vi "Text control 2 v7.2_pump-specific.vi"() -> ()   [LabVIEW 2019]
panel:
  in  "Tab Control":enum32{"Main", "Other parameters"}(tab)
  out "Vp vs time (FPP Bias Stress)":cluster{"Y data in":dbl[], "X data in":dbl[]}[](graph)
  out "Line running":i32
  out "Total lines":i32
  out "Path":path=path "C:/users/rlp38/09Apr2009LTtesting/test2.txt"
  out "I vs Vg":cluster{"Y data in":dbl[], "X data in":dbl[]}[](graph)
  out "Is max":dbl format="%.2e"
  out "Id max":dbl format="%.2e"
  out "Ig max":dbl format="%.2e"
  out "Imax vs time":cluster{"Y data in":dbl[], "X data in":dbl[]}[](graph)
  out "Imin vs time":cluster{"Y data in":dbl[], "X data in":dbl[]}[](graph)
  out "I vs Vd":cluster{"Y data in":dbl[], "X data in":dbl[]}[](graph)
  in  "Script":string="#-------------------------------------------------------\n# SPM pump cleaning script x 10\n#\n# Version: 0.5\n# Author: Dimitrios Simatos\n# Last updated: 2020-09-03\n#-------------------------------------------------------\n# Description\n#\n# This script is designed to run the cleaning sequence of the SPM OEM pump ten times.\n#-------------------------------------------------------\n# Changes\n#\n# Placed initialization and hard stop commands in the beginning.\n#-------------------------------------------------------\n# Important points\n#\n# Never leave any liquid in the pump to dry after the experiments. If they dry, the residue may block the valve.\n# Always run the cleaning cycle after the experiments.\n# Use clockwise rotation when going up in valve port numbers and vice versa.\n#-------------------------------------------------------\n# Things to do before running the script\n#\n# Remove all reservoirs, except the one in Port 3.\n# Set filenames.\n# Replace the tubing, if necessary.\n#-------------------------------------------------------\n# Port connections\n#\n# Port 1: Waste\n# Port 2: Waste\n# Port 3: Various cleaning liquids\n# Port 4: Waste\n# Port 5: Waste\n# Port 6: Waste\n#\n# Between each of the 4 runs, the settings of Port 3 will change, according to the cleaning protocol.\n# The settings for Port 3 are:\n# 1st run: 1% v/v solution of sodium hypochlorite in ultrapure water\n# 2nd run: 0.1% w/v solution of sodium dodecyl sulfate in ultrapure water\n# 3rd run: Ultrapure water\n# 4th run: Waste (in air, not immersed in liquid)\n#-------------------------------------------------------\n# Cleaning protocol for the SPM OEM pump (from the manual)\n#\n# A cleaning procedure should be performed at the end of each day or in between two different experiments.\n# An effective cleaning can be performed in the following manner:\n# • Bleach solution to kill microorganisms\n# 1. Prepare a solution of 1% chlorine bleach and deionized water\n#    NOTE: Prepare a 1% v/v solution of sodium hypochlorite in deionized water\n# 2. Prepare a reservoir and place 1 tubing in the bleach solution and 5 tubings in a waste recipient\n# 3. Pick up the bleach solution through 1 port to entirely fill the syringe\n# 4. Sequentially output the syringe content through the remaining ports and throw it to the waste\n# 5. Repeat operation at least 2 times\n# • Detergent solution to remove debris\n# 1. Prepare a solution of 0.1% detergent and deionized water\n#    NOTE: Prepare a 0.1% w/v solution of sodium dodecyl sulfate in deionized water\n# 2. Move the tubing from the bleach solution reservoir and place it into a reservoir of detergent solution\n# 3. Pick up the detergent solution through 1 port to entirely fill the syringe\n# 4. Sequentially output the detergent solution through the remaining ports into the waste recipient\n# 5. Repeat operation at least 2 times\n# • Rinsing water to prepare the pump for your next experiment\n# 1. Move the tubing from the detergent solution reservoir and place it into a reservoir of deionized water\n# 2. Pick up the rinsing solution through 1 port to entirely fill the syringe\n# 3. Sequentially output the rinse water through the remaining ports into the waste recipient\n# 4. Repeat operation at least 2 times\n# • Replace the tubing, if necessary\n#-------------------------------------------------------\n# Pumping cycles and execution time\n#\n# Execution time for a single cycle: 6 x (1 min + 10 sec) = 7 minutes\n# Total execution time: 4 x 7 = 28 minutes\n# Since the script has to run 4 times, the cleaning lasts for: 4 x 28 = 112 minutes\n# Air must be the last to be pumped through the valve, to remove all liquids.\n# There are 4 pumping cycles. Each one draws a different liquid through port 3 and pumps it sequentially through ports 1,2,4,5,6.\n# During the sequential pumping, each port receives 200 ul of liquid (20% of the total syringe volume = 600 \"plunger units\")\n# The device must be disconnected from the port during the cleaning procedure.\n# All cycles are similar, except cycle 1 has the initialization command uncommented and the first report valve command commented.\n#-------------------------------------------------------\n# Volume of liquid needed\n#\n# Volume of liquid needed per cycle: 1 ml\n# Total volume of liquid needed per script run: 4 x 1 = 4 ml\n# Since the script has to run 4 times, the first 3 with different liquids, I need:\n# 4 ml of 1% v/v solution of sodium hypochlorite in ultrapure water\n# 4 ml of 0.1% w/v solution of sodium dodecyl sulfate in ultrapure water\n# 4 ml of ultrapure water\n#-------------------------------------------------------\n# Parameters\n#\n# Syringe size: 1 ml\n# Step resolution N = 0.01 mm\n# Drawing flow V = 300 pulses/second (6000 ul/min)\n# Pumping flow V = 300 pulses/second (6000 ul/min)\n#-------------------------------------------------------\n# Pump initialization\npump /1T #hard stop pump\npump /1ZR #initialize pump\n#-------------------------------------------------------\n# Cycle 1\n# Fill the syringe\npump /1Q #query pump\npump /1? #report absolute plunger position\n#pump /1?6 #report valve position\nwait-min 1 #wait 1 minute\npump /1N0R #set step resolution: 0.01 mm\npump /1Q #query pump\npump /1? #report absolute plunger position (the plunger should be at 0)\npump /1?6 #report valve position\nwait 1000 #wait 1 second\npump /1V300R #choose speed: 300 steps/s (6000 ul/min)\npump /1Q #query pump\nwait 1000 #wait 1 second\npump /1I3R #go to port 3, clockwise rotation\npump /1Q #query pump\npump /1?6 #report valve position\nwait 1000 #wait 1 second\npump /1A3000R #go to absolute position 3000 (= draw 1 ml)\nwait 30000 #wait 30 seconds\npump /1Q #query pump\npump /1? #report absolute plunger position (the plunger should have finished moving)\n#pump /1?6 #report valve position\n# The sequential pumping begins\n# Port 1\npump /1O1R #switch to port 1, counterclockwise rotation\npump /1Q #query pump\npump /1?6 #report valve position\npump /1A2400R #go to absolute position 2400 (= pump 200 ul)\npump /1Q #query pump\npump /1? #report absolute plunger position (the plunger should be moving to 0)\nwait-min 1 #wait 1 minute\npump /1? #report absolute plunger position (the plunger should have finished moving)\n# Port 2\npump /1I2R #switch to port 2, clockwise rotation\npump /1Q #query pump\npump /1?6 #report valve position\npump /1A1800R #go to absolute position 1800 (= pump 200 ul)\npump /1Q #query pump\npump /1? #report absolute plunger position (the plunger should be moving to 0)\nwait-min 1 #wait 1 minute\npump /1? #report absolute plunger position (the plunger should have finished moving)\n# Port 4\npump /1I4R #switch to port 4, clockwise rotation\npump /1Q #query pump\npump /1?6 #report valve position\npump /1A1200R #go to absolute position 1200 (= pump 200 ul)\npump /1Q #query pump\npump /1? #report absolute plunger position (the plunger should be moving to 0)\nwait-min 1 #wait 1 minute\npump /1? #report absolute plunger position (the plunger should have finished moving)\n# Port 5\npump /1I5R #switch to port 5, clockwise rotation\npump /1Q #query pump\npump /1?6 #report valve position\npump /1A600R #go to absolute position 600 (= pump 200 ul)\npump /1Q #query pump\npump /1? #report absolute plunger position (the plunger should be moving to 0)\nwait-min 1 #wait 1 minute\npump /1? #report absolute plunger position (the plunger should have finished moving)\n# Port 6\npump /1I6R #switch to port 6, clockwise rotation\npump /1Q #query pump\npump /1?6 #report valve position\npump /1A0R #go to absolute position 0 (= pump 200 ul)\npump /1Q #query pump\npump /1? #report absolute plunger position (the plunger should be moving to 0)\nwait-min 1 #wait 1 minute\npump /1? #report absolute plunger position (the plunger should have finished moving)\n#-------------------------------------------------------\n# Cycle 2\n# Fill the syringe\n#pump /1ZR #initialize pump\npump /1Q #query pump\npump /1? #report absolute plunger position\npump /1?6 #report valve position\nwait-min 1 #wait 1 minute\npump /1N0R #set step resolution: 0.01 mm\npump /1Q #query pump\npump /1? #report absolute plunger position (the plunger should be at 0)\npump /1?6 #report valve position\nwait 1000 #wait 1 second\npump /1V300R #choose speed: 300 steps/s (6000 ul/min)\npump /1Q #query pump\nwait 1000 #wait 1 second\npump /1O3R #go to port 3, counterclockwise rotation\npump /1Q #query pump\npump /1?6 #report valve position\nwait 1000 #wait 1 second\npump /1A3000R #go to absolute position 3000 (= draw 1 ml)\nwait 30000 #wait 30 seconds\npump /1Q #query pump\npump /1? #report absolute plunger position (the plunger should have finished moving)\n#pump /1?6 #report valve position\n# The sequential pumping begins\n# Port 1\npump /1O1R #switch to port 1, counterclockwise rotation\npump /1Q #query pump\npump /1?6 #report valve position\npump /1A2400R #go to absolute position 2400 (= pump 200 ul)\npump /1Q #query pump\npump /1? #report absolute plunger position (the plunger should be moving to 0)\nwait-min 1 #wait 1 minute\npump /1? #report absolute plunger position (the plunger should have finished moving)\n# Port 2\npump /1I2R #switch to port 2, clockwise rotation\npump /1Q #query pump\npump /1?6 #report valve position\npump /1A1800R #go to absolute position 1800 (= pump 200 ul)\npump /1Q #query pump\npump /1? #report absolute plunger position (the plunger should be moving to 0)\nwait-min 1 #wait 1 minute\npump /1? #report absolute plunger position (the plunger should have finished moving)\n# Port 4\npump /1I4R #switch to port 4, clockwise rotation\npump /1Q #query pump\npump /1?6 #report valve position\npump /1A1200R #go to absolute position 1200 (= pump 200 ul)\npump /1Q #query pump\npump /1? #report absolute plunger position (the plunger should be moving to 0)\nwait-min 1 #wait 1 minute\npump /1? #report absolute plunger position (the plunger should have finished moving)\n# Port 5\npump /1I5R #switch to port 5, clockwise rotation\npump /1Q #query pump\npump /1?6 #report valve position\npump /1A600R #go to absolute position 600 (= pump 200 ul)\npump /1Q #query pump\npump /1? #report absolute plunger position (the plunger should be moving to 0)\nwait-min 1 #wait 1 minute\npump /1? #report absolute plunger position (the plunger should have finished moving)\n# Port 6\npump /1I6R #switch to port 6, clockwise rotation\npump /1Q #query pump\npump /1?6 #report valve position\npump /1A0R #go to absolute position 0 (= pump 200 ul)\npump /1Q #query pump\npump /1? #report absolute plunger position (the plunger should be moving to 0)\nwait-min 1 #wait 1 minute\npump /1? #report absolute plunger position (the plunger should have finished moving)\n#-------------------------------------------------------\n# Cycle 3\n# Fill the syringe\n#pump /1ZR #initialize pump\npump /1Q #query pump\npump /1? #report absolute plunger position\npump /1?6 #report valve position\nwait-min 1 #wait 1 minute\npump /1N0R #set step resolution: 0.01 mm\npump /1Q #query pump\npump /1? #report absolute plunger position (the plunger should be at 0)\npump /1?6 #report valve position\nwait 1000 #wait 1 second\npump /1V300R #choose speed: 300 steps/s (6000 ul/min)\npump /1Q #query pump\nwait 1000 #wait 1 second\npump /1O3R #go to port 3, counterclockwise rotation\npump /1Q #query pump\npump /1?6 #report valve position\nwait 1000 #wait 1 second\npump /1A3000R #go to absolute position 3000 (= draw 1 ml)\nwait 30000 #wait 30 seconds\npump /1Q #query pump\npump /1? #report absolute plunger position (the plunger should have finished moving)\n#pump /1?6 #report valve position\n# The sequential pumping begins\n# Port 1\npump /1O1R #switch to port 1, counterclockwise rotation\npump /1Q #query pump\npump /1?6 #report valve position\npump /1A2400R #go to absolute position 2400 (= pump 200 ul)\npump /1Q #query pump\npump /1? #report absolute plunger position (the plunger should be moving to 0)\nwait-min 1 #wait 1 minute\npump /1? #report absolute plunger position (the plunger should have finished moving)\n# Port 2\npump /1I2R #switch to port 2, clockwise rotation\npump /1Q #query pump\npump /1?6 #report valve position\npump /1A1800R #go to absolute position 1800 (= pump 200 ul)\npump /1Q #query pump\npump /1? #report absolute plunger position (the plunger should be moving to 0)\nwait-min 1 #wait 1 minute\npump /1? #report absolute plunger position (the plunger should have finished moving)\n# Port 4\npump /1I4R #switch to port 4, clockwise rotation\npump /1Q #query pump\npump /1?6 #report valve position\npump /1A1200R #go to absolute position 1200 (= pump 200 ul)\npump /1Q #query pump\npump /1? #report absolute plunger position (the plunger should be moving to 0)\nwait-min 1 #wait 1 minute\npump /1? #report absolute plunger position (the plunger should have finished moving)\n# Port 5\npump /1I5R #switch to port 5, clockwise rotation\npump /1Q #query pump\npump /1?6 #report valve position\npump /1A600R #go to absolute position 600 (= pump 200 ul)\npump /1Q #query pump\npump /1? #report absolute plunger position (the plunger should be moving to 0)\nwait-min 1 #wait 1 minute\npump /1? #report absolute plunger position (the plunger should have finished moving)\n# Port 6\npump /1I6R #switch to port 6, clockwise rotation\npump /1Q #query pump\npump /1?6 #report valve position\npump /1A0R #go to absolute position 0 (= pump 200 ul)\npump /1Q #query pump\npump /1? #report absolute plunger position (the plunger should be moving to 0)\nwait-min 1 #wait 1 minute\npump /1? #report absolute plunger position (the plunger should have finished moving)\n#-------------------------------------------------------\n# Cycle 4\n# Fill the syringe\n#pump /1ZR #initialize pump\npump /1Q #query pump\npump /1? #report absolute plunger position\npump /1?6 #report valve position\nwait-min 1 #wait 1 minute\npump /1N0R #set step resolution: 0.01 mm\npump /1Q #query pump\npump /1? #report absolute plunger position (the plunger should be at 0)\npump /1?6 #report valve position\nwait 1000 #wait 1 second\npump /1V300R #choose speed: 300 steps/s (6000 ul/min)\npump /1Q #query pump\nwait 1000 #wait 1 second\npump /1O3R #go to port 3, counterclockwise rotation\npump /1Q #query pump\npump /1?6 #report valve position\nwait 1000 #wait 1 second\npump /1A3000R #go to absolute position 3000 (= draw 1 ml)\nwait 30000 #wait 30 seconds\npump /1Q #query pump\npump /1? #report absolute plunger position (the plunger should have finished moving)\n#pump /1?6 #report valve position\n# The sequential pumping begins\n# Port 1\npump /1O1R #switch to port 1, counterclockwise rotation\npump /1Q #query pump\npump /1?6 #report valve position\npump /1A2400R #go to absolute position 2400 (= pump 200 ul)\npump /1Q #query pump\npump /1? #report absolute plunger position (the plunger should be moving to 0)\nwait-min 1 #wait 1 minute\npump /1? #report absolute plunger position (the plunger should have finished moving)\n# Port 2\npump /1I2R #switch to port 2, clockwise rotation\npump /1Q #query pump\npump /1?6 #report valve position\npump /1A1800R #go to absolute position 1800 (= pump 200 ul)\npump /1Q #query pump\npump /1? #report absolute plunger position (the plunger should be moving to 0)\nwait-min 1 #wait 1 minute\npump /1? #report absolute plunger position (the plunger should have finished moving)\n# Port 4\npump /1I4R #switch to port 4, clockwise rotation\npump /1Q #query pump\npump /1?6 #report valve position\npump /1A1200R #go to absolute position 1200 (= pump 200 ul)\npump /1Q #query pump\npump /1? #report absolute plunger position (the plunger should be moving to 0)\nwait-min 1 #wait 1 minute\npump /1? #report absolute plunger position (the plunger should have finished moving)\n# Port 5\npump /1I5R #switch to port 5, clockwise rotation\npump /1Q #query pump\npump /1?6 #report valve position\npump /1A600R #go to absolute position 600 (= pump 200 ul)\npump /1Q #query pump\npump /1? #report absolute plunger position (the plunger should be moving to 0)\nwait-min 1 #wait 1 minute\npump /1? #report absolute plunger position (the plunger should have finished moving)\n# Port 6\npump /1I6R #switch to port 6, clockwise rotation\npump /1Q #query pump\npump /1?6 #report valve position\npump /1A0R #go to absolute position 0 (= pump 200 ul)\npump /1Q #query pump\npump /1? #report absolute plunger position (the plunger should be moving to 0)\nwait-min 1 #wait 1 minute\npump /1? #report absolute plunger position (the plunger should have finished moving)\n#-------------------------------------------------------\n# Cycle 5\n# Fill the syringe\npump /1Q #query pump\npump /1? #report absolute plunger position\n#pump /1?6 #report valve position\nwait-min 1 #wait 1 minute\npump /1N0R #set step resolution: 0.01 mm\npump /1Q #query pump\npump /1? #report absolute plunger position (the plunger should be at 0)\npump /1?6 #report valve position\nwait 1000 #wait 1 second\npump /1V300R #choose speed: 300 steps/s (6000 ul/min)\npump /1Q #query pump\nwait 1000 #wait 1 second\npump /1I3R #go to port 3, clockwise rotation\npump /1Q #query pump\npump /1?6 #report valve position\nwait 1000 #wait 1 second\npump /1A3000R #go to absolute position 3000 (= draw 1 ml)\nwait 30000 #wait 30 seconds\npump /1Q #query pump\npump /1? #report absolute plunger position (the plunger should have finished moving)\n#pump /1?6 #report valve position\n# The sequential pumping begins\n# Port 1\npump /1O1R #switch to port 1, counterclockwise rotation\npump /1Q #query pump\npump /1?6 #report valve position\npump /1A2400R #go to absolute position 2400 (= pump 200 ul)\npump /1Q #query pump\npump /1? #report absolute plunger position (the plunger should be moving to 0)\nwait-min 1 #wait 1 minute\npump /1? #report absolute plunger position (the plunger should have finished moving)\n# Port 2\npump /1I2R #switch to port 2, clockwise rotation\npump /1Q #query pump\npump /1?6 #report valve position\npump /1A1800R #go to absolute position 1800 (= pump 200 ul)\npump /1Q #query pump\npump /1? #report absolute plunger position (the plunger should be moving to 0)\nwait-min 1 #wait 1 minute\npump /1? #report absolute plunger position (the plunger should have finished moving)\n# Port 4\npump /1I4R #switch to port 4, clockwise rotation\npump /1Q #query pump\npump /1?6 #report valve position\npump /1A1200R #go to absolute position 1200 (= pump 200 ul)\npump /1Q #query pump\npump /1? #report absolute plunger position (the plunger should be moving to 0)\nwait-min 1 #wait 1 minute\npump /1? #report absolute plunger position (the plunger should have finished moving)\n# Port 5\npump /1I5R #switch to port 5, clockwise rotation\npump /1Q #query pump\npump /1?6 #report valve position\npump /1A600R #go to absolute position 600 (= pump 200 ul)\npump /1Q #query pump\npump /1? #report absolute plunger position (the plunger should be moving to 0)\nwait-min 1 #wait 1 minute\npump /1? #report absolute plunger position (the plunger should have finished moving)\n# Port 6\npump /1I6R #switch to port 6, clockwise rotation\npump /1Q #query pump\npump /1?6 #report valve position\npump /1A0R #go to absolute position 0 (= pump 200 ul)\npump /1Q #query pump\npump /1? #report absolute plunger position (the plunger should be moving to 0)\nwait-min 1 #wait 1 minute\npump /1? #report absolute plunger position (the plunger should have finished moving)\n#-------------------------------------------------------\n# Cycle 6\n# Fill the syringe\n#pump /1ZR #initialize pump\npump /1Q #query pump\npump /1? #report absolute plunger position\npump /1?6 #report valve position\nwait-min 1 #wait 1 minute\npump /1N0R #set step resolution: 0.01 mm\npump /1Q #query pump\npump /1? #report absolute plunger position (the plunger should be at 0)\npump /1?6 #report valve position\nwait 1000 #wait 1 second\npump /1V300R #choose speed: 300 steps/s (6000 ul/min)\npump /1Q #query pump\nwait 1000 #wait 1 second\npump /1O3R #go to port 3, counterclockwise rotation\npump /1Q #query pump\npump /1?6 #report valve position\nwait 1000 #wait 1 second\npump /1A3000R #go to absolute position 3000 (= draw 1 ml)\nwait 30000 #wait 30 seconds\npump /1Q #query pump\npump /1? #report absolute plunger position (the plunger should have finished moving)\n#pump /1?6 #report valve position\n# The sequential pumping begins\n# Port 1\npump /1O1R #switch to port 1, counterclockwise rotation\npump /1Q #query pump\npump /1?6 #report valve position\npump /1A2400R #go to absolute position 2400 (= pump 200 ul)\npump /1Q #query pump\npump /1? #report absolute plunger position (the plunger should be moving to 0)\nwait-min 1 #wait 1 minute\npump /1? #report absolute plunger position (the plunger should have finished moving)\n# Port 2\npump /1I2R #switch to port 2, clockwise rotation\npump /1Q #query pump\npump /1?6 #report valve position\npump /1A1800R #go to absolute position 1800 (= pump 200 ul)\npump /1Q #query pump\npump /1? #report absolute plunger position (the plunger should be moving to 0)\nwait-min 1 #wait 1 minute\npump /1? #report absolute plunger position (the plunger should have finished moving)\n# Port 4\npump /1I4R #switch to port 4, clockwise rotation\npump /1Q #query pump\npump /1?6 #report valve position\npump /1A1200R #go to absolute position 1200 (= pump 200 ul)\npump /1Q #query pump\npump /1? #report absolute plunger position (the plunger should be moving to 0)\nwait-min 1 #wait 1 minute\npump /1? #report absolute plunger position (the plunger should have finished moving)\n# Port 5\npump /1I5R #switch to port 5, clockwise rotation\npump /1Q #query pump\npump /1?6 #report valve position\npump /1A600R #go to absolute position 600 (= pump 200 ul)\npump /1Q #query pump\npump /1? #report absolute plunger position (the plunger should be moving to 0)\nwait-min 1 #wait 1 minute\npump /1? #report absolute plunger position (the plunger should have finished moving)\n# Port 6\npump /1I6R #switch to port 6, clockwise rotation\npump /1Q #query pump\npump /1?6 #report valve position\npump /1A0R #go to absolute position 0 (= pump 200 ul)\npump /1Q #query pump\npump /1? #report absolute plunger position (the plunger should be moving to 0)\nwait-min 1 #wait 1 minute\npump /1? #report absolute plunger position (the plunger should have finished moving)\n#-------------------------------------------------------\n# Cycle 7\n# Fill the syringe\n#pump /1ZR #initialize pump\npump /1Q #query pump\npump /1? #report absolute plunger position\npump /1?6 #report valve position\nwait-min 1 #wait 1 minute\npump /1N0R #set step resolution: 0.01 mm\npump /1Q #query pump\npump /1? #report absolute plunger position (the plunger should be at 0)\npump /1?6 #report valve position\nwait 1000 #wait 1 second\npump /1V300R #choose speed: 300 steps/s (6000 ul/min)\npump /1Q #query pump\nwait 1000 #wait 1 second\npump /1O3R #go to port 3, counterclockwise rotation\npump /1Q #query pump\npump /1?6 #report valve position\nwait 1000 #wait 1 second\npump /1A3000R #go to absolute position 3000 (= draw 1 ml)\nwait 30000 #wait 30 seconds\npump /1Q #query pump\npump /1? #report absolute plunger position (the plunger should have finished moving)\n#pump /1?6 #report valve position\n# The sequential pumping begins\n# Port 1\npump /1O1R #switch to port 1, counterclockwise rotation\npump /1Q #query pump\npump /1?6 #report valve position\npump /1A2400R #go to absolute position 2400 (= pump 200 ul)\npump /1Q #query pump\npump /1? #report absolute plunger position (the plunger should be moving to 0)\nwait-min 1 #wait 1 minute\npump /1? #report absolute plunger position (the plunger should have finished moving)\n# Port 2\npump /1I2R #switch to port 2, clockwise rotation\npump /1Q #query pump\npump /1?6 #report valve position\npump /1A1800R #go to absolute position 1800 (= pump 200 ul)\npump /1Q #query pump\npump /1? #report absolute plunger position (the plunger should be moving to 0)\nwait-min 1 #wait 1 minute\npump /1? #report absolute plunger position (the plunger should have finished moving)\n# Port 4\npump /1I4R #switch to port 4, clockwise rotation\npump /1Q #query pump\npump /1?6 #report valve position\npump /1A1200R #go to absolute position 1200 (= pump 200 ul)\npump /1Q #query pump\npump /1? #report absolute plunger position (the plunger should be moving to 0)\nwait-min 1 #wait 1 minute\npump /1? #report absolute plunger position (the plunger should have finished moving)\n# Port 5\npump /1I5R #switch to port 5, clockwise rotation\npump /1Q #query pump\npump /1?6 #report valve position\npump /1A600R #go to absolute position 600 (= pump 200 ul)\npump /1Q #query pump\npump /1? #report absolute plunger position (the plunger should be moving to 0)\nwait-min 1 #wait 1 minute\npump /1? #report absolute plunger position (the plunger should have finished moving)\n# Port 6\npump /1I6R #switch to port 6, clockwise rotation\npump /1Q #query pump\npump /1?6 #report valve position\npump /1A0R #go to absolute position 0 (= pump 200 ul)\npump /1Q #query pump\npump /1? #report absolute plunger position (the plunger should be moving to 0)\nwait-min 1 #wait 1 minute\npump /1? #report absolute plunger position (the plunger should have finished moving)\n#-------------------------------------------------------\n# Cycle 8\n# Fill the syringe\n#pump /1ZR #initialize pump\npump /1Q #query pump\npump /1? #report absolute plunger position\npump /1?6 #report valve position\nwait-min 1 #wait 1 minute\npump /1N0R #set step resolution: 0.01 mm\npump /1Q #query pump\npump /1? #report absolute plunger position (the plunger should be at 0)\npump /1?6 #report valve position\nwait 1000 #wait 1 second\npump /1V300R #choose speed: 300 steps/s (6000 ul/min)\npump /1Q #query pump\nwait 1000 #wait 1 second\npump /1O3R #go to port 3, counterclockwise rotation\npump /1Q #query pump\npump /1?6 #report valve position\nwait 1000 #wait 1 second\npump /1A3000R #go to absolute position 3000 (= draw 1 ml)\nwait 30000 #wait 30 seconds\npump /1Q #query pump\npump /1? #report absolute plunger position (the plunger should have finished moving)\n#pump /1?6 #report valve position\n# The sequential pumping begins\n# Port 1\npump /1O1R #switch to port 1, counterclockwise rotation\npump /1Q #query pump\npump /1?6 #report valve position\npump /1A2400R #go to absolute position 2400 (= pump 200 ul)\npump /1Q #query pump\npump /1? #report absolute plunger position (the plunger should be moving to 0)\nwait-min 1 #wait 1 minute\npump /1? #report absolute plunger position (the plunger should have finished moving)\n# Port 2\npump /1I2R #switch to port 2, clockwise rotation\npump /1Q #query pump\npump /1?6 #report valve position\npump /1A1800R #go to absolute position 1800 (= pump 200 ul)\npump /1Q #query pump\npump /1? #report absolute plunger position (the plunger should be moving to 0)\nwait-min 1 #wait 1 minute\npump /1? #report absolute plunger position (the plunger should have finished moving)\n# Port 4\npump /1I4R #switch to port 4, clockwise rotation\npump /1Q #query pump\npump /1?6 #report valve position\npump /1A1200R #go to absolute position 1200 (= pump 200 ul)\npump /1Q #query pump\npump /1? #report absolute plunger position (the plunger should be moving to 0)\nwait-min 1 #wait 1 minute\npump /1? #report absolute plunger position (the plunger should have finished moving)\n# Port 5\npump /1I5R #switch to port 5, clockwise rotation\npump /1Q #query pump\npump /1?6 #report valve position\npump /1A600R #go to absolute position 600 (= pump 200 ul)\npump /1Q #query pump\npump /1? #report absolute plunger position (the plunger should be moving to 0)\nwait-min 1 #wait 1 minute\npump /1? #report absolute plunger position (the plunger should have finished moving)\n# Port 6\npump /1I6R #switch to port 6, clockwise rotation\npump /1Q #query pump\npump /1?6 #report valve position\npump /1A0R #go to absolute position 0 (= pump 200 ul)\npump /1Q #query pump\npump /1? #report absolute plunger position (the plunger should be moving to 0)\nwait-min 1 #wait 1 minute\npump /1? #report absolute plunger position (the plunger should have finished moving)\n#-------------------------------------------------------\n# Cycle 9\n# Fill the syringe\npump /1Q #query pump\npump /1? #report absolute plunger position\n#pump /1?6 #report valve position\nwait-min 1 #wait 1 minute\npump /1N0R #set step resolution: 0.01 mm\npump /1Q #query pump\npump /1? #report absolute plunger position (the plunger should be at 0)\npump /1?6 #report valve position\nwait 1000 #wait 1 second\npump /1V300R #choose speed: 300 steps/s (6000 ul/min)\npump /1Q #query pump\nwait 1000 #wait 1 second\npump /1I3R #go to port 3, clockwise rotation\npump /1Q #query pump\npump /1?6 #report valve position\nwait 1000 #wait 1 second\npump /1A3000R #go to absolute position 3000 (= draw 1 ml)\nwait 30000 #wait 30 seconds\npump /1Q #query pump\npump /1? #report absolute plunger position (the plunger should have finished moving)\n#pump /1?6 #report valve position\n# The sequential pumping begins\n# Port 1\npump /1O1R #switch to port 1, counterclockwise rotation\npump /1Q #query pump\npump /1?6 #report valve position\npump /1A2400R #go to absolute position 2400 (= pump 200 ul)\npump /1Q #query pump\npump /1? #report absolute plunger position (the plunger should be moving to 0)\nwait-min 1 #wait 1 minute\npump /1? #report absolute plunger position (the plunger should have finished moving)\n# Port 2\npump /1I2R #switch to port 2, clockwise rotation\npump /1Q #query pump\npump /1?6 #report valve position\npump /1A1800R #go to absolute position 1800 (= pump 200 ul)\npump /1Q #query pump\npump /1? #report absolute plunger position (the plunger should be moving to 0)\nwait-min 1 #wait 1 minute\npump /1? #report absolute plunger position (the plunger should have finished moving)\n# Port 4\npump /1I4R #switch to port 4, clockwise rotation\npump /1Q #query pump\npump /1?6 #report valve position\npump /1A1200R #go to absolute position 1200 (= pump 200 ul)\npump /1Q #query pump\npump /1? #report absolute plunger position (the plunger should be moving to 0)\nwait-min 1 #wait 1 minute\npump /1? #report absolute plunger position (the plunger should have finished moving)\n# Port 5\npump /1I5R #switch to port 5, clockwise rotation\npump /1Q #query pump\npump /1?6 #report valve position\npump /1A600R #go to absolute position 600 (= pump 200 ul)\npump /1Q #query pump\npump /1? #report absolute plunger position (the plunger should be moving to 0)\nwait-min 1 #wait 1 minute\npump /1? #report absolute plunger position (the plunger should have finished moving)\n# Port 6\npump /1I6R #switch to port 6, clockwise rotation\npump /1Q #query pump\npump /1?6 #report valve position\npump /1A0R #go to absolute position 0 (= pump 200 ul)\npump /1Q #query pump\npump /1? #report absolute plunger position (the plunger should be moving to 0)\nwait-min 1 #wait 1 minute\npump /1? #report absolute plunger position (the plunger should have finished moving)\n#-------------------------------------------------------\n# Cycle 10\n# Fill the syringe\n#pump /1ZR #initialize pump\npump /1Q #query pump\npump /1? #report absolute plunger position\npump /1?6 #report valve position\nwait-min 1 #wait 1 minute\npump /1N0R #set step resolution: 0.01 mm\npump /1Q #query pump\npump /1? #report absolute plunger position (the plunger should be at 0)\npump /1?6 #report valve position\nwait 1000 #wait 1 second\npump /1V300R #choose speed: 300 steps/s (6000 ul/min)\npump /1Q #query pump\nwait 1000 #wait 1 second\npump /1O3R #go to port 3, counterclockwise rotation\npump /1Q #query pump\npump /1?6 #report valve position\nwait 1000 #wait 1 second\npump /1A3000R #go to absolute position 3000 (= draw 1 ml)\nwait 30000 #wait 30 seconds\npump /1Q #query pump\npump /1? #report absolute plunger position (the plunger should have finished moving)\n#pump /1?6 #report valve position\n# The sequential pumping begins\n# Port 1\npump /1O1R #switch to port 1, counterclockwise rotation\npump /1Q #query pump\npump /1?6 #report valve position\npump /1A2400R #go to absolute position 2400 (= pump 200 ul)\npump /1Q #query pump\npump /1? #report absolute plunger position (the plunger should be moving to 0)\nwait-min 1 #wait 1 minute\npump /1? #report absolute plunger position (the plunger should have finished moving)\n# Port 2\npump /1I2R #switch to port 2, clockwise rotation\npump /1Q #query pump\npump /1?6 #report valve position\npump /1A1800R #go to absolute position 1800 (= pump 200 ul)\npump /1Q #query pump\npump /1? #report absolute plunger position (the plunger should be moving to 0)\nwait-min 1 #wait 1 minute\npump /1? #report absolute plunger position (the plunger should have finished moving)\n# Port 4\npump /1I4R #switch to port 4, clockwise rotation\npump /1Q #query pump\npump /1?6 #report valve position\npump /1A1200R #go to absolute position 1200 (= pump 200 ul)\npump /1Q #query pump\npump /1? #report absolute plunger position (the plunger should be moving to 0)\nwait-min 1 #wait 1 minute\npump /1? #report absolute plunger position (the plunger should have finished moving)\n# Port 5\npump /1I5R #switch to port 5, clockwise rotation\npump /1Q #query pump\npump /1?6 #report valve position\npump /1A600R #go to absolute position 600 (= pump 200 ul)\npump /1Q #query pump\npump /1? #report absolute plunger position (the plunger should be moving to 0)\nwait-min 1 #wait 1 minute\npump /1? #report absolute plunger position (the plunger should have finished moving)\n# Port 6\npump /1I6R #switch to port 6, clockwise rotation\npump /1Q #query pump\npump /1?6 #report valve position\npump /1A0R #go to absolute position 0 (= pump 200 ul)\npump /1Q #query pump\npump /1? #report absolute plunger position (the plunger should be moving to 0)\nwait-min 1 #wait 1 minute\npump /1? #report absolute plunger position (the plunger should have finished moving)\n#-------------------------------------------------------\n# Cycle 11\n# Fill the syringe\n#pump /1ZR #initialize pump\npump /1Q #query pump\npump /1? #report absolute plunger position\npump /1?6 #report valve position\nwait-min 1 #wait 1 minute\npump /1N0R #set step resolution: 0.01 mm\npump /1Q #query pump\npump /1? #report absolute plunger position (the plunger should be at 0)\npump /1?6 #report valve position\nwait 1000 #wait 1 second\npump /1V300R #choose speed: 300 steps/s (6000 ul/min)\npump /1Q #query pump\nwait 1000 #wait 1 second\npump /1O3R #go to port 3, counterclockwise rotation\npump /1Q #query pump\npump /1?6 #report valve position\nwait 1000 #wait 1 second\npump /1A3000R #go to absolute position 3000 (= draw 1 ml)\nwait 30000 #wait 30 seconds\npump /1Q #query pump\npump /1? #report absolute plunger position (the plunger should have finished moving)\n#pump /1?6 #report valve position\n# The sequential pumping begins\n# Port 1\npump /1O1R #switch to port 1, counterclockwise rotation\npump /1Q #query pump\npump /1?6 #report valve position\npump /1A2400R #go to absolute position 2400 (= pump 200 ul)\npump /1Q #query pump\npump /1? #report absolute plunger position (the plunger should be moving to 0)\nwait-min 1 #wait 1 minute\npump /1? #report absolute plunger position (the plunger should have finished moving)\n# Port 2\npump /1I2R #switch to port 2, clockwise rotation\npump /1Q #query pump\npump /1?6 #report valve position\npump /1A1800R #go to absolute position 1800 (= pump 200 ul)\npump /1Q #query pump\npump /1? #report absolute plunger position (the plunger should be moving to 0)\nwait-min 1 #wait 1 minute\npump /1? #report absolute plunger position (the plunger should have finished moving)\n# Port 4\npump /1I4R #switch to port 4, clockwise rotation\npump /1Q #query pump\npump /1?6 #report valve position\npump /1A1200R #go to absolute position 1200 (= pump 200 ul)\npump /1Q #query pump\npump /1? #report absolute plunger position (the plunger should be moving to 0)\nwait-min 1 #wait 1 minute\npump /1? #report absolute plunger position (the plunger should have finished moving)\n# Port 5\npump /1I5R #switch to port 5, clockwise rotation\npump /1Q #query pump\npump /1?6 #report valve position\npump /1A600R #go to absolute position 600 (= pump 200 ul)\npump /1Q #query pump\npump /1? #report absolute plunger position (the plunger should be moving to 0)\nwait-min 1 #wait 1 minute\npump /1? #report absolute plunger position (the plunger should have finished moving)\n# Port 6\npump /1I6R #switch to port 6, clockwise rotation\npump /1Q #query pump\npump /1?6 #report valve position\npump /1A0R #go to absolute position 0 (= pump 200 ul)\npump /1Q #query pump\npump /1? #report absolute plunger position (the plunger should be moving to 0)\nwait-min 1 #wait 1 minute\npump /1? #report absolute plunger position (the plunger should have finished moving)\n#-------------------------------------------------------\n# Cycle 12\n# Fill the syringe\n#pump /1ZR #initialize pump\npump /1Q #query pump\npump /1? #report absolute plunger position\npump /1?6 #report valve position\nwait-min 1 #wait 1 minute\npump /1N0R #set step resolution: 0.01 mm\npump /1Q #query pump\npump /1? #report absolute plunger position (the plunger should be at 0)\npump /1?6 #report valve position\nwait 1000 #wait 1 second\npump /1V300R #choose speed: 300 steps/s (6000 ul/min)\npump /1Q #query pump\nwait 1000 #wait 1 second\npump /1O3R #go to port 3, counterclockwise rotation\npump /1Q #query pump\npump /1?6 #report valve position\nwait 1000 #wait 1 second\npump /1A3000R #go to absolute position 3000 (= draw 1 ml)\nwait 30000 #wait 30 seconds\npump /1Q #query pump\npump /1? #report absolute plunger position (the plunger should have finished moving)\n#pump /1?6 #report valve position\n# The sequential pumping begins\n# Port 1\npump /1O1R #switch to port 1, counterclockwise rotation\npump /1Q #query pump\npump /1?6 #report valve position\npump /1A2400R #go to absolute position 2400 (= pump 200 ul)\npump /1Q #query pump\npump /1? #report absolute plunger position (the plunger should be moving to 0)\nwait-min 1 #wait 1 minute\npump /1? #report absolute plunger position (the plunger should have finished moving)\n# Port 2\npump /1I2R #switch to port 2, clockwise rotation\npump /1Q #query pump\npump /1?6 #report valve position\npump /1A1800R #go to absolute position 1800 (= pump 200 ul)\npump /1Q #query pump\npump /1? #report absolute plunger position (the plunger should be moving to 0)\nwait-min 1 #wait 1 minute\npump /1? #report absolute plunger position (the plunger should have finished moving)\n# Port 4\npump /1I4R #switch to port 4, clockwise rotation\npump /1Q #query pump\npump /1?6 #report valve position\npump /1A1200R #go to absolute position 1200 (= pump 200 ul)\npump /1Q #query pump\npump /1? #report absolute plunger position (the plunger should be moving to 0)\nwait-min 1 #wait 1 minute\npump /1? #report absolute plunger position (the plunger should have finished moving)\n# Port 5\npump /1I5R #switch to port 5, clockwise rotation\npump /1Q #query pump\npump /1?6 #report valve position\npump /1A600R #go to absolute position 600 (= pump 200 ul)\npump /1Q #query pump\npump /1? #report absolute plunger position (the plunger should be moving to 0)\nwait-min 1 #wait 1 minute\npump /1? #report absolute plunger position (the plunger should have finished moving)\n# Port 6\npump /1I6R #switch to port 6, clockwise rotation\npump /1Q #query pump\npump /1?6 #report valve position\npump /1A0R #go to absolute position 0 (= pump 200 ul)\npump /1Q #query pump\npump /1? #report absolute plunger position (the plunger should be moving to 0)\nwait-min 1 #wait 1 minute\npump /1? #report absolute plunger position (the plunger should have finished moving)\n#-------------------------------------------------------\n# Cycle 13\n# Fill the syringe\npump /1Q #query pump\npump /1? #report absolute plunger position\n#pump /1?6 #report valve position\nwait-min 1 #wait 1 minute\npump /1N0R #set step resolution: 0.01 mm\npump /1Q #query pump\npump /1? #report absolute plunger position (the plunger should be at 0)\npump /1?6 #report valve position\nwait 1000 #wait 1 second\npump /1V300R #choose speed: 300 steps/s (6000 ul/min)\npump /1Q #query pump\nwait 1000 #wait 1 second\npump /1I3R #go to port 3, clockwise rotation\npump /1Q #query pump\npump /1?6 #report valve position\nwait 1000 #wait 1 second\npump /1A3000R #go to absolute position 3000 (= draw 1 ml)\nwait 30000 #wait 30 seconds\npump /1Q #query pump\npump /1? #report absolute plunger position (the plunger should have finished moving)\n#pump /1?6 #report valve position\n# The sequential pumping begins\n# Port 1\npump /1O1R #switch to port 1, counterclockwise rotation\npump /1Q #query pump\npump /1?6 #report valve position\npump /1A2400R #go to absolute position 2400 (= pump 200 ul)\npump /1Q #query pump\npump /1? #report absolute plunger position (the plunger should be moving to 0)\nwait-min 1 #wait 1 minute\npump /1? #report absolute plunger position (the plunger should have finished moving)\n# Port 2\npump /1I2R #switch to port 2, clockwise rotation\npump /1Q #query pump\npump /1?6 #report valve position\npump /1A1800R #go to absolute position 1800 (= pump 200 ul)\npump /1Q #query pump\npump /1? #report absolute plunger position (the plunger should be moving to 0)\nwait-min 1 #wait 1 minute\npump /1? #report absolute plunger position (the plunger should have finished moving)\n# Port 4\npump /1I4R #switch to port 4, clockwise rotation\npump /1Q #query pump\npump /1?6 #report valve position\npump /1A1200R #go to absolute position 1200 (= pump 200 ul)\npump /1Q #query pump\npump /1? #report absolute plunger position (the plunger should be moving to 0)\nwait-min 1 #wait 1 minute\npump /1? #report absolute plunger position (the plunger should have finished moving)\n# Port 5\npump /1I5R #switch to port 5, clockwise rotation\npump /1Q #query pump\npump /1?6 #report valve position\npump /1A600R #go to absolute position 600 (= pump 200 ul)\npump /1Q #query pump\npump /1? #report absolute plunger position (the plunger should be moving to 0)\nwait-min 1 #wait 1 minute\npump /1? #report absolute plunger position (the plunger should have finished moving)\n# Port 6\npump /1I6R #switch to port 6, clockwise rotation\npump /1Q #query pump\npump /1?6 #report valve position\npump /1A0R #go to absolute position 0 (= pump 200 ul)\npump /1Q #query pump\npump /1? #report absolute plunger position (the plunger should be moving to 0)\nwait-min 1 #wait 1 minute\npump /1? #report absolute plunger position (the plunger should have finished moving)\n#-------------------------------------------------------\n# Cycle 14\n# Fill the syringe\n#pump /1ZR #initialize pump\npump /1Q #query pump\npump /1? #report absolute plunger position\npump /1?6 #report valve position\nwait-min 1 #wait 1 minute\npump /1N0R #set step resolution: 0.01 mm\npump /1Q #query pump\npump /1? #report absolute plunger position (the plunger should be at 0)\npump /1?6 #report valve position\nwait 1000 #wait 1 second\npump /1V300R #choose speed: 300 steps/s (6000 ul/min)\npump /1Q #query pump\nwait 1000 #wait 1 second\npump /1O3R #go to port 3, counterclockwise rotation\npump /1Q #query pump\npump /1?6 #report valve position\nwait 1000 #wait 1 second\npump /1A3000R #go to absolute position 3000 (= draw 1 ml)\nwait 30000 #wait 30 seconds\npump /1Q #query pump\npump /1? #report absolute plunger position (the plunger should have finished moving)\n#pump /1?6 #report valve position\n# The sequential pumping begins\n# Port 1\npump /1O1R #switch to port 1, counterclockwise rotation\npump /1Q #query pump\npump /1?6 #report valve position\npump /1A2400R #go to absolute position 2400 (= pump 200 ul)\npump /1Q #query pump\npump /1? #report absolute plunger position (the plunger should be moving to 0)\nwait-min 1 #wait 1 minute\npump /1? #report absolute plunger position (the plunger should have finished moving)\n# Port 2\npump /1I2R #switch to port 2, clockwise rotation\npump /1Q #query pump\npump /1?6 #report valve position\npump /1A1800R #go to absolute position 1800 (= pump 200 ul)\npump /1Q #query pump\npump /1? #report absolute plunger position (the plunger should be moving to 0)\nwait-min 1 #wait 1 minute\npump /1? #report absolute plunger position (the plunger should have finished moving)\n# Port 4\npump /1I4R #switch to port 4, clockwise rotation\npump /1Q #query pump\npump /1?6 #report valve position\npump /1A1200R #go to absolute position 1200 (= pump 200 ul)\npump /1Q #query pump\npump /1? #report absolute plunger position (the plunger should be moving to 0)\nwait-min 1 #wait 1 minute\npump /1? #report absolute plunger position (the plunger should have finished moving)\n# Port 5\npump /1I5R #switch to port 5, clockwise rotation\npump /1Q #query pump\npump /1?6 #report valve position\npump /1A600R #go to absolute position 600 (= pump 200 ul)\npump /1Q #query pump\npump /1? #report absolute plunger position (the plunger should be moving to 0)\nwait-min 1 #wait 1 minute\npump /1? #report absolute plunger position (the plunger should have finished moving)\n# Port 6\npump /1I6R #switch to port 6, clockwise rotation\npump /1Q #query pump\npump /1?6 #report valve position\npump /1A0R #go to absolute position 0 (= pump 200 ul)\npump /1Q #query pump\npump /1? #report absolute plunger position (the plunger should be moving to 0)\nwait-min 1 #wait 1 minute\npump /1? #report absolute plunger position (the plunger should have finished moving)\n#-------------------------------------------------------\n# Cycle 15\n# Fill the syringe\n#pump /1ZR #initialize pump\npump /1Q #query pump\npump /1? #report absolute plunger position\npump /1?6 #report valve position\nwait-min 1 #wait 1 minute\npump /1N0R #set step resolution: 0.01 mm\npump /1Q #query pump\npump /1? #report absolute plunger position (the plunger should be at 0)\npump /1?6 #report valve position\nwait 1000 #wait 1 second\npump /1V300R #choose speed: 300 steps/s (6000 ul/min)\npump /1Q #query pump\nwait 1000 #wait 1 second\npump /1O3R #go to port 3, counterclockwise rotation\npump /1Q #query pump\npump /1?6 #report valve position\nwait 1000 #wait 1 second\npump /1A3000R #go to absolute position 3000 (= draw 1 ml)\nwait 30000 #wait 30 seconds\npump /1Q #query pump\npump /1? #report absolute plunger position (the plunger should have finished moving)\n#pump /1?6 #report valve position\n# The sequential pumping begins\n# Port 1\npump /1O1R #switch to port 1, counterclockwise rotation\npump /1Q #query pump\npump /1?6 #report valve position\npump /1A2400R #go to absolute position 2400 (= pump 200 ul)\npump /1Q #query pump\npump /1? #report absolute plunger position (the plunger should be moving to 0)\nwait-min 1 #wait 1 minute\npump /1? #report absolute plunger position (the plunger should have finished moving)\n# Port 2\npump /1I2R #switch to port 2, clockwise rotation\npump /1Q #query pump\npump /1?6 #report valve position\npump /1A1800R #go to absolute position 1800 (= pump 200 ul)\npump /1Q #query pump\npump /1? #report absolute plunger position (the plunger should be moving to 0)\nwait-min 1 #wait 1 minute\npump /1? #report absolute plunger position (the plunger should have finished moving)\n# Port 4\npump /1I4R #switch to port 4, clockwise rotation\npump /1Q #query pump\npump /1?6 #report valve position\npump /1A1200R #go to absolute position 1200 (= pump 200 ul)\npump /1Q #query pump\npump /1? #report absolute plunger position (the plunger should be moving to 0)\nwait-min 1 #wait 1 minute\npump /1? #report absolute plunger position (the plunger should have finished moving)\n# Port 5\npump /1I5R #switch to port 5, clockwise rotation\npump /1Q #query pump\npump /1?6 #report valve position\npump /1A600R #go to absolute position 600 (= pump 200 ul)\npump /1Q #query pump\npump /1? #report absolute plunger position (the plunger should be moving to 0)\nwait-min 1 #wait 1 minute\npump /1? #report absolute plunger position (the plunger should have finished moving)\n# Port 6\npump /1I6R #switch to port 6, clockwise rotation\npump /1Q #query pump\npump /1?6 #report valve position\npump /1A0R #go to absolute position 0 (= pump 200 ul)\npump /1Q #query pump\npump /1? #report absolute plunger position (the plunger should be moving to 0)\nwait-min 1 #wait 1 minute\npump /1? #report absolute plunger position (the plunger should have finished moving)\n#-------------------------------------------------------\n# Cycle 16\n# Fill the syringe\n#pump /1ZR #initialize pump\npump /1Q #query pump\npump /1? #report absolute plunger position\npump /1?6 #report valve position\nwait-min 1 #wait 1 minute\npump /1N0R #set step resolution: 0.01 mm\npump /1Q #query pump\npump /1? #report absolute plunger position (the plunger should be at 0)\npump /1?6 #report valve position\nwait 1000 #wait 1 second\npump /1V300R #choose speed: 300 steps/s (6000 ul/min)\npump /1Q #query pump\nwait 1000 #wait 1 second\npump /1O3R #go to port 3, counterclockwise rotation\npump /1Q #query pump\npump /1?6 #report valve position\nwait 1000 #wait 1 second\npump /1A3000R #go to absolute position 3000 (= draw 1 ml)\nwait 30000 #wait 30 seconds\npump /1Q #query pump\npump /1? #report absolute plunger position (the plunger should have finished moving)\n#pump /1?6 #report valve position\n# The sequential pumping begins\n# Port 1\npump /1O1R #switch to port 1, counterclockwise rotation\npump /1Q #query pump\npump /1?6 #report valve position\npump /1A2400R #go to absolute position 2400 (= pump 200 ul)\npump /1Q #query pump\npump /1? #report absolute plunger position (the plunger should be moving to 0)\nwait-min 1 #wait 1 minute\npump /1? #report absolute plunger position (the plunger should have finished moving)\n# Port 2\npump /1I2R #switch to port 2, clockwise rotation\npump /1Q #query pump\npump /1?6 #report valve position\npump /1A1800R #go to absolute position 1800 (= pump 200 ul)\npump /1Q #query pump\npump /1? #report absolute plunger position (the plunger should be moving to 0)\nwait-min 1 #wait 1 minute\npump /1? #report absolute plunger position (the plunger should have finished moving)\n# Port 4\npump /1I4R #switch to port 4, clockwise rotation\npump /1Q #query pump\npump /1?6 #report valve position\npump /1A1200R #go to absolute position 1200 (= pump 200 ul)\npump /1Q #query pump\npump /1? #report absolute plunger position (the plunger should be moving to 0)\nwait-min 1 #wait 1 minute\npump /1? #report absolute plunger position (the plunger should have finished moving)\n# Port 5\npump /1I5R #switch to port 5, clockwise rotation\npump /1Q #query pump\npump /1?6 #report valve position\npump /1A600R #go to absolute position 600 (= pump 200 ul)\npump /1Q #query pump\npump /1? #report absolute plunger position (the plunger should be moving to 0)\nwait-min 1 #wait 1 minute\npump /1? #report absolute plunger position (the plunger should have finished moving)\n# Port 6\npump /1I6R #switch to port 6, clockwise rotation\npump /1Q #query pump\npump /1?6 #report valve position\npump /1A0R #go to absolute position 0 (= pump 200 ul)\npump /1Q #query pump\npump /1? #report absolute plunger position (the plunger should be moving to 0)\nwait-min 1 #wait 1 minute\npump /1? #report absolute plunger position (the plunger should have finished moving)\n#-------------------------------------------------------\n# Cycle 17\n# Fill the syringe\npump /1Q #query pump\npump /1? #report absolute plunger position\n#pump /1?6 #report valve position\nwait-min 1 #wait 1 minute\npump /1N0R #set step resolution: 0.01 mm\npump /1Q #query pump\npump /1? #report absolute plunger position (the plunger should be at 0)\npump /1?6 #report valve position\nwait 1000 #wait 1 second\npump /1V300R #choose speed: 300 steps/s (6000 ul/min)\npump /1Q #query pump\nwait 1000 #wait 1 second\npump /1I3R #go to port 3, clockwise rotation\npump /1Q #query pump\npump /1?6 #report valve position\nwait 1000 #wait 1 second\npump /1A3000R #go to absolute position 3000 (= draw 1 ml)\nwait 30000 #wait 30 seconds\npump /1Q #query pump\npump /1? #report absolute plunger position (the plunger should have finished moving)\n#pump /1?6 #report valve position\n# The sequential pumping begins\n# Port 1\npump /1O1R #switch to port 1, counterclockwise rotation\npump /1Q #query pump\npump /1?6 #report valve position\npump /1A2400R #go to absolute position 2400 (= pump 200 ul)\npump /1Q #query pump\npump /1? #report absolute plunger position (the plunger should be moving to 0)\nwait-min 1 #wait 1 minute\npump /1? #report absolute plunger position (the plunger should have finished moving)\n# Port 2\npump /1I2R #switch to port 2, clockwise rotation\npump /1Q #query pump\npump /1?6 #report valve position\npump /1A1800R #go to absolute position 1800 (= pump 200 ul)\npump /1Q #query pump\npump /1? #report absolute plunger position (the plunger should be moving to 0)\nwait-min 1 #wait 1 minute\npump /1? #report absolute plunger position (the plunger should have finished moving)\n# Port 4\npump /1I4R #switch to port 4, clockwise rotation\npump /1Q #query pump\npump /1?6 #report valve position\npump /1A1200R #go to absolute position 1200 (= pump 200 ul)\npump /1Q #query pump\npump /1? #report absolute plunger position (the plunger should be moving to 0)\nwait-min 1 #wait 1 minute\npump /1? #report absolute plunger position (the plunger should have finished moving)\n# Port 5\npump /1I5R #switch to port 5, clockwise rotation\npump /1Q #query pump\npump /1?6 #report valve position\npump /1A600R #go to absolute position 600 (= pump 200 ul)\npump /1Q #query pump\npump /1? #report absolute plunger position (the plunger should be moving to 0)\nwait-min 1 #wait 1 minute\npump /1? #report absolute plunger position (the plunger should have finished moving)\n# Port 6\npump /1I6R #switch to port 6, clockwise rotation\npump /1Q #query pump\npump /1?6 #report valve position\npump /1A0R #go to absolute position 0 (= pump 200 ul)\npump /1Q #query pump\npump /1? #report absolute plunger position (the plunger should be moving to 0)\nwait-min 1 #wait 1 minute\npump /1? #report absolute plunger position (the plunger should have finished moving)\n#-------------------------------------------------------\n# Cycle 18\n# Fill the syringe\n#pump /1ZR #initialize pump\npump /1Q #query pump\npump /1? #report absolute plunger position\npump /1?6 #report valve position\nwait-min 1 #wait 1 minute\npump /1N0R #set step resolution: 0.01 mm\npump /1Q #query pump\npump /1? #report absolute plunger position (the plunger should be at 0)\npump /1?6 #report valve position\nwait 1000 #wait 1 second\npump /1V300R #choose speed: 300 steps/s (6000 ul/min)\npump /1Q #query pump\nwait 1000 #wait 1 second\npump /1O3R #go to port 3, counterclockwise rotation\npump /1Q #query pump\npump /1?6 #report valve position\nwait 1000 #wait 1 second\npump /1A3000R #go to absolute position 3000 (= draw 1 ml)\nwait 30000 #wait 30 seconds\npump /1Q #query pump\npump /1? #report absolute plunger position (the plunger should have finished moving)\n#pump /1?6 #report valve position\n# The sequential pumping begins\n# Port 1\npump /1O1R #switch to port 1, counterclockwise rotation\npump /1Q #query pump\npump /1?6 #report valve position\npump /1A2400R #go to absolute position 2400 (= pump 200 ul)\npump /1Q #query pump\npump /1? #report absolute plunger position (the plunger should be moving to 0)\nwait-min 1 #wait 1 minute\npump /1? #report absolute plunger position (the plunger should have finished moving)\n# Port 2\npump /1I2R #switch to port 2, clockwise rotation\npump /1Q #query pump\npump /1?6 #report valve position\npump /1A1800R #go to absolute position 1800 (= pump 200 ul)\npump /1Q #query pump\npump /1? #report absolute plunger position (the plunger should be moving to 0)\nwait-min 1 #wait 1 minute\npump /1? #report absolute plunger position (the plunger should have finished moving)\n# Port 4\npump /1I4R #switch to port 4, clockwise rotation\npump /1Q #query pump\npump /1?6 #report valve position\npump /1A1200R #go to absolute position 1200 (= pump 200 ul)\npump /1Q #query pump\npump /1? #report absolute plunger position (the plunger should be moving to 0)\nwait-min 1 #wait 1 minute\npump /1? #report absolute plunger position (the plunger should have finished moving)\n# Port 5\npump /1I5R #switch to port 5, clockwise rotation\npump /1Q #query pump\npump /1?6 #report valve position\npump /1A600R #go to absolute position 600 (= pump 200 ul)\npump /1Q #query pump\npump /1? #report absolute plunger position (the plunger should be moving to 0)\nwait-min 1 #wait 1 minute\npump /1? #report absolute plunger position (the plunger should have finished moving)\n# Port 6\npump /1I6R #switch to port 6, clockwise rotation\npump /1Q #query pump\npump /1?6 #report valve position\npump /1A0R #go to absolute position 0 (= pump 200 ul)\npump /1Q #query pump\npump /1? #report absolute plunger position (the plunger should be moving to 0)\nwait-min 1 #wait 1 minute\npump /1? #report absolute plunger position (the plunger should have finished moving)\n#-------------------------------------------------------\n# Cycle 19\n# Fill the syringe\n#pump /1ZR #initialize pump\npump /1Q #query pump\npump /1? #report absolute plunger position\npump /1?6 #report valve position\nwait-min 1 #wait 1 minute\npump /1N0R #set step resolution: 0.01 mm\npump /1Q #query pump\npump /1? #report absolute plunger position (the plunger should be at 0)\npump /1?6 #report valve position\nwait 1000 #wait 1 second\npump /1V300R #choose speed: 300 steps/s (6000 ul/min)\npump /1Q #query pump\nwait 1000 #wait 1 second\npump /1O3R #go to port 3, counterclockwise rotation\npump /1Q #query pump\npump /1?6 #report valve position\nwait 1000 #wait 1 second\npump /1A3000R #go to absolute position 3000 (= draw 1 ml)\nwait 30000 #wait 30 seconds\npump /1Q #query pump\npump /1? #report absolute plunger position (the plunger should have finished moving)\n#pump /1?6 #report valve position\n# The sequential pumping begins\n# Port 1\npump /1O1R #switch to port 1, counterclockwise rotation\npump /1Q #query pump\npump /1?6 #report valve position\npump /1A2400R #go to absolute position 2400 (= pump 200 ul)\npump /1Q #query pump\npump /1? #report absolute plunger position (the plunger should be moving to 0)\nwait-min 1 #wait 1 minute\npump /1? #report absolute plunger position (the plunger should have finished moving)\n# Port 2\npump /1I2R #switch to port 2, clockwise rotation\npump /1Q #query pump\npump /1?6 #report valve position\npump /1A1800R #go to absolute position 1800 (= pump 200 ul)\npump /1Q #query pump\npump /1? #report absolute plunger position (the plunger should be moving to 0)\nwait-min 1 #wait 1 minute\npump /1? #report absolute plunger position (the plunger should have finished moving)\n# Port 4\npump /1I4R #switch to port 4, clockwise rotation\npump /1Q #query pump\npump /1?6 #report valve position\npump /1A1200R #go to absolute position 1200 (= pump 200 ul)\npump /1Q #query pump\npump /1? #report absolute plunger position (the plunger should be moving to 0)\nwait-min 1 #wait 1 minute\npump /1? #report absolute plunger position (the plunger should have finished moving)\n# Port 5\npump /1I5R #switch to port 5, clockwise rotation\npump /1Q #query pump\npump /1?6 #report valve position\npump /1A600R #go to absolute position 600 (= pump 200 ul)\npump /1Q #query pump\npump /1? #report absolute plunger position (the plunger should be moving to 0)\nwait-min 1 #wait 1 minute\npump /1? #report absolute plunger position (the plunger should have finished moving)\n# Port 6\npump /1I6R #switch to port 6, clockwise rotation\npump /1Q #query pump\npump /1?6 #report valve position\npump /1A0R #go to absolute position 0 (= pump 200 ul)\npump /1Q #query pump\npump /1? #report absolute plunger position (the plunger should be moving to 0)\nwait-min 1 #wait 1 minute\npump /1? #report absolute plunger position (the plunger should have finished moving)\n#-------------------------------------------------------\n# Cycle 20\n# Fill the syringe\n#pump /1ZR #initialize pump\npump /1Q #query pump\npump /1? #report absolute plunger position\npump /1?6 #report valve position\nwait-min 1 #wait 1 minute\npump /1N0R #set step resolution: 0.01 mm\npump /1Q #query pump\npump /1? #report absolute plunger position (the plunger should be at 0)\npump /1?6 #report valve position\nwait 1000 #wait 1 second\npump /1V300R #choose speed: 300 steps/s (6000 ul/min)\npump /1Q #query pump\nwait 1000 #wait 1 second\npump /1O3R #go to port 3, counterclockwise rotation\npump /1Q #query pump\npump /1?6 #report valve position\nwait 1000 #wait 1 second\npump /1A3000R #go to absolute position 3000 (= draw 1 ml)\nwait 30000 #wait 30 seconds\npump /1Q #query pump\npump /1? #report absolute plunger position (the plunger should have finished moving)\n#pump /1?6 #report valve position\n# The sequential pumping begins\n# Port 1\npump /1O1R #switch to port 1, counterclockwise rotation\npump /1Q #query pump\npump /1?6 #report valve position\npump /1A2400R #go to absolute position 2400 (= pump 200 ul)\npump /1Q #query pump\npump /1? #report absolute plunger position (the plunger should be moving to 0)\nwait-min 1 #wait 1 minute\npump /1? #report absolute plunger position (the plunger should have finished moving)\n# Port 2\npump /1I2R #switch to port 2, clockwise rotation\npump /1Q #query pump\npump /1?6 #report valve position\npump /1A1800R #go to absolute position 1800 (= pump 200 ul)\npump /1Q #query pump\npump /1? #report absolute plunger position (the plunger should be moving to 0)\nwait-min 1 #wait 1 minute\npump /1? #report absolute plunger position (the plunger should have finished moving)\n# Port 4\npump /1I4R #switch to port 4, clockwise rotation\npump /1Q #query pump\npump /1?6 #report valve position\npump /1A1200R #go to absolute position 1200 (= pump 200 ul)\npump /1Q #query pump\npump /1? #report absolute plunger position (the plunger should be moving to 0)\nwait-min 1 #wait 1 minute\npump /1? #report absolute plunger position (the plunger should have finished moving)\n# Port 5\npump /1I5R #switch to port 5, clockwise rotation\npump /1Q #query pump\npump /1?6 #report valve position\npump /1A600R #go to absolute position 600 (= pump 200 ul)\npump /1Q #query pump\npump /1? #report absolute plunger position (the plunger should be moving to 0)\nwait-min 1 #wait 1 minute\npump /1? #report absolute plunger position (the plunger should have finished moving)\n# Port 6\npump /1I6R #switch to port 6, clockwise rotation\npump /1Q #query pump\npump /1?6 #report valve position\npump /1A0R #go to absolute position 0 (= pump 200 ul)\npump /1Q #query pump\npump /1? #report absolute plunger position (the plunger should be moving to 0)\nwait-min 1 #wait 1 minute\npump /1? #report absolute plunger position (the plunger should have finished moving)\n#-------------------------------------------------------\n# Cycle 21\n# Fill the syringe\npump /1Q #query pump\npump /1? #report absolute plunger position\n#pump /1?6 #report valve position\nwait-min 1 #wait 1 minute\npump /1N0R #set step resolution: 0.01 mm\npump /1Q #query pump\npump /1? #report absolute plunger position (the plunger should be at 0)\npump /1?6 #report valve position\nwait 1000 #wait 1 second\npump /1V300R #choose speed: 300 steps/s (6000 ul/min)\npump /1Q #query pump\nwait 1000 #wait 1 second\npump /1I3R #go to port 3, clockwise rotation\npump /1Q #query pump\npump /1?6 #report valve position\nwait 1000 #wait 1 second\npump /1A3000R #go to absolute position 3000 (= draw 1 ml)\nwait 30000 #wait 30 seconds\npump /1Q #query pump\npump /1? #report absolute plunger position (the plunger should have finished moving)\n#pump /1?6 #report valve position\n# The sequential pumping begins\n# Port 1\npump /1O1R #switch to port 1, counterclockwise rotation\npump /1Q #query pump\npump /1?6 #report valve position\npump /1A2400R #go to absolute position 2400 (= pump 200 ul)\npump /1Q #query pump\npump /1? #report absolute plunger position (the plunger should be moving to 0)\nwait-min 1 #wait 1 minute\npump /1? #report absolute plunger position (the plunger should have finished moving)\n# Port 2\npump /1I2R #switch to port 2, clockwise rotation\npump /1Q #query pump\npump /1?6 #report valve position\npump /1A1800R #go to absolute position 1800 (= pump 200 ul)\npump /1Q #query pump\npump /1? #report absolute plunger position (the plunger should be moving to 0)\nwait-min 1 #wait 1 minute\npump /1? #report absolute plunger position (the plunger should have finished moving)\n# Port 4\npump /1I4R #switch to port 4, clockwise rotation\npump /1Q #query pump\npump /1?6 #report valve position\npump /1A1200R #go to absolute position 1200 (= pump 200 ul)\npump /1Q #query pump\npump /1? #report absolute plunger position (the plunger should be moving to 0)\nwait-min 1 #wait 1 minute\npump /1? #report absolute plunger position (the plunger should have finished moving)\n# Port 5\npump /1I5R #switch to port 5, clockwise rotation\npump /1Q #query pump\npump /1?6 #report valve position\npump /1A600R #go to absolute position 600 (= pump 200 ul)\npump /1Q #query pump\npump /1? #report absolute plunger position (the plunger should be moving to 0)\nwait-min 1 #wait 1 minute\npump /1? #report absolute plunger position (the plunger should have finished moving)\n# Port 6\npump /1I6R #switch to port 6, clockwise rotation\npump /1Q #query pump\npump /1?6 #report valve position\npump /1A0R #go to absolute position 0 (= pump 200 ul)\npump /1Q #query pump\npump /1? #report absolute plunger position (the plunger should be moving to 0)\nwait-min 1 #wait 1 minute\npump /1? #report absolute plunger position (the plunger should have finished moving)\n#-------------------------------------------------------\n# Cycle 22\n# Fill the syringe\n#pump /1ZR #initialize pump\npump /1Q #query pump\npump /1? #report absolute plunger position\npump /1?6 #report valve position\nwait-min 1 #wait 1 minute\npump /1N0R #set step resolution: 0.01 mm\npump /1Q #query pump\npump /1? #report absolute plunger position (the plunger should be at 0)\npump /1?6 #report valve position\nwait 1000 #wait 1 second\npump /1V300R #choose speed: 300 steps/s (6000 ul/min)\npump /1Q #query pump\nwait 1000 #wait 1 second\npump /1O3R #go to port 3, counterclockwise rotation\npump /1Q #query pump\npump /1?6 #report valve position\nwait 1000 #wait 1 second\npump /1A3000R #go to absolute position 3000 (= draw 1 ml)\nwait 30000 #wait 30 seconds\npump /1Q #query pump\npump /1? #report absolute plunger position (the plunger should have finished moving)\n#pump /1?6 #report valve position\n# The sequential pumping begins\n# Port 1\npump /1O1R #switch to port 1, counterclockwise rotation\npump /1Q #query pump\npump /1?6 #report valve position\npump /1A2400R #go to absolute position 2400 (= pump 200 ul)\npump /1Q #query pump\npump /1? #report absolute plunger position (the plunger should be moving to 0)\nwait-min 1 #wait 1 minute\npump /1? #report absolute plunger position (the plunger should have finished moving)\n# Port 2\npump /1I2R #switch to port 2, clockwise rotation\npump /1Q #query pump\npump /1?6 #report valve position\npump /1A1800R #go to absolute position 1800 (= pump 200 ul)\npump /1Q #query pump\npump /1? #report absolute plunger position (the plunger should be moving to 0)\nwait-min 1 #wait 1 minute\npump /1? #report absolute plunger position (the plunger should have finished moving)\n# Port 4\npump /1I4R #switch to port 4, clockwise rotation\npump /1Q #query pump\npump /1?6 #report valve position\npump /1A1200R #go to absolute position 1200 (= pump 200 ul)\npump /1Q #query pump\npump /1? #report absolute plunger position (the plunger should be moving to 0)\nwait-min 1 #wait 1 minute\npump /1? #report absolute plunger position (the plunger should have finished moving)\n# Port 5\npump /1I5R #switch to port 5, clockwise rotation\npump /1Q #query pump\npump /1?6 #report valve position\npump /1A600R #go to absolute position 600 (= pump 200 ul)\npump /1Q #query pump\npump /1? #report absolute plunger position (the plunger should be moving to 0)\nwait-min 1 #wait 1 minute\npump /1? #report absolute plunger position (the plunger should have finished moving)\n# Port 6\npump /1I6R #switch to port 6, clockwise rotation\npump /1Q #query pump\npump /1?6 #report valve position\npump /1A0R #go to absolute position 0 (= pump 200 ul)\npump /1Q #query pump\npump /1? #report absolute plunger position (the plunger should be moving to 0)\nwait-min 1 #wait 1 minute\npump /1? #report absolute plunger position (the plunger should have finished moving)\n#-------------------------------------------------------\n# Cycle 23\n# Fill the syringe\n#pump /1ZR #initialize pump\npump /1Q #query pump\npump /1? #report absolute plunger position\npump /1?6 #report valve position\nwait-min 1 #wait 1 minute\npump /1N0R #set step resolution: 0.01 mm\npump /1Q #query pump\npump /1? #report absolute plunger position (the plunger should be at 0)\npump /1?6 #report valve position\nwait 1000 #wait 1 second\npump /1V300R #choose speed: 300 steps/s (6000 ul/min)\npump /1Q #query pump\nwait 1000 #wait 1 second\npump /1O3R #go to port 3, counterclockwise rotation\npump /1Q #query pump\npump /1?6 #report valve position\nwait 1000 #wait 1 second\npump /1A3000R #go to absolute position 3000 (= draw 1 ml)\nwait 30000 #wait 30 seconds\npump /1Q #query pump\npump /1? #report absolute plunger position (the plunger should have finished moving)\n#pump /1?6 #report valve position\n# The sequential pumping begins\n# Port 1\npump /1O1R #switch to port 1, counterclockwise rotation\npump /1Q #query pump\npump /1?6 #report valve position\npump /1A2400R #go to absolute position 2400 (= pump 200 ul)\npump /1Q #query pump\npump /1? #report absolute plunger position (the plunger should be moving to 0)\nwait-min 1 #wait 1 minute\npump /1? #report absolute plunger position (the plunger should have finished moving)\n# Port 2\npump /1I2R #switch to port 2, clockwise rotation\npump /1Q #query pump\npump /1?6 #report valve position\npump /1A1800R #go to absolute position 1800 (= pump 200 ul)\npump /1Q #query pump\npump /1? #report absolute plunger position (the plunger should be moving to 0)\nwait-min 1 #wait 1 minute\npump /1? #report absolute plunger position (the plunger should have finished moving)\n# Port 4\npump /1I4R #switch to port 4, clockwise rotation\npump /1Q #query pump\npump /1?6 #report valve position\npump /1A1200R #go to absolute position 1200 (= pump 200 ul)\npump /1Q #query pump\npump /1? #report absolute plunger position (the plunger should be moving to 0)\nwait-min 1 #wait 1 minute\npump /1? #report absolute plunger position (the plunger should have finished moving)\n# Port 5\npump /1I5R #switch to port 5, clockwise rotation\npump /1Q #query pump\npump /1?6 #report valve position\npump /1A600R #go to absolute position 600 (= pump 200 ul)\npump /1Q #query pump\npump /1? #report absolute plunger position (the plunger should be moving to 0)\nwait-min 1 #wait 1 minute\npump /1? #report absolute plunger position (the plunger should have finished moving)\n# Port 6\npump /1I6R #switch to port 6, clockwise rotation\npump /1Q #query pump\npump /1?6 #report valve position\npump /1A0R #go to absolute position 0 (= pump 200 ul)\npump /1Q #query pump\npump /1? #report absolute plunger position (the plunger should be moving to 0)\nwait-min 1 #wait 1 minute\npump /1? #report absolute plunger position (the plunger should have finished moving)\n#-------------------------------------------------------\n# Cycle 24\n# Fill the syringe\n#pump /1ZR #initialize pump\npump /1Q #query pump\npump /1? #report absolute plunger position\npump /1?6 #report valve position\nwait-min 1 #wait 1 minute\npump /1N0R #set step resolution: 0.01 mm\npump /1Q #query pump\npump /1? #report absolute plunger position (the plunger should be at 0)\npump /1?6 #report valve position\nwait 1000 #wait 1 second\npump /1V300R #choose speed: 300 steps/s (6000 ul/min)\npump /1Q #query pump\nwait 1000 #wait 1 second\npump /1O3R #go to port 3, counterclockwise rotation\npump /1Q #query pump\npump /1?6 #report valve position\nwait 1000 #wait 1 second\npump /1A3000R #go to absolute position 3000 (= draw 1 ml)\nwait 30000 #wait 30 seconds\npump /1Q #query pump\npump /1? #report absolute plunger position (the plunger should have finished moving)\n#pump /1?6 #report valve position\n# The sequential pumping begins\n# Port 1\npump /1O1R #switch to port 1, counterclockwise rotation\npump /1Q #query pump\npump /1?6 #report valve position\npump /1A2400R #go to absolute position 2400 (= pump 200 ul)\npump /1Q #query pump\npump /1? #report absolute plunger position (the plunger should be moving to 0)\nwait-min 1 #wait 1 minute\npump /1? #report absolute plunger position (the plunger should have finished moving)\n# Port 2\npump /1I2R #switch to port 2, clockwise rotation\npump /1Q #query pump\npump /1?6 #report valve position\npump /1A1800R #go to absolute position 1800 (= pump 200 ul)\npump /1Q #query pump\npump /1? #report absolute plunger position (the plunger should be moving to 0)\nwait-min 1 #wait 1 minute\npump /1? #report absolute plunger position (the plunger should have finished moving)\n# Port 4\npump /1I4R #switch to port 4, clockwise rotation\npump /1Q #query pump\npump /1?6 #report valve position\npump /1A1200R #go to absolute position 1200 (= pump 200 ul)\npump /1Q #query pump\npump /1? #report absolute plunger position (the plunger should be moving to 0)\nwait-min 1 #wait 1 minute\npump /1? #report absolute plunger position (the plunger should have finished moving)\n# Port 5\npump /1I5R #switch to port 5, clockwise rotation\npump /1Q #query pump\npump /1?6 #report valve position\npump /1A600R #go to absolute position 600 (= pump 200 ul)\npump /1Q #query pump\npump /1? #report absolute plunger position (the plunger should be moving to 0)\nwait-min 1 #wait 1 minute\npump /1? #report absolute plunger position (the plunger should have finished moving)\n# Port 6\npump /1I6R #switch to port 6, clockwise rotation\npump /1Q #query pump\npump /1?6 #report valve position\npump /1A0R #go to absolute position 0 (= pump 200 ul)\npump /1Q #query pump\npump /1? #report absolute plunger position (the plunger should be moving to 0)\nwait-min 1 #wait 1 minute\npump /1? #report absolute plunger position (the plunger should have finished moving)\n#-------------------------------------------------------\n# Cycle 25\n# Fill the syringe\npump /1Q #query pump\npump /1? #report absolute plunger position\n#pump /1?6 #report valve position\nwait-min 1 #wait 1 minute\npump /1N0R #set step resolution: 0.01 mm\npump /1Q #query pump\npump /1? #report absolute plunger position (the plunger should be at 0)\npump /1?6 #report valve position\nwait 1000 #wait 1 second\npump /1V300R #choose speed: 300 steps/s (6000 ul/min)\npump /1Q #query pump\nwait 1000 #wait 1 second\npump /1I3R #go to port 3, clockwise rotation\npump /1Q #query pump\npump /1?6 #report valve position\nwait 1000 #wait 1 second\npump /1A3000R #go to absolute position 3000 (= draw 1 ml)\nwait 30000 #wait 30 seconds\npump /1Q #query pump\npump /1? #report absolute plunger position (the plunger should have finished moving)\n#pump /1?6 #report valve position\n# The sequential pumping begins\n# Port 1\npump /1O1R #switch to port 1, counterclockwise rotation\npump /1Q #query pump\npump /1?6 #report valve position\npump /1A2400R #go to absolute position 2400 (= pump 200 ul)\npump /1Q #query pump\npump /1? #report absolute plunger position (the plunger should be moving to 0)\nwait-min 1 #wait 1 minute\npump /1? #report absolute plunger position (the plunger should have finished moving)\n# Port 2\npump /1I2R #switch to port 2, clockwise rotation\npump /1Q #query pump\npump /1?6 #report valve position\npump /1A1800R #go to absolute position 1800 (= pump 200 ul)\npump /1Q #query pump\npump /1? #report absolute plunger position (the plunger should be moving to 0)\nwait-min 1 #wait 1 minute\npump /1? #report absolute plunger position (the plunger should have finished moving)\n# Port 4\npump /1I4R #switch to port 4, clockwise rotation\npump /1Q #query pump\npump /1?6 #report valve position\npump /1A1200R #go to absolute position 1200 (= pump 200 ul)\npump /1Q #query pump\npump /1? #report absolute plunger position (the plunger should be moving to 0)\nwait-min 1 #wait 1 minute\npump /1? #report absolute plunger position (the plunger should have finished moving)\n# Port 5\npump /1I5R #switch to port 5, clockwise rotation\npump /1Q #query pump\npump /1?6 #report valve position\npump /1A600R #go to absolute position 600 (= pump 200 ul)\npump /1Q #query pump\npump /1? #report absolute plunger position (the plunger should be moving to 0)\nwait-min 1 #wait 1 minute\npump /1? #report absolute plunger position (the plunger should have finished moving)\n# Port 6\npump /1I6R #switch to port 6, clockwise rotation\npump /1Q #query pump\npump /1?6 #report valve position\npump /1A0R #go to absolute position 0 (= pump 200 ul)\npump /1Q #query pump\npump /1? #report absolute plunger position (the plunger should be moving to 0)\nwait-min 1 #wait 1 minute\npump /1? #report absolute plunger position (the plunger should have finished moving)\n#-------------------------------------------------------\n# Cycle 26\n# Fill the syringe\n#pump /1ZR #initialize pump\npump /1Q #query pump\npump /1? #report absolute plunger position\npump /1?6 #report valve position\nwait-min 1 #wait 1 minute\npump /1N0R #set step resolution: 0.01 mm\npump /1Q #query pump\npump /1? #report absolute plunger position (the plunger should be at 0)\npump /1?6 #report valve position\nwait 1000 #wait 1 second\npump /1V300R #choose speed: 300 steps/s (6000 ul/min)\npump /1Q #query pump\nwait 1000 #wait 1 second\npump /1O3R #go to port 3, counterclockwise rotation\npump /1Q #query pump\npump /1?6 #report valve position\nwait 1000 #wait 1 second\npump /1A3000R #go to absolute position 3000 (= draw 1 ml)\nwait 30000 #wait 30 seconds\npump /1Q #query pump\npump /1? #report absolute plunger position (the plunger should have finished moving)\n#pump /1?6 #report valve position\n# The sequential pumping begins\n# Port 1\npump /1O1R #switch to port 1, counterclockwise rotation\npump /1Q #query pump\npump /1?6 #report valve position\npump /1A2400R #go to absolute position 2400 (= pump 200 ul)\npump /1Q #query pump\npump /1? #report absolute plunger position (the plunger should be moving to 0)\nwait-min 1 #wait 1 minute\npump /1? #report absolute plunger position (the plunger should have finished moving)\n# Port 2\npump /1I2R #switch to port 2, clockwise rotation\npump /1Q #query pump\npump /1?6 #report valve position\npump /1A1800R #go to absolute position 1800 (= pump 200 ul)\npump /1Q #query pump\npump /1? #report absolute plunger position (the plunger should be moving to 0)\nwait-min 1 #wait 1 minute\npump /1? #report absolute plunger position (the plunger should have finished moving)\n# Port 4\npump /1I4R #switch to port 4, clockwise rotation\npump /1Q #query pump\npump /1?6 #report valve position\npump /1A1200R #go to absolute position 1200 (= pump 200 ul)\npump /1Q #query pump\npump /1? #report absolute plunger position (the plunger should be moving to 0)\nwait-min 1 #wait 1 minute\npump /1? #report absolute plunger position (the plunger should have finished moving)\n# Port 5\npump /1I5R #switch to port 5, clockwise rotation\npump /1Q #query pump\npump /1?6 #report valve position\npump /1A600R #go to absolute position 600 (= pump 200 ul)\npump /1Q #query pump\npump /1? #report absolute plunger position (the plunger should be moving to 0)\nwait-min 1 #wait 1 minute\npump /1? #report absolute plunger position (the plunger should have finished moving)\n# Port 6\npump /1I6R #switch to port 6, clockwise rotation\npump /1Q #query pump\npump /1?6 #report valve position\npump /1A0R #go to absolute position 0 (= pump 200 ul)\npump /1Q #query pump\npump /1? #report absolute plunger position (the plunger should be moving to 0)\nwait-min 1 #wait 1 minute\npump /1? #report absolute plunger position (the plunger should have finished moving)\n#-------------------------------------------------------\n# Cycle 27\n# Fill the syringe\n#pump /1ZR #initialize pump\npump /1Q #query pump\npump /1? #report absolute plunger position\npump /1?6 #report valve position\nwait-min 1 #wait 1 minute\npump /1N0R #set step resolution: 0.01 mm\npump /1Q #query pump\npump /1? #report absolute plunger position (the plunger should be at 0)\npump /1?6 #report valve position\nwait 1000 #wait 1 second\npump /1V300R #choose speed: 300 steps/s (6000 ul/min)\npump /1Q #query pump\nwait 1000 #wait 1 second\npump /1O3R #go to port 3, counterclockwise rotation\npump /1Q #query pump\npump /1?6 #report valve position\nwait 1000 #wait 1 second\npump /1A3000R #go to absolute position 3000 (= draw 1 ml)\nwait 30000 #wait 30 seconds\npump /1Q #query pump\npump /1? #report absolute plunger position (the plunger should have finished moving)\n#pump /1?6 #report valve position\n# The sequential pumping begins\n# Port 1\npump /1O1R #switch to port 1, counterclockwise rotation\npump /1Q #query pump\npump /1?6 #report valve position\npump /1A2400R #go to absolute position 2400 (= pump 200 ul)\npump /1Q #query pump\npump /1? #report absolute plunger position (the plunger should be moving to 0)\nwait-min 1 #wait 1 minute\npump /1? #report absolute plunger position (the plunger should have finished moving)\n# Port 2\npump /1I2R #switch to port 2, clockwise rotation\npump /1Q #query pump\npump /1?6 #report valve position\npump /1A1800R #go to absolute position 1800 (= pump 200 ul)\npump /1Q #query pump\npump /1? #report absolute plunger position (the plunger should be moving to 0)\nwait-min 1 #wait 1 minute\npump /1? #report absolute plunger position (the plunger should have finished moving)\n# Port 4\npump /1I4R #switch to port 4, clockwise rotation\npump /1Q #query pump\npump /1?6 #report valve position\npump /1A1200R #go to absolute position 1200 (= pump 200 ul)\npump /1Q #query pump\npump /1? #report absolute plunger position (the plunger should be moving to 0)\nwait-min 1 #wait 1 minute\npump /1? #report absolute plunger position (the plunger should have finished moving)\n# Port 5\npump /1I5R #switch to port 5, clockwise rotation\npump /1Q #query pump\npump /1?6 #report valve position\npump /1A600R #go to absolute position 600 (= pump 200 ul)\npump /1Q #query pump\npump /1? #report absolute plunger position (the plunger should be moving to 0)\nwait-min 1 #wait 1 minute\npump /1? #report absolute plunger position (the plunger should have finished moving)\n# Port 6\npump /1I6R #switch to port 6, clockwise rotation\npump /1Q #query pump\npump /1?6 #report valve position\npump /1A0R #go to absolute position 0 (= pump 200 ul)\npump /1Q #query pump\npump /1? #report absolute plunger position (the plunger should be moving to 0)\nwait-min 1 #wait 1 minute\npump /1? #report absolute plunger position (the plunger should have finished moving)\n#-------------------------------------------------------\n# Cycle 28\n# Fill the syringe\n#pump /1ZR #initialize pump\npump /1Q #query pump\npump /1? #report absolute plunger position\npump /1?6 #report valve position\nwait-min 1 #wait 1 minute\npump /1N0R #set step resolution: 0.01 mm\npump /1Q #query pump\npump /1? #report absolute plunger position (the plunger should be at 0)\npump /1?6 #report valve position\nwait 1000 #wait 1 second\npump /1V300R #choose speed: 300 steps/s (6000 ul/min)\npump /1Q #query pump\nwait 1000 #wait 1 second\npump /1O3R #go to port 3, counterclockwise rotation\npump /1Q #query pump\npump /1?6 #report valve position\nwait 1000 #wait 1 second\npump /1A3000R #go to absolute position 3000 (= draw 1 ml)\nwait 30000 #wait 30 seconds\npump /1Q #query pump\npump /1? #report absolute plunger position (the plunger should have finished moving)\n#pump /1?6 #report valve position\n# The sequential pumping begins\n# Port 1\npump /1O1R #switch to port 1, counterclockwise rotation\npump /1Q #query pump\npump /1?6 #report valve position\npump /1A2400R #go to absolute position 2400 (= pump 200 ul)\npump /1Q #query pump\npump /1? #report absolute plunger position (the plunger should be moving to 0)\nwait-min 1 #wait 1 minute\npump /1? #report absolute plunger position (the plunger should have finished moving)\n# Port 2\npump /1I2R #switch to port 2, clockwise rotation\npump /1Q #query pump\npump /1?6 #report valve position\npump /1A1800R #go to absolute position 1800 (= pump 200 ul)\npump /1Q #query pump\npump /1? #report absolute plunger position (the plunger should be moving to 0)\nwait-min 1 #wait 1 minute\npump /1? #report absolute plunger position (the plunger should have finished moving)\n# Port 4\npump /1I4R #switch to port 4, clockwise rotation\npump /1Q #query pump\npump /1?6 #report valve position\npump /1A1200R #go to absolute position 1200 (= pump 200 ul)\npump /1Q #query pump\npump /1? #report absolute plunger position (the plunger should be moving to 0)\nwait-min 1 #wait 1 minute\npump /1? #report absolute plunger position (the plunger should have finished moving)\n# Port 5\npump /1I5R #switch to port 5, clockwise rotation\npump /1Q #query pump\npump /1?6 #report valve position\npump /1A600R #go to absolute position 600 (= pump 200 ul)\npump /1Q #query pump\npump /1? #report absolute plunger position (the plunger should be moving to 0)\nwait-min 1 #wait 1 minute\npump /1? #report absolute plunger position (the plunger should have finished moving)\n# Port 6\npump /1I6R #switch to port 6, clockwise rotation\npump /1Q #query pump\npump /1?6 #report valve position\npump /1A0R #go to absolute position 0 (= pump 200 ul)\npump /1Q #query pump\npump /1? #report absolute plunger position (the plunger should be moving to 0)\nwait-min 1 #wait 1 minute\npump /1? #report absolute plunger position (the plunger should have finished moving)\n#-------------------------------------------------------\n# Cycle 29\n# Fill the syringe\npump /1Q #query pump\npump /1? #report absolute plunger position\n#pump /1?6 #report valve position\nwait-min 1 #wait 1 minute\npump /1N0R #set step resolution: 0.01 mm\npump /1Q #query pump\npump /1? #report absolute plunger position (the plunger should be at 0)\npump /1?6 #report valve position\nwait 1000 #wait 1 second\npump /1V300R #choose speed: 300 steps/s (6000 ul/min)\npump /1Q #query pump\nwait 1000 #wait 1 second\npump /1I3R #go to port 3, clockwise rotation\npump /1Q #query pump\npump /1?6 #report valve position\nwait 1000 #wait 1 second\npump /1A3000R #go to absolute position 3000 (= draw 1 ml)\nwait 30000 #wait 30 seconds\npump /1Q #query pump\npump /1? #report absolute plunger position (the plunger should have finished moving)\n#pump /1?6 #report valve position\n# The sequential pumping begins\n# Port 1\npump /1O1R #switch to port 1, counterclockwise rotation\npump /1Q #query pump\npump /1?6 #report valve position\npump /1A2400R #go to absolute position 2400 (= pump 200 ul)\npump /1Q #query pump\npump /1? #report absolute plunger position (the plunger should be moving to 0)\nwait-min 1 #wait 1 minute\npump /1? #report absolute plunger position (the plunger should have finished moving)\n# Port 2\npump /1I2R #switch to port 2, clockwise rotation\npump /1Q #query pump\npump /1?6 #report valve position\npump /1A1800R #go to absolute position 1800 (= pump 200 ul)\npump /1Q #query pump\npump /1? #report absolute plunger position (the plunger should be moving to 0)\nwait-min 1 #wait 1 minute\npump /1? #report absolute plunger position (the plunger should have finished moving)\n# Port 4\npump /1I4R #switch to port 4, clockwise rotation\npump /1Q #query pump\npump /1?6 #report valve position\npump /1A1200R #go to absolute position 1200 (= pump 200 ul)\npump /1Q #query pump\npump /1? #report absolute plunger position (the plunger should be moving to 0)\nwait-min 1 #wait 1 minute\npump /1? #report absolute plunger position (the plunger should have finished moving)\n# Port 5\npump /1I5R #switch to port 5, clockwise rotation\npump /1Q #query pump\npump /1?6 #report valve position\npump /1A600R #go to absolute position 600 (= pump 200 ul)\npump /1Q #query pump\npump /1? #report absolute plunger position (the plunger should be moving to 0)\nwait-min 1 #wait 1 minute\npump /1? #report absolute plunger position (the plunger should have finished moving)\n# Port 6\npump /1I6R #switch to port 6, clockwise rotation\npump /1Q #query pump\npump /1?6 #report valve position\npump /1A0R #go to absolute position 0 (= pump 200 ul)\npump /1Q #query pump\npump /1? #report absolute plunger position (the plunger should be moving to 0)\nwait-min 1 #wait 1 minute\npump /1? #report absolute plunger position (the plunger should have finished moving)\n#-------------------------------------------------------\n# Cycle 30\n# Fill the syringe\n#pump /1ZR #initialize pump\npump /1Q #query pump\npump /1? #report absolute plunger position\npump /1?6 #report valve position\nwait-min 1 #wait 1 minute\npump /1N0R #set step resolution: 0.01 mm\npump /1Q #query pump\npump /1? #report absolute plunger position (the plunger should be at 0)\npump /1?6 #report valve position\nwait 1000 #wait 1 second\npump /1V300R #choose speed: 300 steps/s (6000 ul/min)\npump /1Q #query pump\nwait 1000 #wait 1 second\npump /1O3R #go to port 3, counterclockwise rotation\npump /1Q #query pump\npump /1?6 #report valve position\nwait 1000 #wait 1 second\npump /1A3000R #go to absolute position 3000 (= draw 1 ml)\nwait 30000 #wait 30 seconds\npump /1Q #query pump\npump /1? #report absolute plunger position (the plunger should have finished moving)\n#pump /1?6 #report valve position\n# The sequential pumping begins\n# Port 1\npump /1O1R #switch to port 1, counterclockwise rotation\npump /1Q #query pump\npump /1?6 #report valve position\npump /1A2400R #go to absolute position 2400 (= pump 200 ul)\npump /1Q #query pump\npump /1? #report absolute plunger position (the plunger should be moving to 0)\nwait-min 1 #wait 1 minute\npump /1? #report absolute plunger position (the plunger should have finished moving)\n# Port 2\npump /1I2R #switch to port 2, clockwise rotation\npump /1Q #query pump\npump /1?6 #report valve position\npump /1A1800R #go to absolute position 1800 (= pump 200 ul)\npump /1Q #query pump\npump /1? #report absolute plunger position (the plunger should be moving to 0)\nwait-min 1 #wait 1 minute\npump /1? #report absolute plunger position (the plunger should have finished moving)\n# Port 4\npump /1I4R #switch to port 4, clockwise rotation\npump /1Q #query pump\npump /1?6 #report valve position\npump /1A1200R #go to absolute position 1200 (= pump 200 ul)\npump /1Q #query pump\npump /1? #report absolute plunger position (the plunger should be moving to 0)\nwait-min 1 #wait 1 minute\npump /1? #report absolute plunger position (the plunger should have finished moving)\n# Port 5\npump /1I5R #switch to port 5, clockwise rotation\npump /1Q #query pump\npump /1?6 #report valve position\npump /1A600R #go to absolute position 600 (= pump 200 ul)\npump /1Q #query pump\npump /1? #report absolute plunger position (the plunger should be moving to 0)\nwait-min 1 #wait 1 minute\npump /1? #report absolute plunger position (the plunger should have finished moving)\n# Port 6\npump /1I6R #switch to port 6, clockwise rotation\npump /1Q #query pump\npump /1?6 #report valve position\npump /1A0R #go to absolute position 0 (= pump 200 ul)\npump /1Q #query pump\npump /1? #report absolute plunger position (the plunger should be moving to 0)\nwait-min 1 #wait 1 minute\npump /1? #report absolute plunger position (the plunger should have finished moving)\n#-------------------------------------------------------\n# Cycle 31\n# Fill the syringe\n#pump /1ZR #initialize pump\npump /1Q #query pump\npump /1? #report absolute plunger position\npump /1?6 #report valve position\nwait-min 1 #wait 1 minute\npump /1N0R #set step resolution: 0.01 mm\npump /1Q #query pump\npump /1? #report absolute plunger position (the plunger should be at 0)\npump /1?6 #report valve position\nwait 1000 #wait 1 second\npump /1V300R #choose speed: 300 steps/s (6000 ul/min)\npump /1Q #query pump\nwait 1000 #wait 1 second\npump /1O3R #go to port 3, counterclockwise rotation\npump /1Q #query pump\npump /1?6 #report valve position\nwait 1000 #wait 1 second\npump /1A3000R #go to absolute position 3000 (= draw 1 ml)\nwait 30000 #wait 30 seconds\npump /1Q #query pump\npump /1? #report absolute plunger position (the plunger should have finished moving)\n#pump /1?6 #report valve position\n# The sequential pumping begins\n# Port 1\npump /1O1R #switch to port 1, counterclockwise rotation\npump /1Q #query pump\npump /1?6 #report valve position\npump /1A2400R #go to absolute position 2400 (= pump 200 ul)\npump /1Q #query pump\npump /1? #report absolute plunger position (the plunger should be moving to 0)\nwait-min 1 #wait 1 minute\npump /1? #report absolute plunger position (the plunger should have finished moving)\n# Port 2\npump /1I2R #switch to port 2, clockwise rotation\npump /1Q #query pump\npump /1?6 #report valve position\npump /1A1800R #go to absolute position 1800 (= pump 200 ul)\npump /1Q #query pump\npump /1? #report absolute plunger position (the plunger should be moving to 0)\nwait-min 1 #wait 1 minute\npump /1? #report absolute plunger position (the plunger should have finished moving)\n# Port 4\npump /1I4R #switch to port 4, clockwise rotation\npump /1Q #query pump\npump /1?6 #report valve position\npump /1A1200R #go to absolute position 1200 (= pump 200 ul)\npump /1Q #query pump\npump /1? #report absolute plunger position (the plunger should be moving to 0)\nwait-min 1 #wait 1 minute\npump /1? #report absolute plunger position (the plunger should have finished moving)\n# Port 5\npump /1I5R #switch to port 5, clockwise rotation\npump /1Q #query pump\npump /1?6 #report valve position\npump /1A600R #go to absolute position 600 (= pump 200 ul)\npump /1Q #query pump\npump /1? #report absolute plunger position (the plunger should be moving to 0)\nwait-min 1 #wait 1 minute\npump /1? #report absolute plunger position (the plunger should have finished moving)\n# Port 6\npump /1I6R #switch to port 6, clockwise rotation\npump /1Q #query pump\npump /1?6 #report valve position\npump /1A0R #go to absolute position 0 (= pump 200 ul)\npump /1Q #query pump\npump /1? #report absolute plunger position (the plunger should be moving to 0)\nwait-min 1 #wait 1 minute\npump /1? #report absolute plunger position (the plunger should have finished moving)\n#-------------------------------------------------------\n# Cycle 32\n# Fill the syringe\n#pump /1ZR #initialize pump\npump /1Q #query pump\npump /1? #report absolute plunger position\npump /1?6 #report valve position\nwait-min 1 #wait 1 minute\npump /1N0R #set step resolution: 0.01 mm\npump /1Q #query pump\npump /1? #report absolute plunger position (the plunger should be at 0)\npump /1?6 #report valve position\nwait 1000 #wait 1 second\npump /1V300R #choose speed: 300 steps/s (6000 ul/min)\npump /1Q #query pump\nwait 1000 #wait 1 second\npump /1O3R #go to port 3, counterclockwise rotation\npump /1Q #query pump\npump /1?6 #report valve position\nwait 1000 #wait 1 second\npump /1A3000R #go to absolute position 3000 (= draw 1 ml)\nwait 30000 #wait 30 seconds\npump /1Q #query pump\npump /1? #report absolute plunger position (the plunger should have finished moving)\n#pump /1?6 #report valve position\n# The sequential pumping begins\n# Port 1\npump /1O1R #switch to port 1, counterclockwise rotation\npump /1Q #query pump\npump /1?6 #report valve position\npump /1A2400R #go to absolute position 2400 (= pump 200 ul)\npump /1Q #query pump\npump /1? #report absolute plunger position (the plunger should be moving to 0)\nwait-min 1 #wait 1 minute\npump /1? #report absolute plunger position (the plunger should have finished moving)\n# Port 2\npump /1I2R #switch to port 2, clockwise rotation\npump /1Q #query pump\npump /1?6 #report valve position\npump /1A1800R #go to absolute position 1800 (= pump 200 ul)\npump /1Q #query pump\npump /1? #report absolute plunger position (the plunger should be moving to 0)\nwait-min 1 #wait 1 minute\npump /1? #report absolute plunger position (the plunger should have finished moving)\n# Port 4\npump /1I4R #switch to port 4, clockwise rotation\npump /1Q #query pump\npump /1?6 #report valve position\npump /1A1200R #go to absolute position 1200 (= pump 200 ul)\npump /1Q #query pump\npump /1? #report absolute plunger position (the plunger should be moving to 0)\nwait-min 1 #wait 1 minute\npump /1? #report absolute plunger position (the plunger should have finished moving)\n# Port 5\npump /1I5R #switch to port 5, clockwise rotation\npump /1Q #query pump\npump /1?6 #report valve position\npump /1A600R #go to absolute position 600 (= pump 200 ul)\npump /1Q #query pump\npump /1? #report absolute plunger position (the plunger should be moving to 0)\nwait-min 1 #wait 1 minute\npump /1? #report absolute plunger position (the plunger should have finished moving)\n# Port 6\npump /1I6R #switch to port 6, clockwise rotation\npump /1Q #query pump\npump /1?6 #report valve position\npump /1A0R #go to absolute position 0 (= pump 200 ul)\npump /1Q #query pump\npump /1? #report absolute plunger position (the plunger should be moving to 0)\nwait-min 1 #wait 1 minute\npump /1? #report absolute plunger position (the plunger should have finished moving)\n#-------------------------------------------------------\n# Cycle 33\n# Fill the syringe\npump /1Q #query pump\npump /1? #report absolute plunger position\n#pump /1?6 #report valve position\nwait-min 1 #wait 1 minute\npump /1N0R #set step resolution: 0.01 mm\npump /1Q #query pump\npump /1? #report absolute plunger position (the plunger should be at 0)\npump /1?6 #report valve position\nwait 1000 #wait 1 second\npump /1V300R #choose speed: 300 steps/s (6000 ul/min)\npump /1Q #query pump\nwait 1000 #wait 1 second\npump /1I3R #go to port 3, clockwise rotation\npump /1Q #query pump\npump /1?6 #report valve position\nwait 1000 #wait 1 second\npump /1A3000R #go to absolute position 3000 (= draw 1 ml)\nwait 30000 #wait 30 seconds\npump /1Q #query pump\npump /1? #report absolute plunger position (the plunger should have finished moving)\n#pump /1?6 #report valve position\n# The sequential pumping begins\n# Port 1\npump /1O1R #switch to port 1, counterclockwise rotation\npump /1Q #query pump\npump /1?6 #report valve position\npump /1A2400R #go to absolute position 2400 (= pump 200 ul)\npump /1Q #query pump\npump /1? #report absolute plunger position (the plunger should be moving to 0)\nwait-min 1 #wait 1 minute\npump /1? #report absolute plunger position (the plunger should have finished moving)\n# Port 2\npump /1I2R #switch to port 2, clockwise rotation\npump /1Q #query pump\npump /1?6 #report valve position\npump /1A1800R #go to absolute position 1800 (= pump 200 ul)\npump /1Q #query pump\npump /1? #report absolute plunger position (the plunger should be moving to 0)\nwait-min 1 #wait 1 minute\npump /1? #report absolute plunger position (the plunger should have finished moving)\n# Port 4\npump /1I4R #switch to port 4, clockwise rotation\npump /1Q #query pump\npump /1?6 #report valve position\npump /1A1200R #go to absolute position 1200 (= pump 200 ul)\npump /1Q #query pump\npump /1? #report absolute plunger position (the plunger should be moving to 0)\nwait-min 1 #wait 1 minute\npump /1? #report absolute plunger position (the plunger should have finished moving)\n# Port 5\npump /1I5R #switch to port 5, clockwise rotation\npump /1Q #query pump\npump /1?6 #report valve position\npump /1A600R #go to absolute position 600 (= pump 200 ul)\npump /1Q #query pump\npump /1? #report absolute plunger position (the plunger should be moving to 0)\nwait-min 1 #wait 1 minute\npump /1? #report absolute plunger position (the plunger should have finished moving)\n# Port 6\npump /1I6R #switch to port 6, clockwise rotation\npump /1Q #query pump\npump /1?6 #report valve position\npump /1A0R #go to absolute position 0 (= pump 200 ul)\npump /1Q #query pump\npump /1? #report absolute plunger position (the plunger should be moving to 0)\nwait-min 1 #wait 1 minute\npump /1? #report absolute plunger position (the plunger should have finished moving)\n#-------------------------------------------------------\n# Cycle 34\n# Fill the syringe\n#pump /1ZR #initialize pump\npump /1Q #query pump\npump /1? #report absolute plunger position\npump /1?6 #report valve position\nwait-min 1 #wait 1 minute\npump /1N0R #set step resolution: 0.01 mm\npump /1Q #query pump\npump /1? #report absolute plunger position (the plunger should be at 0)\npump /1?6 #report valve position\nwait 1000 #wait 1 second\npump /1V300R #choose speed: 300 steps/s (6000 ul/min)\npump /1Q #query pump\nwait 1000 #wait 1 second\npump /1O3R #go to port 3, counterclockwise rotation\npump /1Q #query pump\npump /1?6 #report valve position\nwait 1000 #wait 1 second\npump /1A3000R #go to absolute position 3000 (= draw 1 ml)\nwait 30000 #wait 30 seconds\npump /1Q #query pump\npump /1? #report absolute plunger position (the plunger should have finished moving)\n#pump /1?6 #report valve position\n# The sequential pumping begins\n# Port 1\npump /1O1R #switch to port 1, counterclockwise rotation\npump /1Q #query pump\npump /1?6 #report valve position\npump /1A2400R #go to absolute position 2400 (= pump 200 ul)\npump /1Q #query pump\npump /1? #report absolute plunger position (the plunger should be moving to 0)\nwait-min 1 #wait 1 minute\npump /1? #report absolute plunger position (the plunger should have finished moving)\n# Port 2\npump /1I2R #switch to port 2, clockwise rotation\npump /1Q #query pump\npump /1?6 #report valve position\npump /1A1800R #go to absolute position 1800 (= pump 200 ul)\npump /1Q #query pump\npump /1? #report absolute plunger position (the plunger should be moving to 0)\nwait-min 1 #wait 1 minute\npump /1? #report absolute plunger position (the plunger should have finished moving)\n# Port 4\npump /1I4R #switch to port 4, clockwise rotation\npump /1Q #query pump\npump /1?6 #report valve position\npump /1A1200R #go to absolute position 1200 (= pump 200 ul)\npump /1Q #query pump\npump /1? #report absolute plunger position (the plunger should be moving to 0)\nwait-min 1 #wait 1 minute\npump /1? #report absolute plunger position (the plunger should have finished moving)\n# Port 5\npump /1I5R #switch to port 5, clockwise rotation\npump /1Q #query pump\npump /1?6 #report valve position\npump /1A600R #go to absolute position 600 (= pump 200 ul)\npump /1Q #query pump\npump /1? #report absolute plunger position (the plunger should be moving to 0)\nwait-min 1 #wait 1 minute\npump /1? #report absolute plunger position (the plunger should have finished moving)\n# Port 6\npump /1I6R #switch to port 6, clockwise rotation\npump /1Q #query pump\npump /1?6 #report valve position\npump /1A0R #go to absolute position 0 (= pump 200 ul)\npump /1Q #query pump\npump /1? #report absolute plunger position (the plunger should be moving to 0)\nwait-min 1 #wait 1 minute\npump /1? #report absolute plunger position (the plunger should have finished moving)\n#-------------------------------------------------------\n# Cycle 35\n# Fill the syringe\n#pump /1ZR #initialize pump\npump /1Q #query pump\npump /1? #report absolute plunger position\npump /1?6 #report valve position\nwait-min 1 #wait 1 minute\npump /1N0R #set step resolution: 0.01 mm\npump /1Q #query pump\npump /1? #report absolute plunger position (the plunger should be at 0)\npump /1?6 #report valve position\nwait 1000 #wait 1 second\npump /1V300R #choose speed: 300 steps/s (6000 ul/min)\npump /1Q #query pump\nwait 1000 #wait 1 second\npump /1O3R #go to port 3, counterclockwise rotation\npump /1Q #query pump\npump /1?6 #report valve position\nwait 1000 #wait 1 second\npump /1A3000R #go to absolute position 3000 (= draw 1 ml)\nwait 30000 #wait 30 seconds\npump /1Q #query pump\npump /1? #report absolute plunger position (the plunger should have finished moving)\n#pump /1?6 #report valve position\n# The sequential pumping begins\n# Port 1\npump /1O1R #switch to port 1, counterclockwise rotation\npump /1Q #query pump\npump /1?6 #report valve position\npump /1A2400R #go to absolute position 2400 (= pump 200 ul)\npump /1Q #query pump\npump /1? #report absolute plunger position (the plunger should be moving to 0)\nwait-min 1 #wait 1 minute\npump /1? #report absolute plunger position (the plunger should have finished moving)\n# Port 2\npump /1I2R #switch to port 2, clockwise rotation\npump /1Q #query pump\npump /1?6 #report valve position\npump /1A1800R #go to absolute position 1800 (= pump 200 ul)\npump /1Q #query pump\npump /1? #report absolute plunger position (the plunger should be moving to 0)\nwait-min 1 #wait 1 minute\npump /1? #report absolute plunger position (the plunger should have finished moving)\n# Port 4\npump /1I4R #switch to port 4, clockwise rotation\npump /1Q #query pump\npump /1?6 #report valve position\npump /1A1200R #go to absolute position 1200 (= pump 200 ul)\npump /1Q #query pump\npump /1? #report absolute plunger position (the plunger should be moving to 0)\nwait-min 1 #wait 1 minute\npump /1? #report absolute plunger position (the plunger should have finished moving)\n# Port 5\npump /1I5R #switch to port 5, clockwise rotation\npump /1Q #query pump\npump /1?6 #report valve position\npump /1A600R #go to absolute position 600 (= pump 200 ul)\npump /1Q #query pump\npump /1? #report absolute plunger position (the plunger should be moving to 0)\nwait-min 1 #wait 1 minute\npump /1? #report absolute plunger position (the plunger should have finished moving)\n# Port 6\npump /1I6R #switch to port 6, clockwise rotation\npump /1Q #query pump\npump /1?6 #report valve position\npump /1A0R #go to absolute position 0 (= pump 200 ul)\npump /1Q #query pump\npump /1? #report absolute plunger position (the plunger should be moving to 0)\nwait-min 1 #wait 1 minute\npump /1? #report absolute plunger position (the plunger should have finished moving)\n#-------------------------------------------------------\n# Cycle 36\n# Fill the syringe\n#pump /1ZR #initialize pump\npump /1Q #query pump\npump /1? #report absolute plunger position\npump /1?6 #report valve position\nwait-min 1 #wait 1 minute\npump /1N0R #set step resolution: 0.01 mm\npump /1Q #query pump\npump /1? #report absolute plunger position (the plunger should be at 0)\npump /1?6 #report valve position\nwait 1000 #wait 1 second\npump /1V300R #choose speed: 300 steps/s (6000 ul/min)\npump /1Q #query pump\nwait 1000 #wait 1 second\npump /1O3R #go to port 3, counterclockwise rotation\npump /1Q #query pump\npump /1?6 #report valve position\nwait 1000 #wait 1 second\npump /1A3000R #go to absolute position 3000 (= draw 1 ml)\nwait 30000 #wait 30 seconds\npump /1Q #query pump\npump /1? #report absolute plunger position (the plunger should have finished moving)\n#pump /1?6 #report valve position\n# The sequential pumping begins\n# Port 1\npump /1O1R #switch to port 1, counterclockwise rotation\npump /1Q #query pump\npump /1?6 #report valve position\npump /1A2400R #go to absolute position 2400 (= pump 200 ul)\npump /1Q #query pump\npump /1? #report absolute plunger position (the plunger should be moving to 0)\nwait-min 1 #wait 1 minute\npump /1? #report absolute plunger position (the plunger should have finished moving)\n# Port 2\npump /1I2R #switch to port 2, clockwise rotation\npump /1Q #query pump\npump /1?6 #report valve position\npump /1A1800R #go to absolute position 1800 (= pump 200 ul)\npump /1Q #query pump\npump /1? #report absolute plunger position (the plunger should be moving to 0)\nwait-min 1 #wait 1 minute\npump /1? #report absolute plunger position (the plunger should have finished moving)\n# Port 4\npump /1I4R #switch to port 4, clockwise rotation\npump /1Q #query pump\npump /1?6 #report valve position\npump /1A1200R #go to absolute position 1200 (= pump 200 ul)\npump /1Q #query pump\npump /1? #report absolute plunger position (the plunger should be moving to 0)\nwait-min 1 #wait 1 minute\npump /1? #report absolute plunger position (the plunger should have finished moving)\n# Port 5\npump /1I5R #switch to port 5, clockwise rotation\npump /1Q #query pump\npump /1?6 #report valve position\npump /1A600R #go to absolute position 600 (= pump 200 ul)\npump /1Q #query pump\npump /1? #report absolute plunger position (the plunger should be moving to 0)\nwait-min 1 #wait 1 minute\npump /1? #report absolute plunger position (the plunger should have finished moving)\n# Port 6\npump /1I6R #switch to port 6, clockwise rotation\npump /1Q #query pump\npump /1?6 #report valve position\npump /1A0R #go to absolute position 0 (= pump 200 ul)\npump /1Q #query pump\npump /1? #report absolute plunger position (the plunger should be moving to 0)\nwait-min 1 #wait 1 minute\npump /1? #report absolute plunger position (the plunger should have finished moving)\n#-------------------------------------------------------\n# Cycle 37\n# Fill the syringe\npump /1Q #query pump\npump /1? #report absolute plunger position\n#pump /1?6 #report valve position\nwait-min 1 #wait 1 minute\npump /1N0R #set step resolution: 0.01 mm\npump /1Q #query pump\npump /1? #report absolute plunger position (the plunger should be at 0)\npump /1?6 #report valve position\nwait 1000 #wait 1 second\npump /1V300R #choose speed: 300 steps/s (6000 ul/min)\npump /1Q #query pump\nwait 1000 #wait 1 second\npump /1I3R #go to port 3, clockwise rotation\npump /1Q #query pump\npump /1?6 #report valve position\nwait 1000 #wait 1 second\npump /1A3000R #go to absolute position 3000 (= draw 1 ml)\nwait 30000 #wait 30 seconds\npump /1Q #query pump\npump /1? #report absolute plunger position (the plunger should have finished moving)\n#pump /1?6 #report valve position\n# The sequential pumping begins\n# Port 1\npump /1O1R #switch to port 1, counterclockwise rotation\npump /1Q #query pump\npump /1?6 #report valve position\npump /1A2400R #go to absolute position 2400 (= pump 200 ul)\npump /1Q #query pump\npump /1? #report absolute plunger position (the plunger should be moving to 0)\nwait-min 1 #wait 1 minute\npump /1? #report absolute plunger position (the plunger should have finished moving)\n# Port 2\npump /1I2R #switch to port 2, clockwise rotation\npump /1Q #query pump\npump /1?6 #report valve position\npump /1A1800R #go to absolute position 1800 (= pump 200 ul)\npump /1Q #query pump\npump /1? #report absolute plunger position (the plunger should be moving to 0)\nwait-min 1 #wait 1 minute\npump /1? #report absolute plunger position (the plunger should have finished moving)\n# Port 4\npump /1I4R #switch to port 4, clockwise rotation\npump /1Q #query pump\npump /1?6 #report valve position\npump /1A1200R #go to absolute position 1200 (= pump 200 ul)\npump /1Q #query pump\npump /1? #report absolute plunger position (the plunger should be moving to 0)\nwait-min 1 #wait 1 minute\npump /1? #report absolute plunger position (the plunger should have finished moving)\n# Port 5\npump /1I5R #switch to port 5, clockwise rotation\npump /1Q #query pump\npump /1?6 #report valve position\npump /1A600R #go to absolute position 600 (= pump 200 ul)\npump /1Q #query pump\npump /1? #report absolute plunger position (the plunger should be moving to 0)\nwait-min 1 #wait 1 minute\npump /1? #report absolute plunger position (the plunger should have finished moving)\n# Port 6\npump /1I6R #switch to port 6, clockwise rotation\npump /1Q #query pump\npump /1?6 #report valve position\npump /1A0R #go to absolute position 0 (= pump 200 ul)\npump /1Q #query pump\npump /1? #report absolute plunger position (the plunger should be moving to 0)\nwait-min 1 #wait 1 minute\npump /1? #report absolute plunger position (the plunger should have finished moving)\n#-------------------------------------------------------\n# Cycle 38\n# Fill the syringe\n#pump /1ZR #initialize pump\npump /1Q #query pump\npump /1? #report absolute plunger position\npump /1?6 #report valve position\nwait-min 1 #wait 1 minute\npump /1N0R #set step resolution: 0.01 mm\npump /1Q #query pump\npump /1? #report absolute plunger position (the plunger should be at 0)\npump /1?6 #report valve position\nwait 1000 #wait 1 second\npump /1V300R #choose speed: 300 steps/s (6000 ul/min)\npump /1Q #query pump\nwait 1000 #wait 1 second\npump /1O3R #go to port 3, counterclockwise rotation\npump /1Q #query pump\npump /1?6 #report valve position\nwait 1000 #wait 1 second\npump /1A3000R #go to absolute position 3000 (= draw 1 ml)\nwait 30000 #wait 30 seconds\npump /1Q #query pump\npump /1? #report absolute plunger position (the plunger should have finished moving)\n#pump /1?6 #report valve position\n# The sequential pumping begins\n# Port 1\npump /1O1R #switch to port 1, counterclockwise rotation\npump /1Q #query pump\npump /1?6 #report valve position\npump /1A2400R #go to absolute position 2400 (= pump 200 ul)\npump /1Q #query pump\npump /1? #report absolute plunger position (the plunger should be moving to 0)\nwait-min 1 #wait 1 minute\npump /1? #report absolute plunger position (the plunger should have finished moving)\n# Port 2\npump /1I2R #switch to port 2, clockwise rotation\npump /1Q #query pump\npump /1?6 #report valve position\npump /1A1800R #go to absolute position 1800 (= pump 200 ul)\npump /1Q #query pump\npump /1? #report absolute plunger position (the plunger should be moving to 0)\nwait-min 1 #wait 1 minute\npump /1? #report absolute plunger position (the plunger should have finished moving)\n# Port 4\npump /1I4R #switch to port 4, clockwise rotation\npump /1Q #query pump\npump /1?6 #report valve position\npump /1A1200R #go to absolute position 1200 (= pump 200 ul)\npump /1Q #query pump\npump /1? #report absolute plunger position (the plunger should be moving to 0)\nwait-min 1 #wait 1 minute\npump /1? #report absolute plunger position (the plunger should have finished moving)\n# Port 5\npump /1I5R #switch to port 5, clockwise rotation\npump /1Q #query pump\npump /1?6 #report valve position\npump /1A600R #go to absolute position 600 (= pump 200 ul)\npump /1Q #query pump\npump /1? #report absolute plunger position (the plunger should be moving to 0)\nwait-min 1 #wait 1 minute\npump /1? #report absolute plunger position (the plunger should have finished moving)\n# Port 6\npump /1I6R #switch to port 6, clockwise rotation\npump /1Q #query pump\npump /1?6 #report valve position\npump /1A0R #go to absolute position 0 (= pump 200 ul)\npump /1Q #query pump\npump /1? #report absolute plunger position (the plunger should be moving to 0)\nwait-min 1 #wait 1 minute\npump /1? #report absolute plunger position (the plunger should have finished moving)\n#-------------------------------------------------------\n# Cycle 39\n# Fill the syringe\n#pump /1ZR #initialize pump\npump /1Q #query pump\npump /1? #report absolute plunger position\npump /1?6 #report valve position\nwait-min 1 #wait 1 minute\npump /1N0R #set step resolution: 0.01 mm\npump /1Q #query pump\npump /1? #report absolute plunger position (the plunger should be at 0)\npump /1?6 #report valve position\nwait 1000 #wait 1 second\npump /1V300R #choose speed: 300 steps/s (6000 ul/min)\npump /1Q #query pump\nwait 1000 #wait 1 second\npump /1O3R #go to port 3, counterclockwise rotation\npump /1Q #query pump\npump /1?6 #report valve position\nwait 1000 #wait 1 second\npump /1A3000R #go to absolute position 3000 (= draw 1 ml)\nwait 30000 #wait 30 seconds\npump /1Q #query pump\npump /1? #report absolute plunger position (the plunger should have finished moving)\n#pump /1?6 #report valve position\n# The sequential pumping begins\n# Port 1\npump /1O1R #switch to port 1, counterclockwise rotation\npump /1Q #query pump\npump /1?6 #report valve position\npump /1A2400R #go to absolute position 2400 (= pump 200 ul)\npump /1Q #query pump\npump /1? #report absolute plunger position (the plunger should be moving to 0)\nwait-min 1 #wait 1 minute\npump /1? #report absolute plunger position (the plunger should have finished moving)\n# Port 2\npump /1I2R #switch to port 2, clockwise rotation\npump /1Q #query pump\npump /1?6 #report valve position\npump /1A1800R #go to absolute position 1800 (= pump 200 ul)\npump /1Q #query pump\npump /1? #report absolute plunger position (the plunger should be moving to 0)\nwait-min 1 #wait 1 minute\npump /1? #report absolute plunger position (the plunger should have finished moving)\n# Port 4\npump /1I4R #switch to port 4, clockwise rotation\npump /1Q #query pump\npump /1?6 #report valve position\npump /1A1200R #go to absolute position 1200 (= pump 200 ul)\npump /1Q #query pump\npump /1? #report absolute plunger position (the plunger should be moving to 0)\nwait-min 1 #wait 1 minute\npump /1? #report absolute plunger position (the plunger should have finished moving)\n# Port 5\npump /1I5R #switch to port 5, clockwise rotation\npump /1Q #query pump\npump /1?6 #report valve position\npump /1A600R #go to absolute position 600 (= pump 200 ul)\npump /1Q #query pump\npump /1? #report absolute plunger position (the plunger should be moving to 0)\nwait-min 1 #wait 1 minute\npump /1? #report absolute plunger position (the plunger should have finished moving)\n# Port 6\npump /1I6R #switch to port 6, clockwise rotation\npump /1Q #query pump\npump /1?6 #report valve position\npump /1A0R #go to absolute position 0 (= pump 200 ul)\npump /1Q #query pump\npump /1? #report absolute plunger position (the plunger should be moving to 0)\nwait-min 1 #wait 1 minute\npump /1? #report absolute plunger position (the plunger should have finished moving)\n#-------------------------------------------------------\n# Cycle 40\n# Fill the syringe\n#pump /1ZR #initialize pump\npump /1Q #query pump\npump /1? #report absolute plunger position\npump /1?6 #report valve position\nwait-min 1 #wait 1 minute\npump /1N0R #set step resolution: 0.01 mm\npump /1Q #query pump\npump /1? #report absolute plunger position (the plunger should be at 0)\npump /1?6 #report valve position\nwait 1000 #wait 1 second\npump /1V300R #choose speed: 300 steps/s (6000 ul/min)\npump /1Q #query pump\nwait 1000 #wait 1 second\npump /1O3R #go to port 3, counterclockwise rotation\npump /1Q #query pump\npump /1?6 #report valve position\nwait 1000 #wait 1 second\npump /1A3000R #go to absolute position 3000 (= draw 1 ml)\nwait 30000 #wait 30 seconds\npump /1Q #query pump\npump /1? #report absolute plunger position (the plunger should have finished moving)\n#pump /1?6 #report valve position\n# The sequential pumping begins\n# Port 1\npump /1O1R #switch to port 1, counterclockwise rotation\npump /1Q #query pump\npump /1?6 #report valve position\npump /1A2400R #go to absolute position 2400 (= pump 200 ul)\npump /1Q #query pump\npump /1? #report absolute plunger position (the plunger should be moving to 0)\nwait-min 1 #wait 1 minute\npump /1? #report absolute plunger position (the plunger should have finished moving)\n# Port 2\npump /1I2R #switch to port 2, clockwise rotation\npump /1Q #query pump\npump /1?6 #report valve position\npump /1A1800R #go to absolute position 1800 (= pump 200 ul)\npump /1Q #query pump\npump /1? #report absolute plunger position (the plunger should be moving to 0)\nwait-min 1 #wait 1 minute\npump /1? #report absolute plunger position (the plunger should have finished moving)\n# Port 4\npump /1I4R #switch to port 4, clockwise rotation\npump /1Q #query pump\npump /1?6 #report valve position\npump /1A1200R #go to absolute position 1200 (= pump 200 ul)\npump /1Q #query pump\npump /1? #report absolute plunger position (the plunger should be moving to 0)\nwait-min 1 #wait 1 minute\npump /1? #report absolute plunger position (the plunger should have finished moving)\n# Port 5\npump /1I5R #switch to port 5, clockwise rotation\npump /1Q #query pump\npump /1?6 #report valve position\npump /1A600R #go to absolute position 600 (= pump 200 ul)\npump /1Q #query pump\npump /1? #report absolute plunger position (the plunger should be moving to 0)\nwait-min 1 #wait 1 minute\npump /1? #report absolute plunger position (the plunger should have finished moving)\n# Port 6\npump /1I6R #switch to port 6, clockwise rotation\npump /1Q #query pump\npump /1?6 #report valve position\npump /1A0R #go to absolute position 0 (= pump 200 ul)\npump /1Q #query pump\npump /1? #report absolute plunger position (the plunger should be moving to 0)\nwait-min 1 #wait 1 minute\npump /1? #report absolute plunger position (the plunger should have finished moving)\n#-------------------------------------------------------"
  out "Command running:":string
  out "Serial port data":string
  out "Elapsed Time":dbl caption="Elapsed Time (s)"
  in  "Time Units":u16(ring)=1 items=["Seconds", "Minutes", "Hours"]
  in  "Time Offset":dbl caption="Set Start Time (s)"
  in  "Reset":bool
  in  "Auto Reset":bool
  in  "integration time":u32(slide) max=2 step=1 scale=0.0..2.0
  in  "Interrupt scan":bool
  out "Absolute plunger position vs time":cluster{"Y data in":dbl[], "X data in":dbl[]}[](graph)
  out "Valve position vs time":cluster{"Y data in":dbl[], "X data in":dbl[]}[](graph)
  out "Is on":dbl format="%.2e"
  out "Id on":dbl format="%.2e"
  out "Ig on":dbl format="%.2e"
  out "Ion vs time":cluster{"Y data in":dbl[], "X data in":dbl[]}[](graph)
  out "Ioff vs time":cluster{"Y data in":dbl[], "X data in":dbl[]}[](graph)
  out "Ig min":dbl format="%.2e"
  out "Id min":dbl format="%.2e"
  out "Is min":dbl format="%.2e"
  out "Is off":dbl format="%.2e"
  out "Id off":dbl format="%.2e"
  out "Ig off":dbl format="%.2e"
  in  "Integration time (long)":dbl=0.32 min=0.04 max=2.0 step=0.02 format="%.2f"
  in  "Integration time (short)":dbl=0.0019 min=8e-05 max=0.0019 step=8e-05 format="%^.0e"
  in  "Gate: Compliance":dbl=0.001 format="%.8f"
  in  "Drain: Compliance":dbl=0.001 format="%.8f"
  in  "Hard stop pump":bool
  in  "Halt pump":bool
  in  "Interrupt program":bool
  in  "Suffix (script)":string="step_1_up-H2O_initial_script.txt"
  in  "Filename (variable part)":string="step_1_up-H2O_initial_"
  in  "Plot output curve extrema vs time":bool
  in  "Plot transfer curve extrema vs time":bool=TRUE
  in  "Plot sample extrema vs time":bool
  out "I vs time (Bias Stress)":cluster{"Y data in":dbl[], "X data in":dbl[]}[](graph)
  out "Vp1":dbl format="%.2e"
  out "Vp2":dbl format="%.2e"
  in  "Sample I - Probe 4 (Disabled)":u32(ring)=3 items=["SMU1  ", "SMU2  ", "SMU3  ", "SMU4  ", "SMU5  ", "SMU6  ", "VSU1  ", "VSU2  "]
  in  "Sample I - Source/Common":u32(ring) items=["SMU1  ", "SMU2  ", "SMU3  ", "SMU4  ", "SMU5  ", "SMU6  ", "VSU1  ", "VSU2  "]
  in  "Sample I - Probe 3 (Disabled)":u32(ring)=2 items=["SMU1  ", "SMU2  ", "SMU3  ", "SMU4  ", "SMU5  ", "SMU6  ", "VSU1  ", "VSU2  "]
  in  "Sample I - Drain/Gate":u32(ring)=1 items=["SMU1  ", "SMU2  ", "SMU3  ", "SMU4  ", "SMU5  ", "SMU6  ", "VSU1  ", "VSU2  "]
  in  "Sample - Probe 4":u32(ring)=3 items=["SMU1  ", "SMU2  ", "SMU3  ", "SMU4  ", "SMU5  ", "SMU6  ", "VSU1  ", "VSU2  "]
  in  "Sample - Source/Common":u32(ring) items=["SMU1  ", "SMU2  ", "SMU3  ", "SMU4  ", "SMU5  ", "SMU6  ", "VSU1  ", "VSU2  "]
  in  "Sample - Gate":u32(ring)=2 items=["SMU1  ", "SMU2  ", "SMU3  ", "SMU4  ", "SMU5  ", "SMU6  ", "VSU1  ", "VSU2  "]
  in  "Sample - Drain":u32(ring)=1 items=["SMU1  ", "SMU2  ", "SMU3  ", "SMU4  ", "SMU5  ", "SMU6  ", "VSU1  ", "VSU2  "]
  in  "VSU2 Stress - Source/Common":u32(ring) items=["SMU1  ", "SMU2  ", "SMU3  ", "SMU4  ", "SMU5  ", "SMU6  ", "VSU1  "]
  in  "Stress I - Source/Common":u32(ring) items=["SMU1  ", "SMU2  ", "SMU3  ", "SMU4  ", "SMU5  ", "SMU6  ", "VSU1  ", "VSU2  "]
  in  "Stress I - Drain/Gate":u32(ring)=1 items=["SMU1  ", "SMU2  ", "SMU3  ", "SMU4  ", "SMU5  ", "SMU6  ", "VSU1  ", "VSU2  "]
  in  "Stress V - Source/Common":u32(ring) items=["SMU1  ", "SMU2  ", "SMU3  ", "SMU4  ", "SMU5  ", "SMU6  ", "VSU1  ", "VSU2  "]
  in  "Stress V - Gate":u32(ring)=2 items=["SMU1  ", "SMU2  ", "SMU3  ", "SMU4  ", "SMU5  ", "SMU6  ", "VSU1  ", "VSU2  "]
  in  "Stress V - Drain":u32(ring)=1 items=["SMU1  ", "SMU2  ", "SMU3  ", "SMU4  ", "SMU5  ", "SMU6  ", "VSU1  ", "VSU2  "]
  in  "FPP - Source":u32(ring)=6 items=["SMU1  ", "SMU2  ", "SMU3  ", "SMU4  ", "SMU5  ", "SMU6  ", "VSU1  ", "VSU2  "]
  in  "FPP - Probe 2":u32(ring)=3 items=["SMU1  ", "SMU2  ", "SMU3  ", "SMU4  ", "SMU5  ", "SMU6  ", "VSU1  ", "VSU2  "]
  in  "FPP - Probe 1":u32(ring) items=["SMU1  ", "SMU2  ", "SMU3  ", "SMU4  ", "SMU5  ", "SMU6  ", "VSU1  ", "VSU2  "]
  in  "FPP - Gate":u32(ring)=2 items=["SMU1  ", "SMU2  ", "SMU3  ", "SMU4  ", "SMU5  ", "SMU6  ", "VSU1  ", "VSU2  "]
  in  "FPP - Drain":u32(ring)=1 items=["SMU1  ", "SMU2  ", "SMU3  ", "SMU4  ", "SMU5  ", "SMU6  ", "VSU1  ", "VSU2  "]
  in  "Pulsed Stress V - Vextra":u32(ring)=6 items=["SMU1  ", "SMU2  ", "SMU3  ", "SMU4  ", "SMU5  ", "SMU6  ", "VSU1  ", "VSU2  "]
  in  "Pulsed Stress V - Probe 4":u32(ring)=3 items=["SMU1  ", "SMU2  ", "SMU3  ", "SMU4  ", "SMU5  ", "SMU6  ", "VSU1  ", "VSU2  "]
  in  "Pulsed Stress V - Source/Common":u32(ring) items=["SMU1  ", "SMU2  ", "SMU3  ", "SMU4  ", "SMU5  ", "SMU6  ", "VSU1  ", "VSU2  "]
  in  "Pulsed Stress V - Gate":u32(ring)=2 items=["SMU1  ", "SMU2  ", "SMU3  ", "SMU4  ", "SMU5  ", "SMU6  ", "VSU1  ", "VSU2  "]
  in  "Pulsed Stress V - Drain":u32(ring)=1 items=["SMU1  ", "SMU2  ", "SMU3  ", "SMU4  ", "SMU5  ", "SMU6  ", "VSU1  ", "VSU2  "]
  in  "Transfer/Output - Probe 4":u32(ring)=3 items=["SMU1  ", "SMU2  ", "SMU3  ", "SMU4  ", "SMU5  ", "SMU6  ", "VSU1  ", "VSU2  "]
  in  "Transfer/Output - Source/Common":u32(ring) items=["SMU1  ", "SMU2  ", "SMU3  ", "SMU4  ", "SMU5  ", "SMU6  ", "VSU1  ", "VSU2  "]
  in  "Transfer/Output - Gate":u32(ring)=2 items=["SMU1  ", "SMU2  ", "SMU3  ", "SMU4  ", "SMU5  ", "SMU6  ", "VSU1  ", "VSU2  "]
  in  "Transfer/Output - Drain":u32(ring)=1 items=["SMU1  ", "SMU2  ", "SMU3  ", "SMU4  ", "SMU5  ", "SMU6  ", "VSU1  ", "VSU2  "]
  in  "Gate Range\nmode":u16(ring) items=["Auto", "Limited", "Fixed"]
  in  "Gate Range":u8(slide)=3 max=11 scale=0.0..11.0
  in  "Source/Drain\nRange mode":u16(ring) items=["Auto", "Limited", "Fixed"]
  in  "Source/Drain Range":u8(slide)=3 max=11 scale=0.0..11.0
  in  "Panel Controls":T1={"Emergency Stop"=refnum, "TransGraph Max"=1e-05, "Text/Graph (text=false)"=TRUE} {"TransGraph Max" format="%.2e"}
  in  "Panel Controls 2":T2={"Emergency Stop"=refnum, "TransGraph Max"=1e-05, "Text/Graph (text=false)"=TRUE, "TransGraph Min"=1e-11} {"TransGraph Min" format="%.2e"; "TransGraph Max" format="%.2e"}
  in  "Probe 4":cluster{"on/off":bool, "Voltage":dbl} {"Voltage" min=-100.0 max=100.0 format="%.2f"}
  in  "Full Reset":bool
  in  "Standby":T3
  out "error out":errorcluster
  in  "Delay before read (ms)":u32=1000
  in  "byte count":u32=64
  in  "Serial End Mode for Reads":u16(ring)=2 items=["None", "LastBit", "TermChar"]
  in  "Timeout (ms)":u32=10000
  in  "Enable Termination\nChar (T)":bool=TRUE
  in  "Termination char\n(0xA = '\\n' = LF)\n(0xD = '\\r' = CR)":u8=13 format="%.0x"
  in  "flow control":u16(ring) items=["None"=0, "XON/XOFF"=1, "RTS/CTS"=2, "DTR/DSR"=4]
  in  "stop bits":u16(ring)=10 items=["1.0"=10, "1.5"=15, "2.0"=20]
  in  "parity":u16(ring) items=["None", "Odd", "Even", "Mark", "Space"]
  in  "data bits":u16=8 min=5 max=8 step=1
  in  "VISA resource name":refnum<visa-resource-name>="COM6"
  in  "baud rate":u32=9600
  out "Timings Indicator":T4 {"integration time" scale=0.0..2.0}
  in  "Timings (overwritten by the Front Panel)":T5={"integration time"=0, "Short/Long integration time"=0.00064, "hold time (sec)"=0.0, "delay time (sec)"=0.0, "Step Time (0 disables)"=0.0, "sweep method"=0, "Pulse period"=0.005, "Base voltage"=0.0, "Pulse width"=0.0005} {"Pulse width" min=0.0005 max=0.1 step=0.0001 format="%.4f"; "Base voltage" format="%^.4e"; "Pulse period" min=0.005 max=1.0 step=0.0001 format="%.4f"; "sweep method" items=["Continuous", "Pulsed"]; "Step Time (0 disables)" format="%.2f"; "delay time (sec)" format="%.4f"; "hold time (sec)" format="%.4f"; "Short/Long integration time" format="%^.0e"; "integration time" scale=0.0..2.0}
  out "Probe 4 Indicator":cluster{"on/off":bool, "Voltage":dbl} {"Voltage" min=-100.0 max=100.0 format="%.2f"}
  in  "VISA resource name in":refnum<visa-resource-name>="GPIB0::14::INSTR"
  in  "Gate":T6={"Gate Start"=0.0, "Gate Stop"=2.0, "Gate Step (linear only)"=1.0, "Gate Compliance"=0.0001, "Gate PComp"=0.0, "Range mode"=0, "Range"=6} {"Range" max=11 scale=0.0..11.0; "Range mode" items=["Auto", "Limited", "Fixed"]; "Gate PComp" format="%^.2e"; "Gate Compliance" format="%^.2e"; "Gate Step (linear only)" format="%^.4e"; "Gate Stop" format="%^.4e"; "Gate Start" format="%^.4e"}
  in  "Drain 2":T7={"Drain Start"=0.0, "Drain Stop"=2.0, "Drain Compliance"=0.0001, "Drain Step"=1.0, "Drain PComp"=0.0, "Range mode"=0, "Range"=6} {"Range" max=11 scale=0.0..11.0; "Range mode" items=["Auto", "Limited", "Fixed"]; "Drain PComp" format="%^.2e"; "Drain Step" format="%^.4e"; "Drain Compliance" format="%^.2e"; "Drain Stop" format="%^.4e"; "Drain Start" format="%^.4e"}
  # "Syntax:\nitime [s|m|l] time(sec): [s|m|l] determines the integration time setting (small|medium|long) and time sets the value.\nNOTE: The value of the integration time has to be within the range allowed by its category (s|m|l), otherwise, the closest value will be used. (e.g. if the category is set to short but the time value is very long, the actual value used will be the maximum short integration time.\nIntegration times:\n    Short: Default: 640 us. Range: 8E-5 - 1.92E-3 seconds.\n    Medium: Fixed at 1 NPL cycle (0.02 seconds).\n    Long: Default: 16 NPL cycles (0.32 seconds). Range: 2-100 NPL cycles (0.04 seconds - 2 seconds).\ngaterangemode [a|l|f]\ndrainrangemode [a|l|f]\npulsed [on|off] PulsePeriod(sec) PulseBaseVoltage PulseONWidth(sec)\nstandby [on l off]\nwait NumMilliseconds\nwait-min NumMinutes\n# texthere = comment\nProbe4 [ON|OFF] Voltage\ntransfer [s|d] VgStart VgStop VgStep VdStart VdStop VdStep\noutput [s|d] VgStart VgStop VgStep VdStart VdStop VdStep\nsample Vg Vd NumSamples Time(s) SampleInterval(s)\nsamplei Idg NumSamples Time(s) SampleInterval(s) VDGcompliance\n100 samples is approximately 13 seconds with medium integration\n# If in doubt use SampleInterval(s) = 0.004\n    NOTE: When doing bias stress measurements, it is best to set the Time Units to \"Seconds\", as the \"sample\" command has been configured to give the output to seconds.\nstressV VG VD IGcompliance IDcompliance Duration(sec)\nstressI IDG VDGcompliance Duration(sec)\nvsu2pulse Bias Duration(s)\npulsedstressV [s|d] VEstop VgON VgOFF Period(s) PulseONwidth(s) Vd\nsample-fpp Vg Vd NumSamples Time\nresample-fpp Vg Vd\ntransfer-fpp [s|d] VgStart VgStop VgStep VdStart VdStop VdStep\noutput-fpp [s|d] VgStart VgStop VgStep VdStart VdStop VdStep\nserial SerialPortCommand\npump SerialPortCommand for the SPM pump\n\nSPM Pump Syntax (<x>: pump number, use 1 if only one pump):\nif the command syntax contains [R], then append the letter R to the command\n/<x>Q: query (a query command should follow each command)\n/<x>Z[R] or /<x>Y[R]: initialize pump\n/<x>N<n>[R] (<n>=0,1): <0> (<1>) microstep 0.01 mm (0.00125 mm) resolution\n/<x>I<n> (<n>=0-6): turn to port number n (clockwise)\n/<x>O<n> (<n>=0-6): turn to port number n (counterclockwise)\n/<x>X: Re-execute last command string\n/<x>G<n>[R] (<n>=0-60000): repeat command sequence (default: 0, 0=loop forever)\n/<x>g: Mark the start of a repeat sequence (max = 10)\n/<x>M<n>[R] (<n>=0-86400000): delay command execution by n milliseconds\n/<x>H: Halt; Pause the sequence after finishing the current move\n/<x>T: Hardstop; Interrupt the current move and suppress it from the sequence\n/<x>A<n>[R] (<n>=0-3000 with N=0, 0-24000 with N=1): absolute position\n/<x>P<n>[R] (<n>=0-3000 with N=0, 0-24000 with N=1): relative pickup\n/<x>D<n>[R] (<n>=0-3000 with N=0, 0-24000 with N=1): relative dispense\n/<x>V<n>[R] (<n>=1-1600 default: 150): set peak speed (pulses/sec)\nNOTE: The lowest speed limit is 1 pulse/sec, not 5, as the manual states.\n/<x>S<n>[R] (<n>=10-40 default: 22): set speed (NOT in pulses/sec, look in manual)\nNOTE: When controlled with absolute position, one does not need to pay special attention to the syringe that is mounted on the pump.\nWithdraw from lower stage (ports 3, 5), dispense from higher stage (ports 2, 4, 6).\nConnect Port 1 to waste."
  # "Time"
  # "1\n2\n3\n4\n5\n6\n7\n8\n9\n10\n11\n12\n13\n14\n15\n16\n17\n18\n19\n20"
  # "Serial port settings"
  # "SMUs"
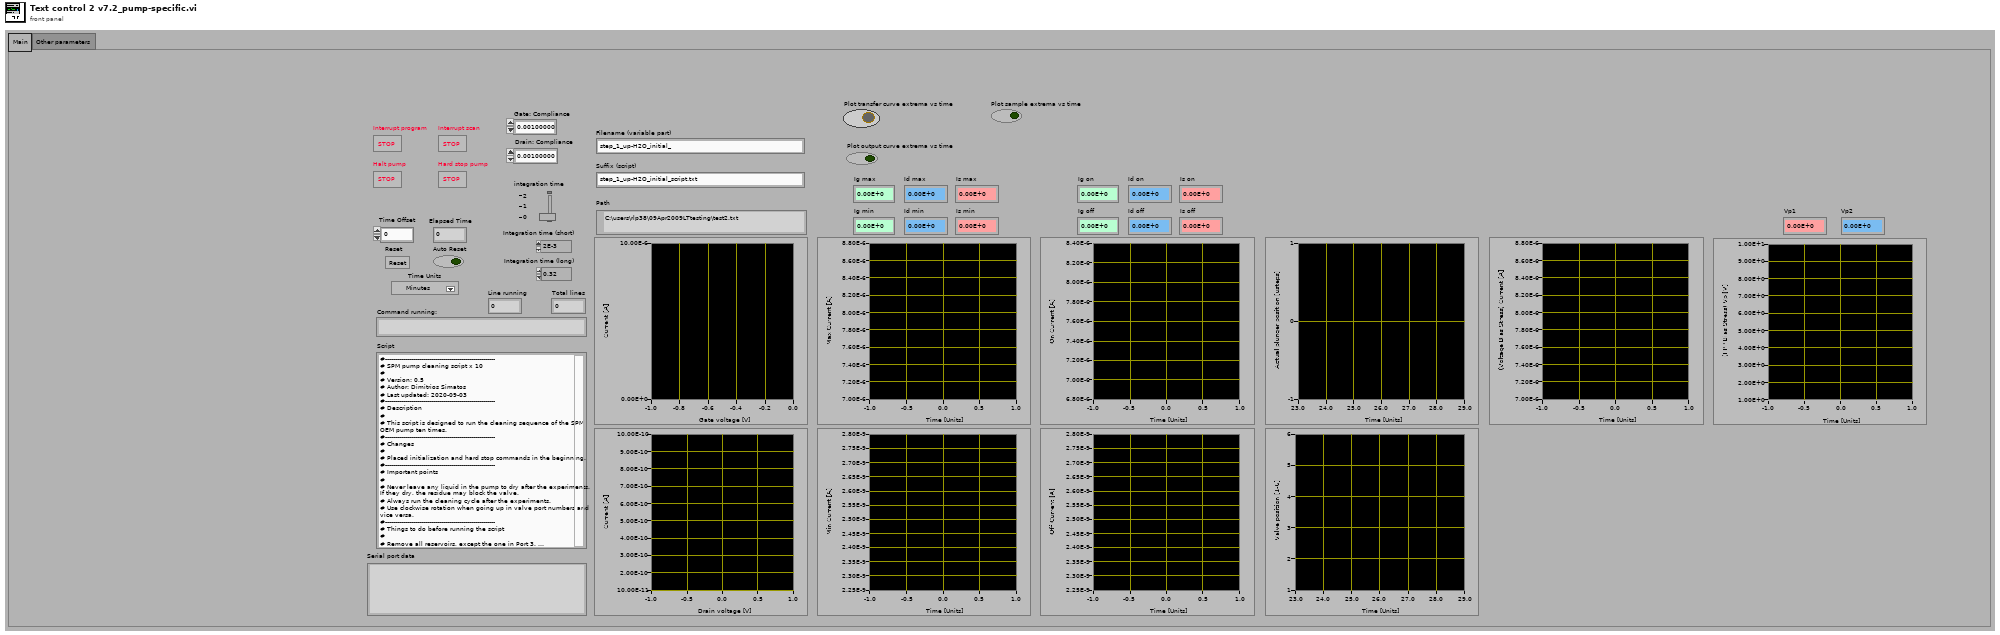
[diagram p1: front panel]
types:
  T1 = cluster{"Emergency Stop":refnum<vi>, "TransGraph Max":dbl, "Text/Graph (text=false)":bool}
  T2 = cluster{"Emergency Stop":refnum<vi>, "TransGraph Max":dbl, "Text/Graph (text=false)":bool, "TransGraph Min":dbl}
  T3 = cluster{"Gate Standby":bool, "Drain Standby":bool}
  T4 = cluster{"Short/Long integration time":dbl, "hold time (sec)":dbl, "delay time (sec)":dbl, "Step Time (0 disables)":dbl, "sweep method":u16, "Pulse period":dbl, "Base voltage":dbl, "Pulse width":dbl, "integration time":u32}
  T5 = cluster{"integration time":u32, "Short/Long integration time":dbl, "hold time (sec)":dbl, "delay time (sec)":dbl, "Step Time (0 disables)":dbl, "sweep method":u16, "Pulse period":dbl, "Base voltage":dbl, "Pulse width":dbl}
  T6 = cluster{"Gate Start":dbl, "Gate Stop":dbl, "Gate Step (linear only)":dbl, "Gate Compliance":dbl, "Gate PComp":dbl, "Range mode":u16, "Range":u8}
  T7 = cluster{"Drain Start":dbl, "Drain Stop":dbl, "Drain Compliance":dbl, "Drain Step":dbl, "Drain PComp":dbl, "Range mode":u16, "Range":u8}
  T8 = enum16{"open", "replace", "create", "open or create", "replace or create", "replace or create with confirmation"}
  T9 = cluster{"V2 Start":dbl, "V2 Step":dbl, "Number of points":i32}
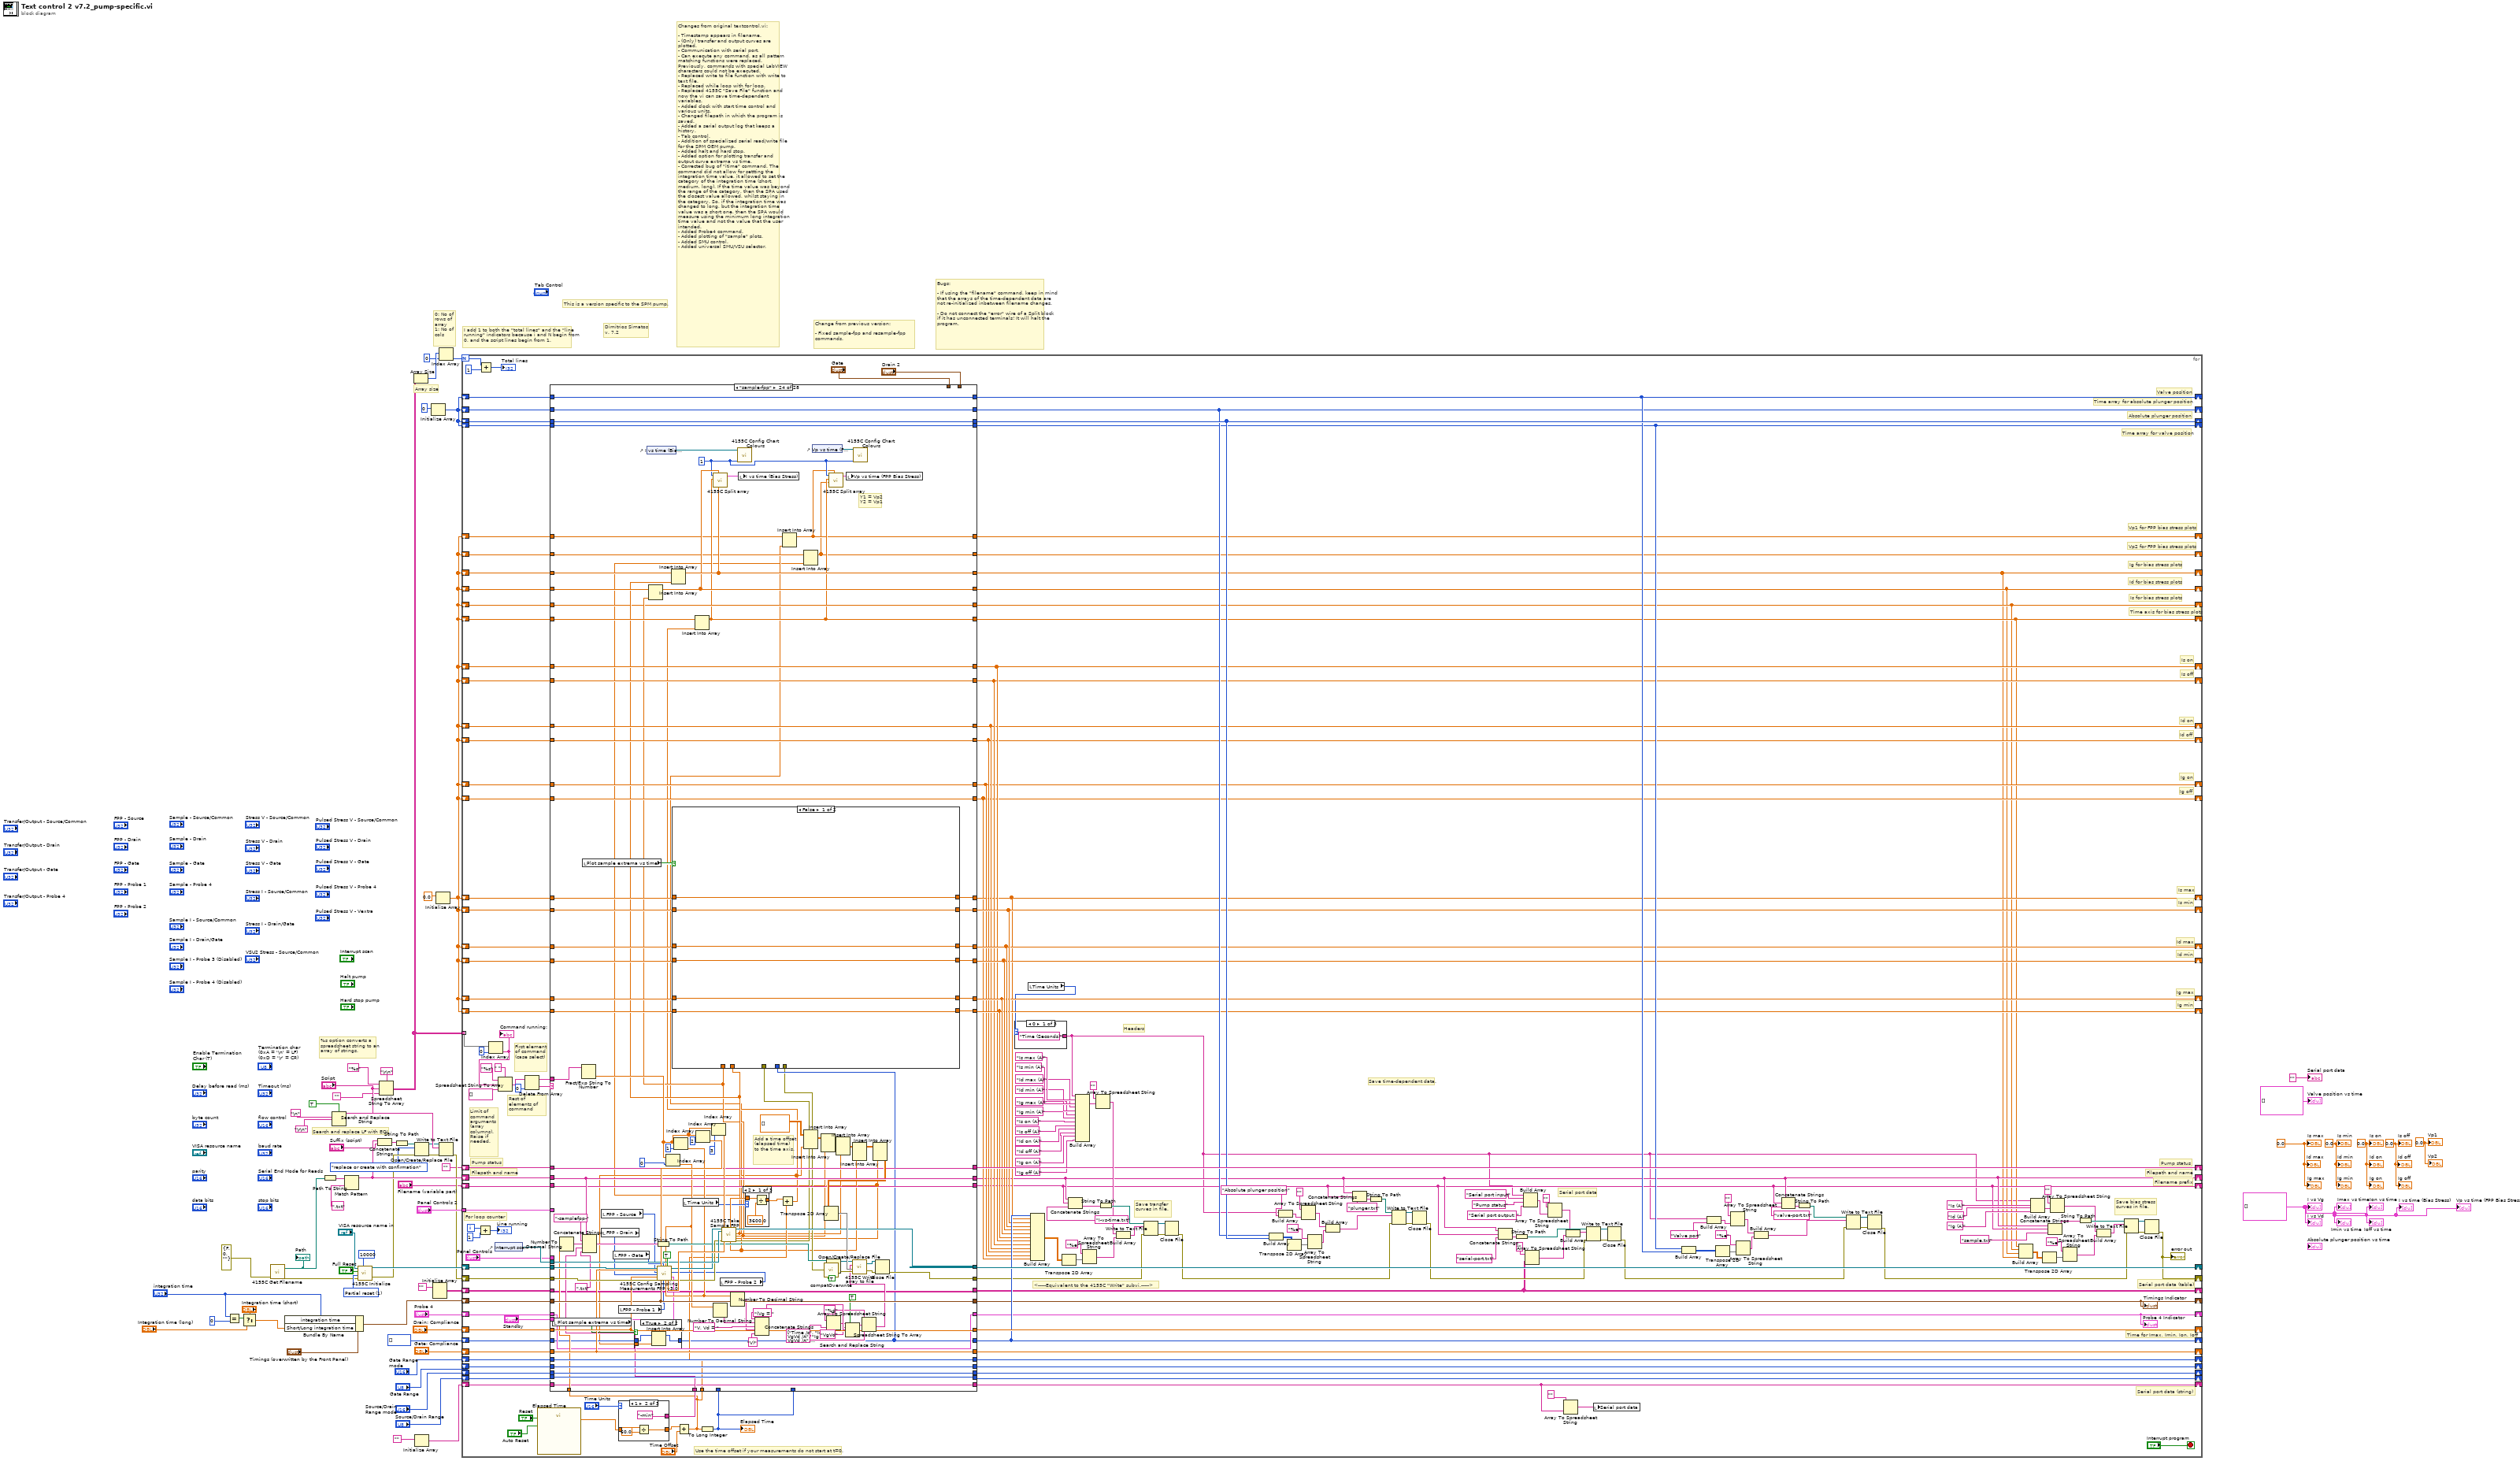
[diagram p0: block diagram]
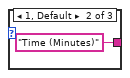
[diagram p2: hidden frame]
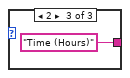
[diagram p3: hidden frame]
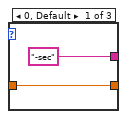
[diagram p4: hidden frame]
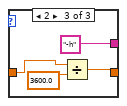
[diagram p5: hidden frame]
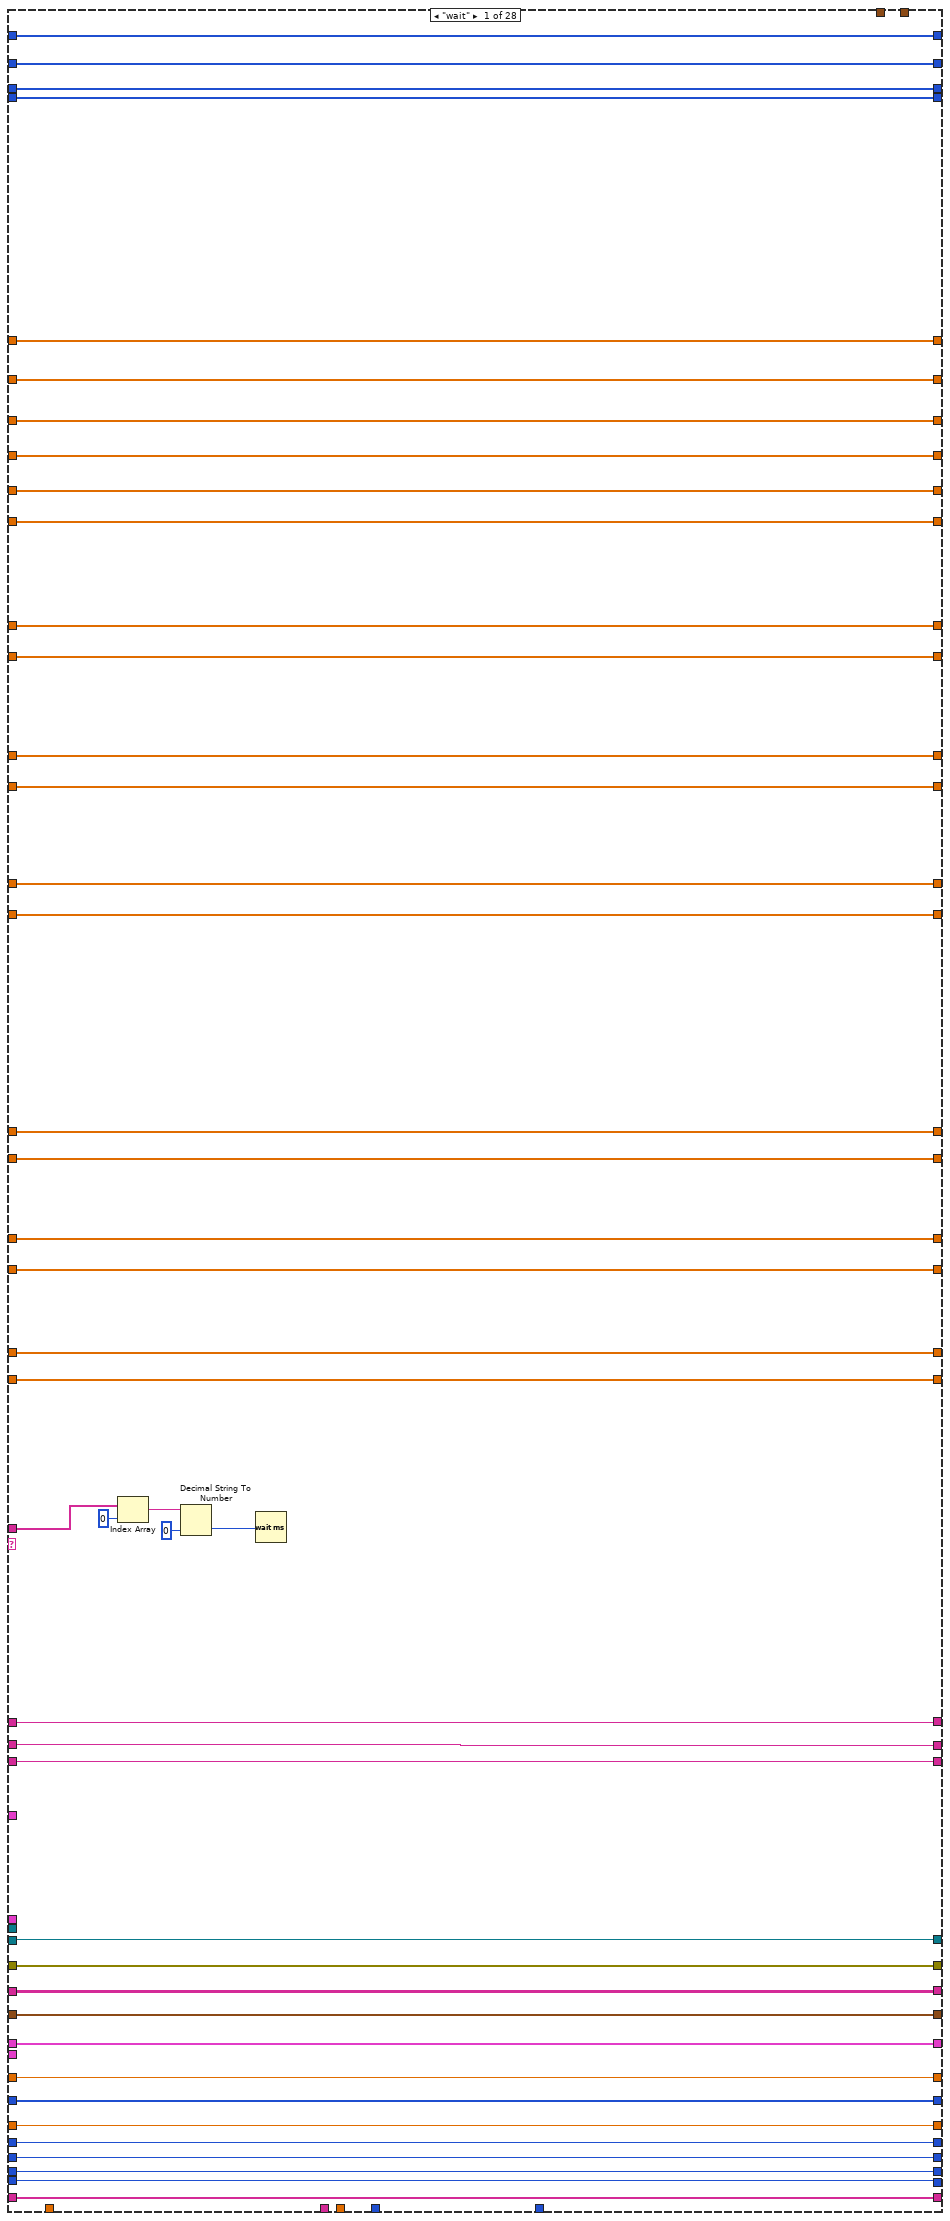
[diagram p6: hidden frame]
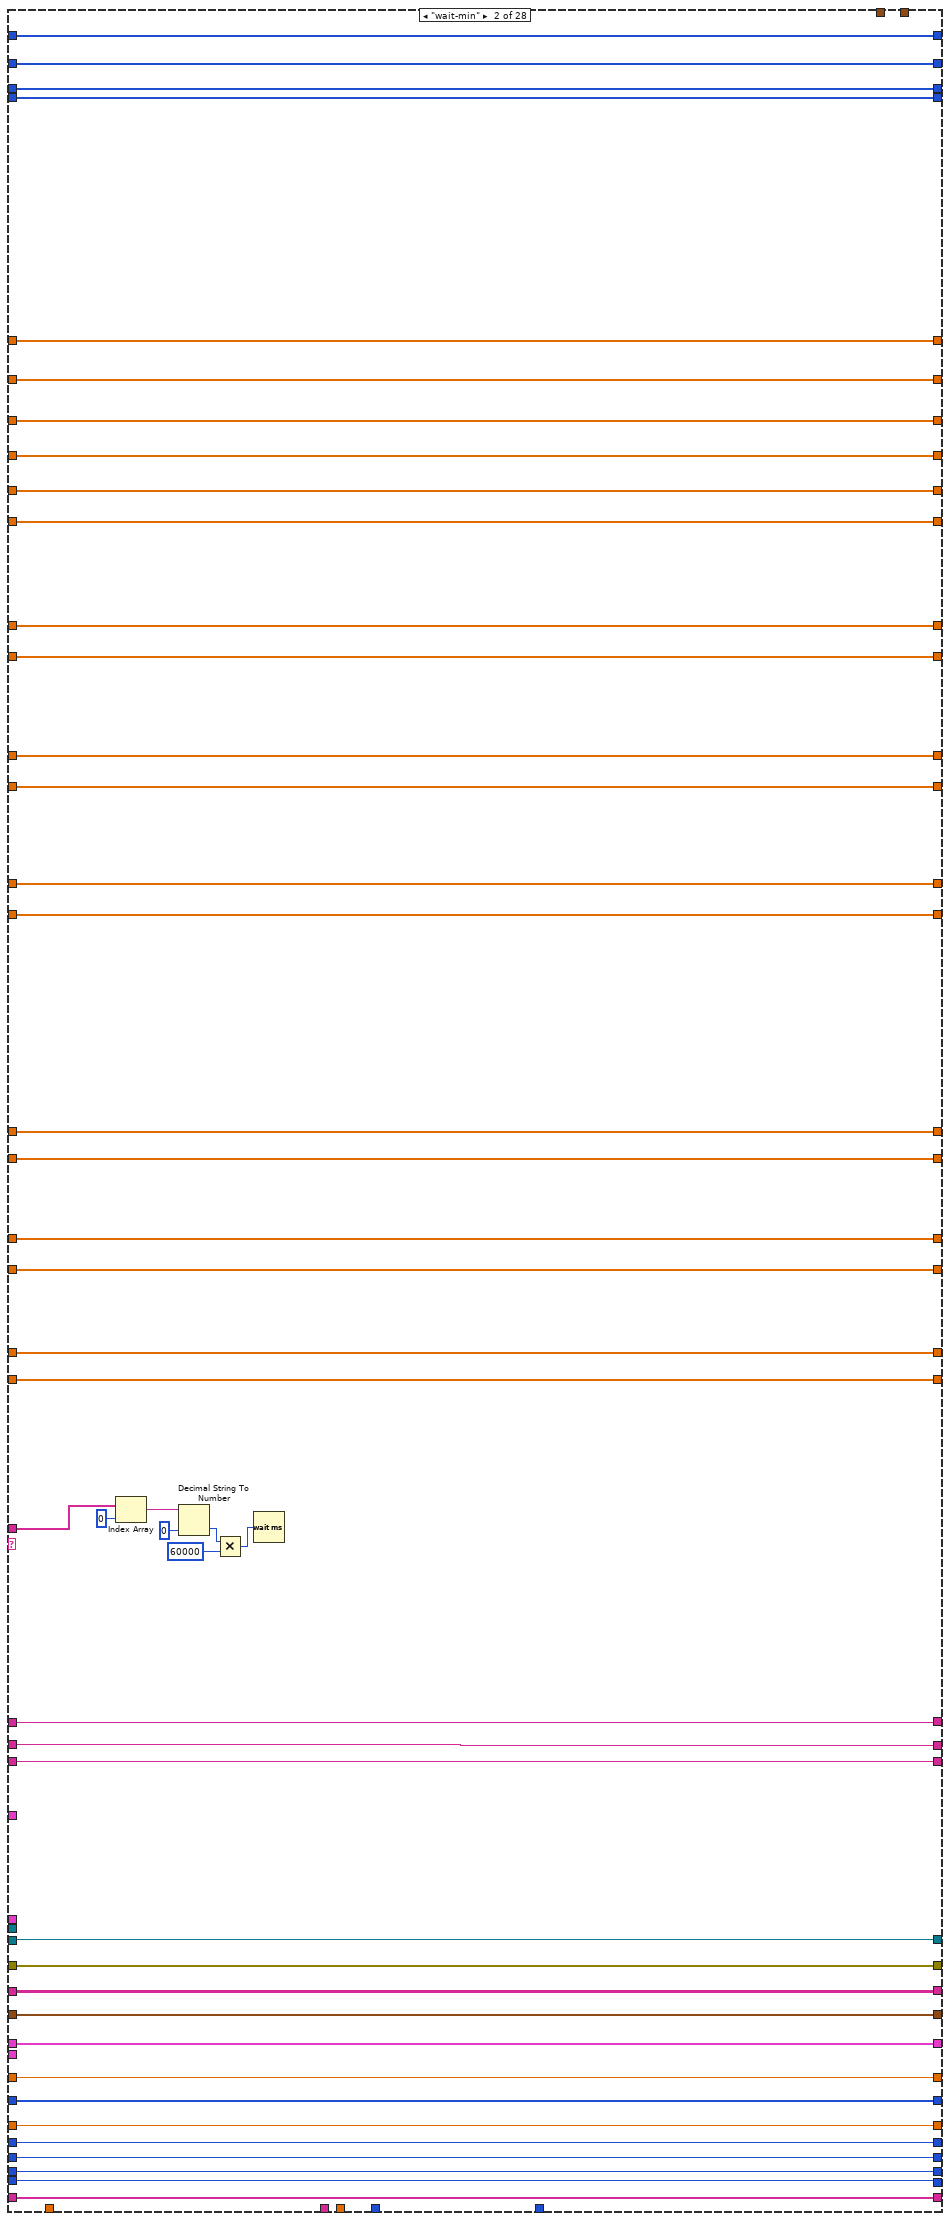
[diagram p7: hidden frame]
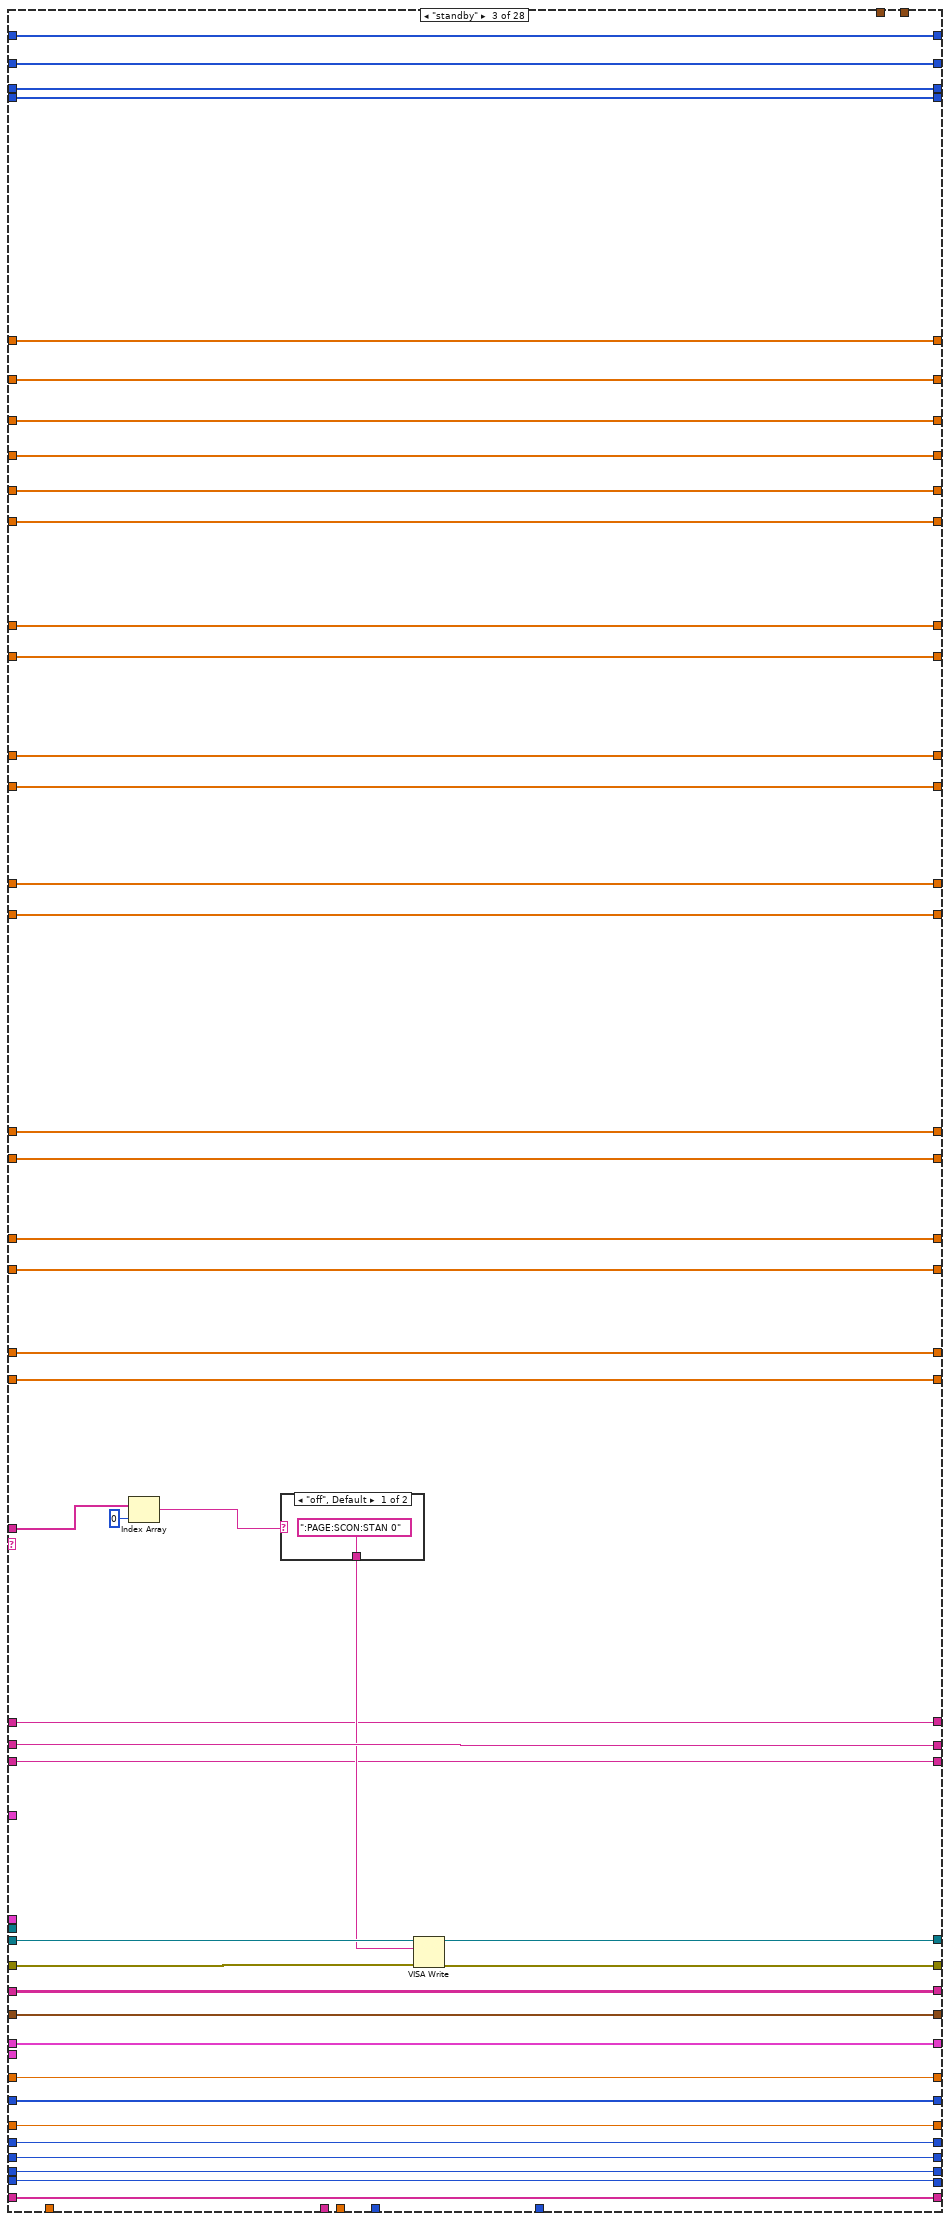
[diagram p8: hidden frame]
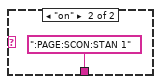
[diagram p9: hidden frame]
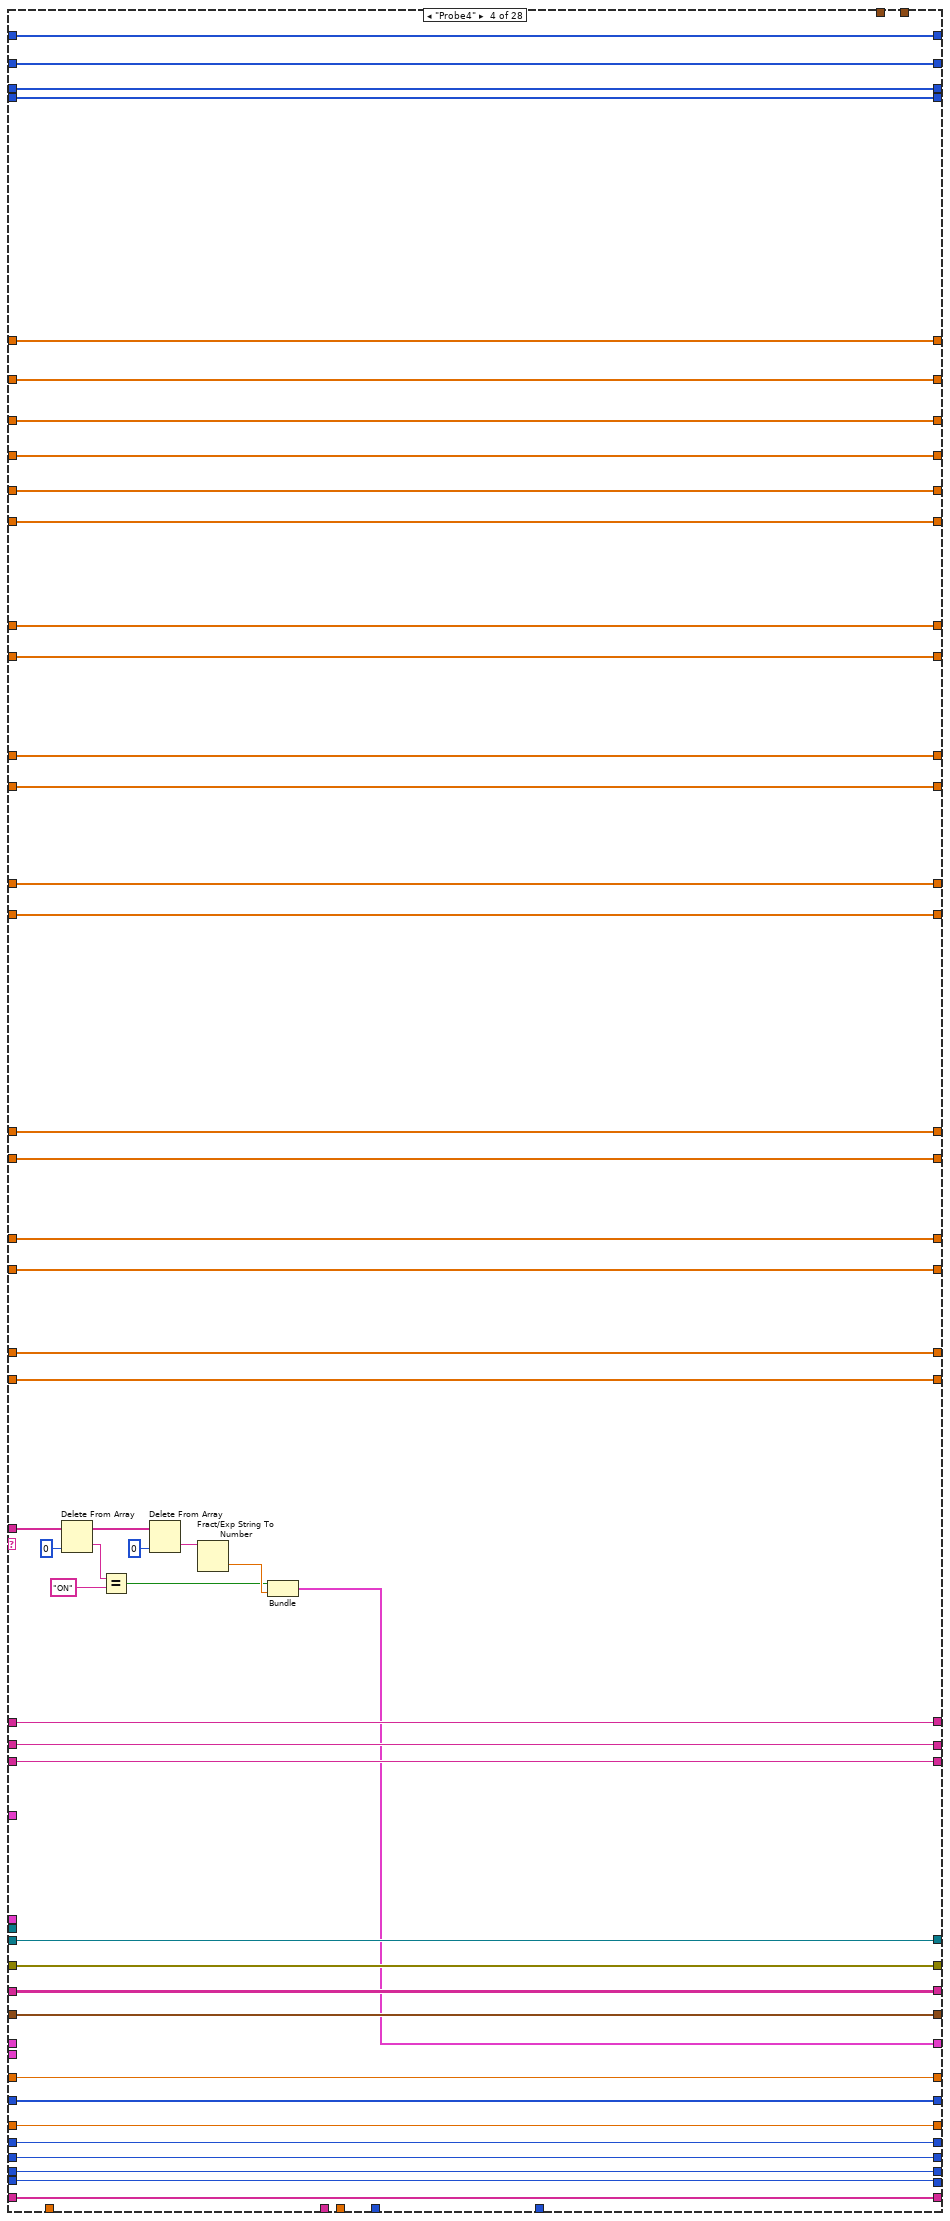
[diagram p10: hidden frame]
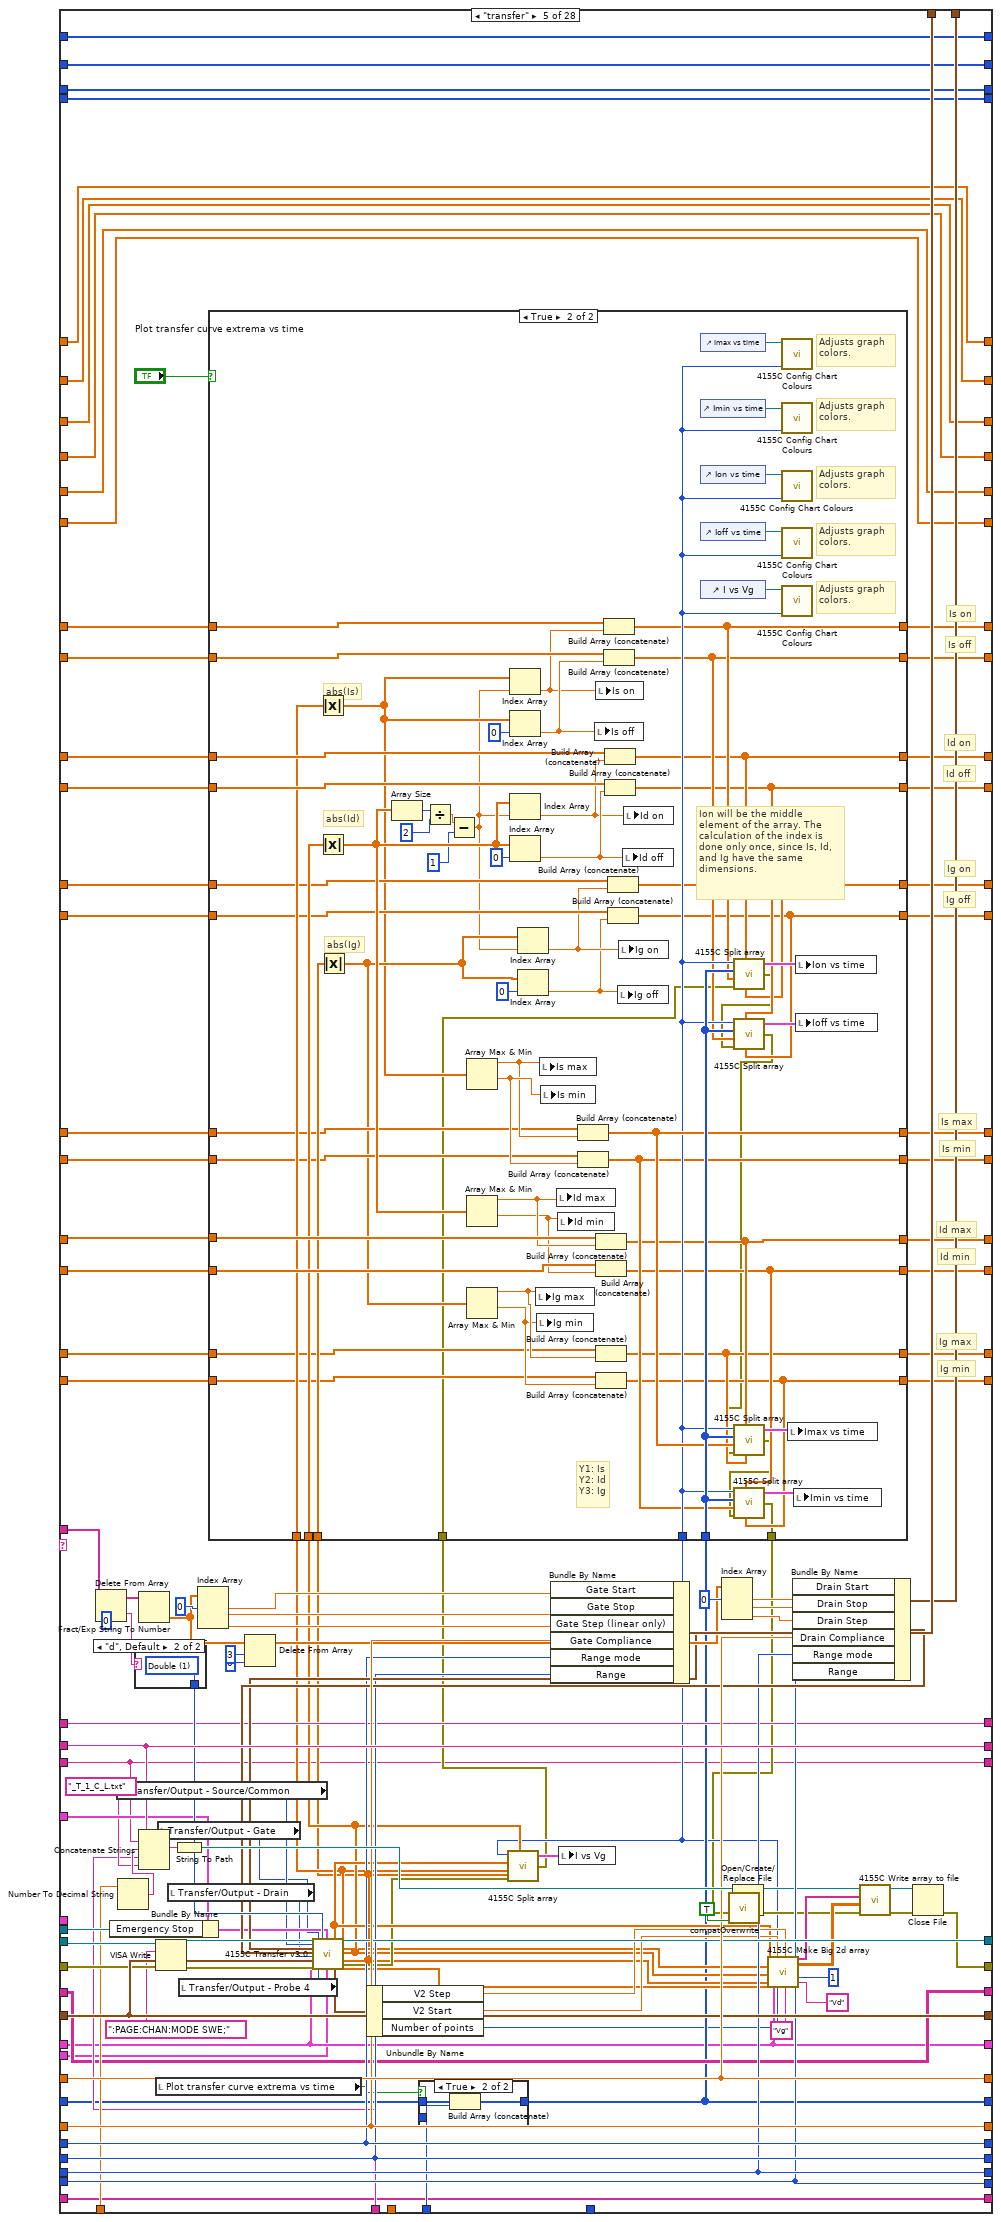
[diagram p11: hidden frame]
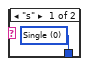
[diagram p14: hidden frame]
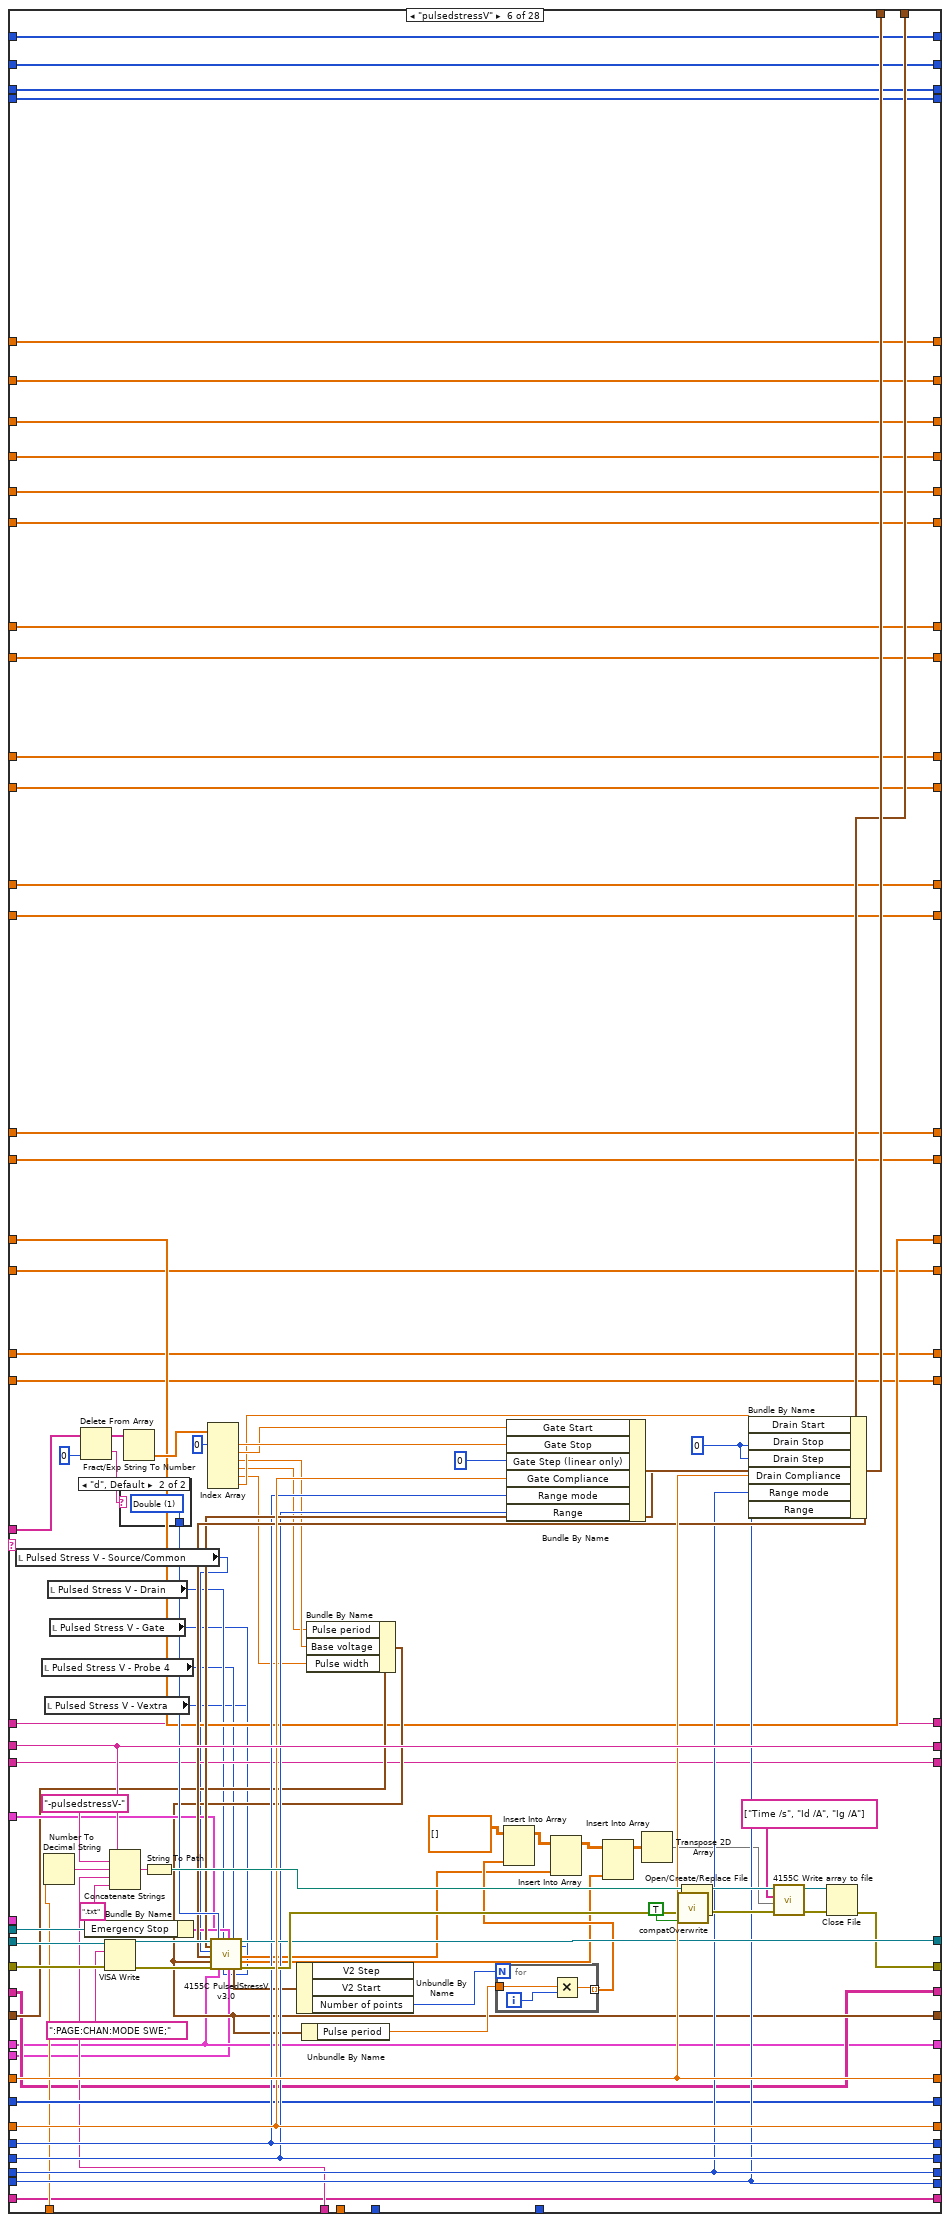
[diagram p15: hidden frame]
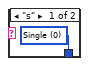
[diagram p16: hidden frame]
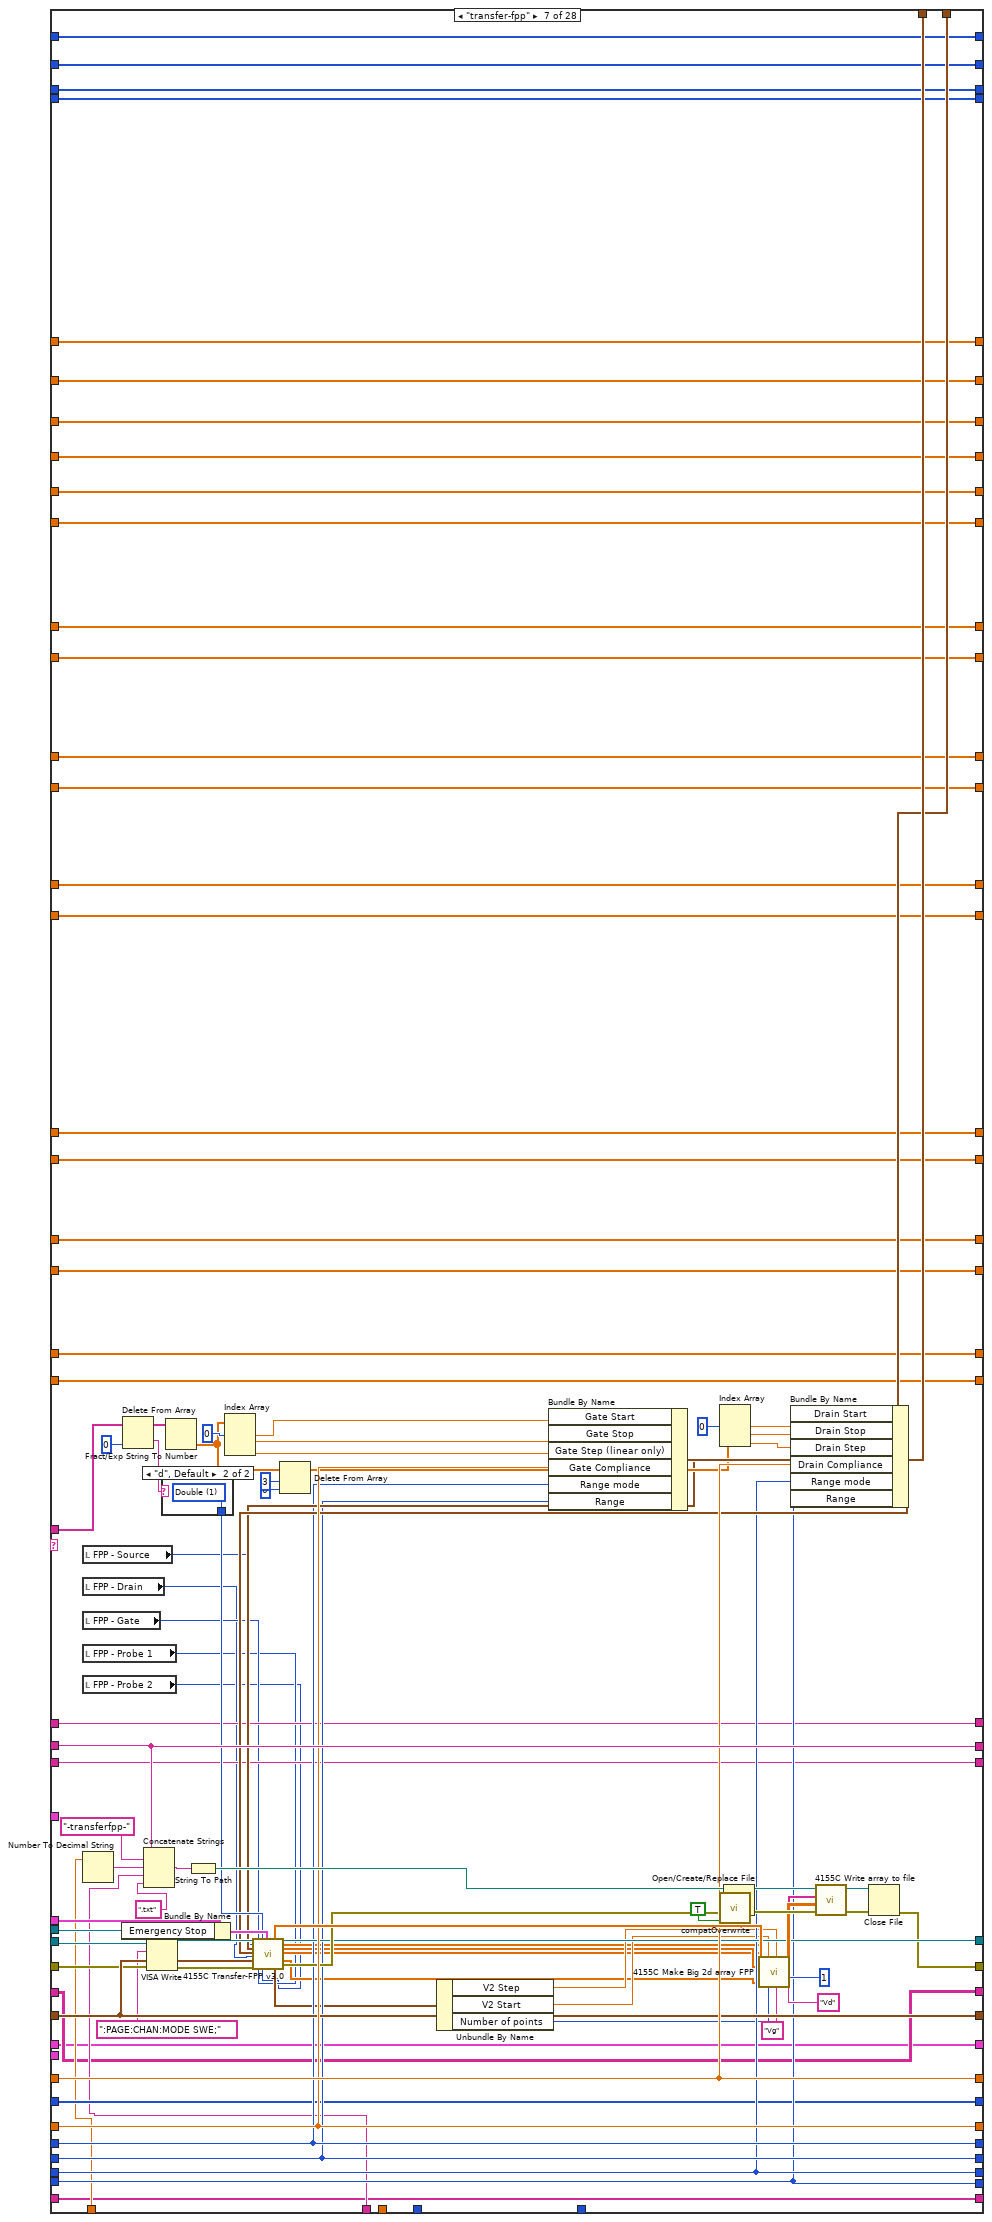
[diagram p17: hidden frame]
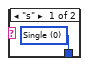
[diagram p18: hidden frame]
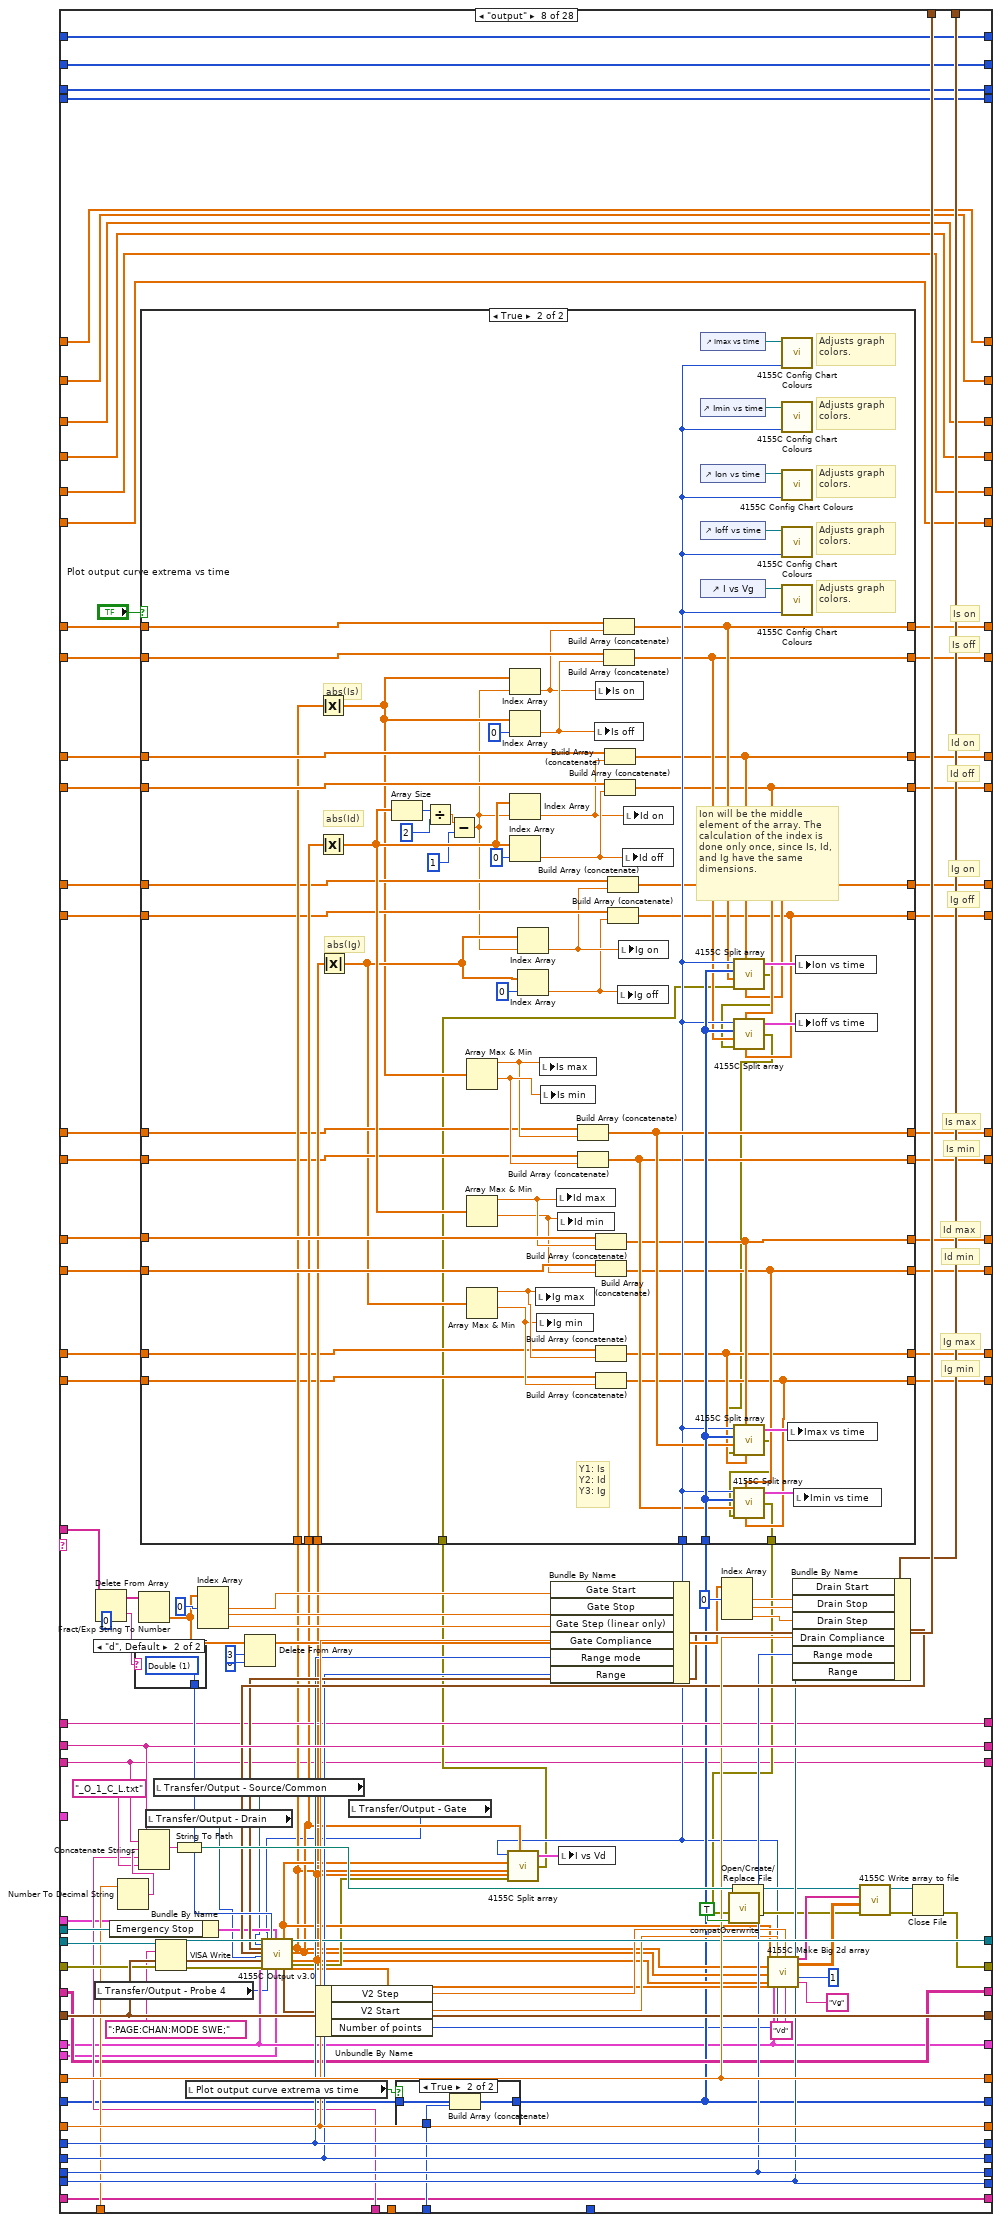
[diagram p19: hidden frame]
diagram:
  w3 = 0.0 ("Is off")
  w2 = cluster{"Y data in":dbl[], "X data in":dbl[]}[] [] ("I vs Vg")
  w12 = 0.0 ("Is off")
  w13 = 0.0 ("Is on")
  w14 = 0.0 ("Is min")
  w15 = 0.0 ("Is max")
  w61 = u16 1 items=["Reset All", "Partial reset"] ("Type of reset")
  # "Change from previous version:\n\n- Fixed sample-fpp and resample-fpp commands."
  # "This is a version specific to the SPM pump."
  # "I add 1 to both the \"total lines\" and the \"line running\" indicators because i and N begin from 0, and the script lines begin from 1."
  # "Bugs:\n\n- If using the \"filename\" command, keep in mind that the arrays of the time-dependent data are not re-initialized inbetween filename changes. \n\n- Do not connect the \"error\" wire of a Split block if it has unconnected terminals! It will halt the program."
  # "Array size"
  # "%s option converts a spreadsheet string to an array of strings."
  # "0: No of rows of array\n1: No of cols"
  # "Dimitrios Simatos\nv. 7.2"
  # "Changes from original textcontrol.vi:\n\n- Timestamp appears in filename.\n- (Only) transfer and output curves are plotted.\n- Communication with serial port.\n- Can execute any command, as all pattern matching functions were replaced. Previously, commands with special LabVIEW characters could not be executed.\n- Replaced write to file function with write to text file.\n- Replaced while loop with for loop.\n- Replaced 4155C \"Save File\" function and now the vi can save time-dependent variables.\n- Added clock with start time control and various units.\n- Changed filepath in which the program is saved.\n- Added a serial output log that keeps a history.\n- Tab control.\n- Addition of specialized serial read/write file for the SPM OEM pump.\n- Added halt and hard stop.\n- Added option for plotting transfer and output curve extrema vs time.\n- Corrected bug of \"itime\" command. The command did not allow for settting the integration time value, it allowed to set the category of the integration time (short, medium, long). If the time value was beyond the range of the category, then the SPA used the closest value allowed, whilst staying in the category. So, if the integration time was changed to long, but the integration time value was a short one, then the SPA would measure using the minimum long integration time value and not the value that the user intended.\n- Added Probe4 command.\n- Added plotting of \"sample\" plots.\n- Added SMU control.\n- Added universal SMU/VSU selector."
  # "Search and replace LF with EOL"
  n1 = Equal?(x="integration time", y=u32 0) -> (x = y?=w62:bool)
  n2 = Select(t="Integration time (short)", s=w62, f="Integration time (long)") -> (s? t:f=w16:dbl)
  n3 = call "4155C Get Filename.vi"("error in (no error)"=errorcluster {"status"=FALSE, "code"=0, "source"=""}) -> ("error out"=w56:errorcluster, "path"=w31:path)  [unwired: 2 in, 1 out]
  "Path" <- w31
  n4 = Bundle By Name(cluster="Timings (overwritten by the Front Panel)", "integration time"="integration time", "Short/Long integration time"=w16) -> (w54:T5)
  n5 = Path To String(path=w31) -> (string=w32:string)
  n6 = Search and Replace String(replace all?=TRUE ("replace all? (F)"), input string="Script", search string="\n", replace string="\r\n") -> (result string=w44:string)  [unwired: 4 in, 3 out]
  n7 = Match Pattern(string=w32, regular expression=".txt") -> (before substring=w28:string)  [unwired: 1 in, 3 out]
  n8 = call "4155C Initialise.vi"("VISA resource name in"="VISA resource name in", "Reset"="Full Reset", "Type of reset"=w61, "error in (no error)"=w56, "VISA Timeout Value"=u32 10000) -> ("VISA Resource Name out"=w55:refnum<visa-resource-name>, "error out"=w5:errorcluster)
  n9 = Concatenate Strings(w28, "Suffix (script)") -> (w27:string)
  n10 = Spreadsheet String To Array(delimiter (Tab)="\r\n", format string="%s", spreadsheet string="Script", array type (2D Dbl)="") -> (array=w35:string[][])
  n11 = String To Path(string=w27) -> (path=w8:path)
  n12 = Array Size(array=w35) -> (size(s)=w39:i32[])
  n13 = Initialize Array("") -> (w20:string[])  [unwired: 1 in]
  n14 = Open/Create/Replace File(file path (use dialog)=w8, error in=w5, operation (0:open)=T8."replace or create with confirmation") -> (refnum out=w7:refnum<file>, error out=w6:errorcluster)  [unwired: 3 in, 1 out]
  n15 = Initialize Array(0 ("element")) -> (w22:i32[])  [unwired: 1 in]
  n16 = Initialize Array("") -> (w18:string[][])  [unwired: 2 in]
  n17 = Initialize Array(0.0 ("element")) -> (w1:dbl[])  [unwired: 1 in]
  n18 = Index Array(array=w39, index=0) -> (element=w37:i32)
  n19 = Write to Text File(file (use dialog)=w7, text=w44, error in=w6) -> (error out=w26:errorcluster)  [unwired: 1 in, 2 out]
  n20 = for {
    N: w37 -> [w210]
    shift-left: "Source/Drain Range" -> [w250]
    shift-right: [w246] -> _
    shift-left: "Source/Drain\nRange mode" -> [w251]
    shift-right: [w247] -> _
    shift-left: "Gate Range" -> [w252]
    shift-right: [w248] -> _
    shift-left: "Gate Range\nmode" -> [w253]
    shift-right: [w249] -> _
    shift-left: "Gate: Compliance" -> [w261]
    shift-right: [w258] -> _
    shift-left: "Drain: Compliance" -> [w262]
    shift-right: [w259] -> _
    shift-left: w54 -> [w263]
    shift-right: [w72] -> _
    shift-left: w26 -> [w264]
    shift-right: [w71] -> _
    shift-left: w55 -> [w265]
    shift-right: [w260] -> _
    shift-left: w28 -> [w266]
    shift-right: [w81] -> _
    tunnel: "Panel Controls 2" -> [w244]
    shift-right: [w122] -> _
    shift-left: w1 -> [w243]
    shift-right: [w180] -> _
    shift-left: i32[] [] -> [w239]
    tunnel: w35 -> [w238] mode=indexing
    shift-right: [w121] -> _
    shift-left: w1 -> [w215]
    shift-right: [w153] -> _
    shift-left: w20 -> [w202]
    shift-right: [w181] -> _
    shift-left: w22 -> [w197]
    shift-right: [w163] -> _
    shift-left: w22 -> [w196]
    shift-right: [w195] -> _
    shift-left: "" -> [w194]
    shift-right: [w158] -> _
    shift-left: w22 -> [w178]
    shift-right: [w157] -> _
    shift-left: w22 -> [w162]
    shift-right: [w154] -> _
    shift-left: w18 -> [w156]
    shift-right: [w115] -> _
    shift-left: w1 -> [w143]
    shift-right: [w116] -> _
    shift-left: w1 -> [w142]
    shift-right: [w120] -> _
    shift-left: w1 -> [w131]
    shift-right: [w119] -> _
    shift-left: w1 -> [w130]
    shift-right: [w113] -> _
    shift-left: w1 -> [w129]
    shift-right: [w123] -> _
    shift-left: w1 -> [w128]
    shift-right: [w114] -> _
    shift-left: w1 -> [w127]
    shift-right: [w112] -> _
    shift-left: w1 -> [w126]
    shift-right: [w118] -> _
    shift-left: w1 -> [w125]
    shift-right: [w117] -> _
    shift-left: w1 -> [w124]
    shift-right: [w80] -> _
    shift-left: "Filename (variable part)" -> [w107]
    shift-right: [w73] -> _
    shift-left: "Probe 4" -> [w245]
    shift-right: [w76] -> _
    shift-left: w1 -> [w102]
    shift-right: [w77] -> _
    shift-left: w1 -> [w101]
    shift-right: [w78] -> _
    shift-left: w1 -> [w100]
    shift-right: [w79] -> _
    shift-left: w1 -> [w99]
    shift-right: [w67] -> _
    shift-left: w1 -> [w70]
    shift-right: [w68] -> _
    shift-left: w1 -> [w69]
    i -> [w205]
    stop <- "Interrupt program" stop-if-true
    # "Vp2 for FPP bias stress plots"
    # "Vp1 for FPP bias stress plots"
    # "Ig for bias stress plots"
    # "Id for bias stress plots"
    # "Is for bias stress plots"
    # "Time axis for bias stress plots"
    # "Save bias stress curves in file."
    # "Filename prefix"
    # "Is off"
    # "Is on"
    # "Ig off"
    # "Ig on"
    # "Is min"
    # "Is max"
    # "Ig min"
    # "Ig max"
    # "Id min"
    # "Id max"
    # "Id off"
    # "Id on"
    # "Pump status"
    # "Filepath and name"
    # "Pump status"
    # "Limit of command arguments (array columns). Raise if needed."
    # "Serial port data (string)"
    # "Serial port data (table)"
    # "Time array for valve position"
    # "Time array for absolute plunger position"
    # "Valve position"
    # "Absolute plunger position"
    # "Serial port data"
    # "For loop counter"
    # "<-----Equivalent to the 4155C \"Write\" subvi.----->"
    # "Headers"
    # "Save transfer curves in file."
    # "Filepath and name"
    # "Save time-dependent data."
    # "Use the time offset if your measurements do not start at t=0."
    # "Time for Imax, Imin, Ion, Ioff"
    # "Rest of elements of command"
    # "First element of command\n(case select)"
    n21 = Add(x=w205, y=1) -> (x+y=→"Line running":i32)
    n22 = Add(x=w210, y=1) -> (x+y=→"Total lines":i32)
    n23 = Index Array(array=w238, index=0 ("line index")) -> (element=w233:string)
    "Command running:" <- w233
    n24 = control-ref of="Interrupt scan"() -> (w257:refnum<vi>)
    n25 = Spreadsheet String To Array(delimiter (Tab)=" ", format string="%s", spreadsheet string=w233, array type (2D Dbl)=string[] []) -> (array=w231:string[])
    n26 = Delete From Array(array=w231, index=0) -> (deleted portion=w144:string, array with subset deleted=w230:string[])  [unwired: 1 in]
    n27 = call "Elapsed Time"("Reset"="Reset", "Auto Reset"="Auto Reset") -> ("Elapsed Time (s)"=w240:dbl)  [unwired: 10 in, 7 out]
    n28 = case shown="1" "Time Units" {
      tunnel: ["-sec" "-min" "-h"] -> w241
      tunnel: [w270 w274 w277] -> w211
      tunnel: w240 -> [w270 w273 w278]
      frame 0, Default {
      }
      frame 1 {
        n29 = Divide(x=w273, y=60.0) -> (x/y=w274:dbl)
      }
      frame 2 {
        n30 = Divide(x=w278, y=3600.0) -> (x/y=w277:dbl)
      }
    }
    n31 = Add(x=w211, y="Time Offset") -> (x+y=w103:dbl)
    n32 = To Long Integer(number=w103) -> (32bit integer=w104:i32)
    "Elapsed Time" <- w104
    n33 = case shown="\"sample-fpp\"" w144 {
      tunnel: w230 -> [w322 w367 w411 w421 w568 w688 w845 w976 w1149 w1183 w1270 w1323 w1374 w1421 w1461 _ _ w1678 w1817 _ w1937 w2009 w2078 w2203 w2359 w2449 w2526 w2587]
      tunnel: w266 -> [w317 w363 w409 w443 w575 w752 w853 w983 w1157 w1206 w1259 w1315 w1367 w1415 w1454 w1499 w1567 w1605 w1799 w1856 w1924 w1996 w2066 w2197 w2355 w2451 w2528 w2589]
      tunnel: w265 -> [w316 w362 w400 w441 w546 w737 w822 w954 w1125 w1207 w1260 w1316 w1368 w1416 w1455 w1504 w1569 w1683 w1823 w1860 w1943 w2015 w2084 w2209 w2319 w2455 w2532 w2591]
      tunnel: w264 -> [w315 w361 w399 w440 w545 w736 w821 w953 w1122 w1208 w1261 w1317 w1369 w1417 w1456 w1503 w1540 w1682 w1822 w1859 w1942 w2014 w2083 w2208 w2318 w2454 w2531 w2592]
      tunnel: w263 -> [w314 w360 w408 w438 w571 w713 w849 w979 w1153 w1216 w1269 w1314 w1366 w1414 w1453 w1502 w1564 w1653 w1791 w1865 w1917 w1989 w2059 w2196 w2354 w2456 w2533 w2594]
      tunnel: w262 -> [w313 w359 w407 w437 w573 w750 w851 w981 w1155 w1215 w1268 w1322 w1373 w1420 w1460 w1501 w1549 w1681 w1821 w1868 w1941 w2013 w2082 w2207 w2363 w2457 w2534 w2595]
      tunnel: w261 -> [w312 w358 w406 w435 w572 w749 w850 w980 w1154 w1214 w1267 w1321 w1372 w1419 w1459 w1500 w1550 w1661 w1800 w1867 w1925 w1997 w2067 w2198 w2356 w2459 w2535 w2597]
      tunnel: [w316 w362 w398 w441 w570 w747 w847 w978 w1151 w1207 w1260 w1316 w1368 w1416 w1455 w1504 w1569 w1654 w1773 w1858 w1918 w1990 w2060 w2156 w2321 w2455 w2532 w2591] -> w260
      tunnel: [w315 w361 w397 w440 w569 w746 w846 w977 w1150 w1208 w1261 w1317 w1369 w1417 w1456 w1503 w1539 w1662 w1774 w1857 w1926 w1998 w2068 w2155 w2320 w2453 w2530 w2592] -> w177
      tunnel: [w314 w360 w408 w438 w571 w709 w849 w979 w1153 w1209 w1262 w1314 w1366 w1414 w1453 w1502 w1564 w1653 w1791 w1865 w1917 w1989 w2059 w2196 w2354 w2456 w2533 w2594] -> w72
      tunnel: [w313 w359 w407 w437 w573 w750 w851 w981 w1155 w1215 w1268 w1322 w1373 w1420 w1460 w1501 w1549 w1681 w1821 w1868 w1941 w2013 w2082 w2207 w2363 w2457 w2534 w2595] -> w259
      tunnel: [w312 w358 w406 w435 w572 w749 w850 w980 w1154 w1214 w1267 w1321 w1372 w1419 w1459 w1500 w1550 w1661 w1800 w1867 w1925 w1997 w2067 w2198 w2356 w2459 w2535 w2597] -> w258
      tunnel: [w317 w363 w409 w443 w575 w752 w853 w983 w1157 w1206 w1259 w1315 w1367 w1415 w1454 w1499 w1567 w1605 w1799 w1856 w1924 w1996 w2066 w2197 w2355 w2451 w2528 w2589] -> w81
      tunnel: w257 -> [_ _ _ _ w577 w756 w858 w985 w1161 _ _ _ _ _ _ _ _ w1658 w1796 _ w1923 w1995 w2065 w2175 w2337 _ _ _]
      tunnel: "Gate" -> [_ _ _ _ w555 w740 w832 w963 w1136 _ _ _ _ _ _ _ _ _ _ _ _ _ _ _ _ _ _ _]
      tunnel: "Drain 2" -> [_ _ _ _ w554 w739 w831 w962 w1135 _ _ _ _ _ _ _ _ _ _ _ _ _ _ _ _ _ _ _]
      tunnel: "Panel Controls" -> [_ _ _ _ _ _ w830 w883 w1134 _ _ _ _ _ _ _ _ _ _ _ _ _ _ _ _ _ _ _]
      tunnel: w253 -> [w311 w357 w405 w434 w539 w730 w815 w947 w1120 w1213 w1266 _ w1365 w1413 w1452 w1498 w1551 w1649 w1787 w1861 w1913 w1985 w2055 w2192 w2350 w2460 w2536 w2598]
      tunnel: w252 -> [w310 w356 w404 w433 w538 w729 w814 w946 w1119 w1212 w1265 w1320 _ w1404 w1458 w1497 w1552 w1650 w1788 w1862 w1914 w1986 w2056 w2193 w2351 w2461 w2537 w2599]
      tunnel: w251 -> [w309 w355 w403 w432 w537 w728 w813 w945 w1118 w1211 w1264 w1319 w1371 w1418 _ w1496 w1553 w1651 w1789 w1863 w1915 w1987 w2057 w2194 w2352 w2462 w2538 w2600]
      tunnel: w250 -> [w308 w354 w402 w431 w536 w727 w812 w944 w1121 w1210 w1263 w1318 w1370 _ w1457 w1495 w1554 w1652 w1790 w1864 w1916 w1988 w2058 w2195 w2353 w2463 w2539 w2601]
      tunnel: [w311 w357 w405 w434 w539 w730 w815 w947 w1120 w1213 w1266 w1313 w1365 w1413 w1452 w1498 w1551 w1649 w1787 w1861 w1913 w1985 w2055 w2192 w2350 w2460 w2536 w2598] -> w249
      tunnel: [w310 w356 w404 w433 w538 w729 w814 w946 w1119 w1212 w1265 w1320 w1357 w1404 w1458 w1497 w1552 w1650 w1788 w1862 w1914 w1986 w2056 w2193 w2351 w2461 w2537 w2599] -> w248
      tunnel: [w309 w355 w403 w432 w537 w728 w813 w945 w1118 w1211 w1264 w1319 w1371 w1418 w1451 w1496 w1553 w1651 w1789 w1863 w1915 w1987 w2057 w2194 w2352 w2462 w2538 w2600] -> w247
      tunnel: [w308 w354 w402 w431 w536 w727 w812 w944 w1121 w1210 w1263 w1318 w1370 w1405 w1457 w1495 w1554 w1652 w1790 w1864 w1916 w1988 w2058 w2195 w2353 w2463 w2539 w2601] -> w246
      tunnel: w245 -> [w286 w329 w374 _ w472 w676 w778 w880 w1083 w1180 w1236 w1291 w1335 w1382 w1429 w1473 w1511 w1626 w1747 w1834 w1878 w1954 w2025 w2136 w2297 w2414 w2470 w2585]
      tunnel: w244 -> [_ _ _ _ w530 w724 _ _ _ _ _ _ _ _ _ _ _ _ _ _ _ _ _ _ _ _ _ _]
      tunnel: [w307 w350 w395 w448 w487 w701 w802 w896 w1107 w1205 w1257 w1312 w1356 w1403 w1450 w1494 w1535 w1615 w1752 w1855 w1902 w1978 w2049 w2110 w2277 w2452 w2529 w2606] -> w122
      tunnel: w243 -> [w307 w350 w395 w448 w527 w701 w802 w936 w1107 w1205 w1257 w1312 w1356 w1403 w1450 w1494 w1535 w1622 w1752 w1855 w1902 w1978 w2049 w2116 w2281 w2452 w2529 w2606]
      tunnel: w103 -> [_ _ _ _ w526 w698 w800 w935 w1104 _ _ _ _ _ _ _ w1533 w1642 w1769 _ w1899 w1975 w2046 w2152 w2312 _ _ _]
      tunnel: w241 -> [_ _ _ _ w523 w697 w798 w932 w1103 _ _ _ _ _ _ _ w1531 w1640 w1768 _ w1898 w1974 w2045 w2151 w2313 _ w2497 _]
      tunnel: w104 -> [_ _ _ _ w519 _ _ w928 _ _ _ _ _ _ _ _ _ _ _ _ _ _ _ _ _ _ w2500 _]
      tunnel: [w306 w349 w394 w436 w491 w700 w801 w900 w1106 w1204 w1256 w1311 w1355 w1402 w1449 w1493 w1534 w1607 w1771 w1854 w1901 w1977 w2048 w2104 w2271 w2458 w2509 w2596] -> w180
      tunnel: w239 -> [w306 w349 w394 w436 w522 w700 w801 w931 w1106 w1204 w1256 w1311 w1355 w1402 w1449 w1493 w1534 w1611 w1771 w1854 w1901 w1977 w2048 w2105 w2272 w2458 w2509 w2596]
      tunnel: [w305 w348 w393 w447 w486 w696 w797 w895 w1102 w1203 w1255 w1310 w1354 w1401 w1448 w1492 w1530 w1614 w1751 w1853 w1897 w1973 w2044 w2109 w2276 w2447 w2525 w2605] -> w121
      tunnel: w215 -> [w305 w348 w393 w447 w518 w696 w797 w927 w1102 w1203 w1255 w1310 w1354 w1401 w1448 w1492 w1530 w1621 w1751 w1853 w1897 w1973 w2044 w2115 w2280 w2447 w2525 w2605]
      tunnel: [w304 w347 w392 w430 w511 w695 w796 w920 w1101 w1202 w1254 w1309 w1353 w1400 w1447 w1491 w1529 w1639 w1767 w1852 w1896 w1972 w2043 w2150 w2311 w2446 w2524 w2602] -> w153
      tunnel: w202 -> [w304 w347 w392 w430 w511 w695 w796 w920 w1101 w1202 w1254 w1309 w1353 w1400 w1447 w1491 w1529 w1639 w1767 w1852 w1896 w1972 w2043 w2150 w2311 w2445 w2498 w2602]
      tunnel: [w303 w346 w391 w458 w510 w694 w795 w919 w1100 w1201 w1253 w1308 w1352 w1399 w1446 w1490 w1528 w1638 w1766 w1851 w1895 w1971 w2042 w2149 w2310 w2431 w2511 w2616] -> w181
      tunnel: w197 -> [w303 w346 w391 w458 w510 w694 w795 w919 w1100 w1201 w1253 w1308 w1352 w1399 w1446 w1490 w1528 w1638 w1766 w1851 w1895 w1971 w2042 w2149 w2310 w2431 w2510 w2616]
      tunnel: [w302 w345 w390 w460 w509 w693 w794 w918 w1099 w1200 w1252 w1307 w1351 w1398 w1445 w1489 w1527 w1637 w1765 w1850 w1894 w1970 w2041 w2148 w2309 w2430 w2493 w2618] -> w163
      tunnel: w196 -> [w302 w345 w390 w460 w509 w693 w794 w918 w1099 w1200 w1252 w1307 w1351 w1398 w1445 w1489 w1527 w1637 w1765 w1850 w1894 w1970 w2041 w2148 w2309 w2430 w2491 w2618]
      tunnel: [w301 w344 w389 w444 w508 w692 w793 w917 w1098 w1199 w1251 w1306 w1350 w1397 w1444 w1488 w1526 w1636 w1764 w1849 w1893 w1969 w2040 w2147 w2308 w2429 w2490 w2590] -> w195
      tunnel: w194 -> [w301 w344 w389 w444 w508 w692 w793 w917 w1098 w1199 w1251 w1306 w1350 w1397 w1444 w1488 w1526 w1636 w1764 w1849 w1893 w1969 w2040 w2147 w2308 w2429 w2501 w2590]
      tunnel: w104 -> [_ _ _ _ _ _ _ _ _ _ _ _ _ _ _ _ _ _ _ _ _ _ _ _ _ _ w2489 _]
      tunnel: w178 -> [w300 w343 w388 w459 w507 w691 w792 w916 w1097 w1198 w1250 w1305 w1349 w1396 w1443 w1487 w1525 w1635 w1763 w1848 w1892 w1968 w2039 w2146 w2307 w2428 w2488 w2617]
      tunnel: [w300 w343 w388 w459 w507 w691 w792 w916 w1097 w1198 w1250 w1305 w1349 w1396 w1443 w1487 w1525 w1635 w1763 w1848 w1892 w1968 w2039 w2146 w2307 w2428 w2487 w2617] -> w158
      tunnel: [w299 w342 w387 w457 w506 w690 w791 w915 w1096 w1197 w1249 w1304 w1348 w1395 w1442 w1486 w1524 w1634 w1762 w1847 w1891 w1967 w2038 w2145 w2306 w2427 w2486 w2615] -> w157
      tunnel: w162 -> [w299 w342 w387 w457 w506 w690 w791 w915 w1096 w1197 w1249 w1304 w1348 w1395 w1442 w1486 w1524 w1634 w1762 w1847 w1891 w1967 w2038 w2145 w2306 w2427 w2485 w2615]
      tunnel: [w298 w341 w386 w439 w505 w689 w790 w914 w1095 w1196 w1248 w1303 w1347 w1394 w1441 w1485 w1523 w1633 w1761 w1846 w1890 w1966 w2037 w2144 w2305 w2426 w2483 w2593] -> w154
      tunnel: w156 -> [w298 w341 w386 w439 w505 w689 w790 w914 w1095 w1196 w1248 w1303 w1347 w1394 w1441 w1485 w1523 w1633 w1761 w1846 w1890 w1966 w2037 w2144 w2305 w2426 w2482 w2593]
      tunnel: [w296 w339 w384 w453 w480 w686 w788 w889 w1093 w1194 w1247 w1302 w1345 w1392 w1439 w1483 w1521 w1632 w1760 w1845 w1889 w1965 w2035 w2143 w2304 w2425 w2481 w2611] -> w115
      tunnel: w143 -> [w296 w339 w384 w453 w504 w686 w788 w913 w1093 w1194 w1247 w1302 w1345 w1392 w1439 w1483 w1521 w1632 w1760 w1845 w1889 w1965 w2035 w2143 w2304 w2425 w2481 w2611]
      tunnel: [w297 w340 w385 w454 w481 w687 w789 w890 w1094 w1195 w1246 w1301 w1346 w1393 w1440 w1484 w1522 w1631 w1759 w1844 w1888 w1964 w2036 w2142 w2303 w2424 w2480 w2612] -> w116
      tunnel: w142 -> [w297 w340 w385 w454 w503 w687 w789 w912 w1094 w1195 w1246 w1301 w1346 w1393 w1440 w1484 w1522 w1631 w1759 w1844 w1888 w1964 w2036 w2142 w2303 w2424 w2480 w2612]
      tunnel: [w289 w332 w377 w446 w485 w683 w786 w894 w1091 w1187 w1244 w1299 w1343 w1390 w1437 w1481 w1514 w1613 w1750 w1843 w1881 w1957 w2028 w2108 w2275 w2417 w2479 w2604] -> w120
      tunnel: w131 -> [w289 w332 w377 w446 w499 w683 w786 w908 w1091 w1187 w1244 w1299 w1343 w1390 w1437 w1481 w1514 w1620 w1750 w1843 w1881 w1957 w2028 w2114 w2279 w2417 w2479 w2604]
      tunnel: [w288 w331 w376 w445 w484 w684 w787 w893 w1092 w1186 w1245 w1300 w1344 w1391 w1438 w1482 w1513 w1612 w1749 w1842 w1880 w1956 w2027 w2107 w2274 w2416 w2478 w2603] -> w119
      tunnel: w130 -> [w288 w331 w376 w445 w498 w684 w787 w907 w1092 w1186 w1245 w1300 w1344 w1391 w1438 w1482 w1513 w1619 w1749 w1842 w1880 w1956 w2027 w2113 w2278 w2416 w2478 w2603]
      tunnel: [w291 w334 w379 w450 w490 w682 w784 w899 w1089 w1192 w1242 w1297 w1341 w1388 w1435 w1479 w1516 w1617 w1754 w1837 w1883 w1959 w2030 w2112 w2284 w2421 w2476 w2608] -> w113
      tunnel: w129 -> [w291 w334 w379 w450 w497 w682 w784 w906 w1089 w1192 w1242 w1297 w1341 w1388 w1435 w1479 w1516 w1624 w1754 w1837 w1883 w1959 w2030 w2118 w2285 w2421 w2476 w2608]
      tunnel: [w290 w333 w378 w449 w488 w685 w785 w897 w1090 w1193 w1243 w1298 w1342 w1389 w1436 w1480 w1515 w1616 w1753 w1836 w1882 w1958 w2029 w2111 w2282 w2420 w2477 w2607] -> w123
      tunnel: w128 -> [w290 w333 w378 w449 w496 w685 w785 w905 w1090 w1193 w1243 w1298 w1342 w1389 w1436 w1480 w1515 w1623 w1753 w1836 w1882 w1958 w2029 w2117 w2283 w2420 w2477 w2607]
      tunnel: [w293 w336 w381 w452 w479 w681 w782 w888 w1087 w1190 w1240 w1295 w1339 w1386 w1433 w1477 w1518 w1628 w1756 w1839 w1885 w1961 w2032 w2139 w2300 w2423 w2474 w2610] -> w114
      tunnel: w127 -> [w293 w336 w381 w452 w495 w681 w782 w904 w1087 w1190 w1240 w1295 w1339 w1386 w1433 w1477 w1518 w1628 w1756 w1839 w1885 w1961 w2032 w2139 w2300 w2423 w2474 w2610]
      tunnel: [w292 w335 w380 w451 w478 w680 w783 w887 w1088 w1191 w1241 w1296 w1340 w1387 w1434 w1478 w1517 w1627 w1755 w1838 w1884 w1960 w2031 w2138 w2299 w2422 w2475 w2609] -> w112
      tunnel: w126 -> [w292 w335 w380 w451 w494 w680 w783 w903 w1088 w1191 w1241 w1296 w1340 w1387 w1434 w1478 w1517 w1627 w1755 w1838 w1884 w1960 w2031 w2138 w2299 w2422 w2475 w2609]
      tunnel: [w295 w338 w383 w456 w483 w679 w780 w892 w1085 w1188 w1238 w1293 w1337 w1384 w1431 w1475 w1520 w1630 w1758 w1841 w1887 w1963 w2034 w2141 w2302 w2419 w2472 w2614] -> w118
      tunnel: w125 -> [w295 w338 w383 w456 w493 w679 w780 w902 w1085 w1188 w1238 w1293 w1337 w1384 w1431 w1475 w1520 w1630 w1758 w1841 w1887 w1963 w2034 w2141 w2302 w2419 w2472 w2614]
      tunnel: [w294 w337 w382 w455 w482 w678 w781 w891 w1086 w1189 w1239 w1294 w1338 w1385 w1432 w1476 w1519 w1629 w1757 w1840 w1886 w1962 w2033 w2140 w2301 w2418 w2473 w2613] -> w117
      tunnel: w124 -> [w294 w337 w382 w455 w492 w678 w781 w901 w1086 w1189 w1239 w1294 w1338 w1385 w1432 w1476 w1519 w1629 w1757 w1840 w1886 w1962 w2033 w2140 w2301 w2418 w2473 w2613]
      tunnel: w107 -> [w287 w330 w375 w442 w475 w677 w779 w884 w1084 w1185 w1237 w1292 w1336 w1383 w1430 w1474 w1512 w1604 w1748 w1835 w1879 w1955 w2026 w2137 w2298 w2415 w2471 _]
      tunnel: [w287 w330 w375 w442 w475 w677 w779 w884 w1084 w1185 w1237 w1292 w1336 w1383 w1430 w1474 w1512 w1604 w1748 w1835 w1879 w1955 w2026 w2137 w2298 w2415 w2471 w2586] -> w80
      tunnel: [w286 w329 w374 w420 w472 w676 w778 w880 w1083 w1180 w1236 w1291 w1335 w1382 w1429 w1473 w1511 w1626 w1747 w1834 w1878 w1954 w2025 w2136 w2297 w2414 w2470 w2585] -> w73
      tunnel: w103 -> [_ _ _ _ _ _ _ _ _ _ _ _ _ _ _ _ _ w1574 _ _ _ _ _ w2120 w2288 _ _ _]
      tunnel: [w285 w328 w373 w419 w471 w675 w777 w879 w1082 w1179 w1235 w1290 w1334 w1381 w1428 w1472 w1510 w1588 w1746 w1833 w1877 w1953 w2024 w2126 w2293 w2413 w2469 w2584] -> w76
      tunnel: [w284 w327 w372 w418 w470 w674 w776 w878 w1081 w1178 w1234 w1289 w1333 w1380 w1427 w1471 w1509 w1587 w1745 w1832 w1876 w1952 w2023 w2125 w2292 w2412 w2468 w2583] -> w77
      tunnel: [w283 w326 w371 w417 w469 w673 w775 w877 w1080 w1177 w1233 w1288 w1332 w1379 w1426 w1470 w1508 w1589 w1744 w1831 w1875 w1951 w2022 w2098 w2265 w2411 w2467 w2582] -> w78
      tunnel: [w282 w325 w370 w416 w468 w672 w774 w876 w1079 w1176 w1232 w1287 w1331 w1378 w1425 w1469 w1507 w1586 w1743 w1830 w1874 w1950 w2021 w2095 w2262 w2410 w2466 w2581] -> w79
      tunnel: w102 -> [w285 w328 w373 w419 w471 w675 w777 w879 w1082 w1179 w1235 w1290 w1334 w1381 w1428 w1472 w1510 w1585 w1746 w1833 w1877 w1953 w2024 w2129 w2296 w2413 w2469 w2584]
      tunnel: w101 -> [w284 w327 w372 w418 w470 w674 w776 w878 w1081 w1178 w1234 w1289 w1333 w1380 w1427 w1471 w1509 w1584 w1745 w1832 w1876 w1952 w2023 w2128 w2295 w2412 w2468 w2583]
      tunnel: w100 -> [w283 w326 w371 w417 w469 w673 w775 w877 w1080 w1177 w1233 w1288 w1332 w1379 w1426 w1470 w1508 w1583 w1744 w1831 w1875 w1951 w2022 w2098 w2265 w2411 w2467 w2582]
      tunnel: w99 -> [w282 w325 w370 w416 w468 w672 w774 w876 w1079 w1176 w1232 w1287 w1331 w1378 w1425 w1469 w1507 w1582 w1743 w1830 w1874 w1950 w2021 w2127 w2294 w2410 w2466 w2581]
      tunnel: "Standby" -> [_ _ _ _ w467 w671 _ w875 _ _ _ _ _ _ _ _ _ w1580 w1742 _ _ _ _ w2135 _ _ _ _]
      tunnel: w70 -> [w281 w324 w369 w415 w461 w665 w768 w869 w1072 w1175 w1231 w1286 w1330 w1377 w1424 w1468 w1506 w1571 w1737 w1829 w1870 w1947 w2019 w2092 w2259 w2409 w2465 w2580]
      tunnel: [w281 w324 w369 w415 w461 w665 w768 w869 w1072 w1175 w1231 w1286 w1330 w1377 w1424 w1468 w1506 w1571 w1737 w1829 w1870 w1947 w2019 w2090 w2257 w2409 w2465 w2580] -> w67
      tunnel: w69 -> [w280 w323 w368 w414 w462 w664 w767 w870 w1073 w1174 w1230 w1285 w1329 w1376 w1423 w1467 w1505 w1570 w1736 w1828 w1869 w1946 w2018 w2091 w2258 w2408 w2464 w2579]
      tunnel: [w280 w323 w368 w414 w462 w664 w767 w870 w1073 w1174 w1230 w1285 w1329 w1376 w1423 w1467 w1505 w1570 w1736 w1828 w1869 w1946 w2018 w2089 w2256 w2408 w2464 w2579] -> w68
      frame "wait" {
        n34 = Index Array(array=w322, index=0 ("Index")) -> (element=w320:string)
        n35 = Decimal String To Number(string=w320, default (0L)=u32 0) -> (number=w319:u32)  [unwired: 1 in, 1 out]
        n36 = Wait (ms)(milliseconds to wait=w319) -> ()  [unwired: 1 out]
      }
      frame "wait-min" {
        n37 = Index Array(array=w367, index=0 ("Index")) -> (element=w365:string)
        n38 = Decimal String To Number(string=w365, default (0L)=u32 0) -> (number=w353:u32)  [unwired: 1 in, 1 out]
        n39 = Multiply(x=w353, y=u32 60000) -> (x*y=w352:u32)
        n40 = Wait (ms)(milliseconds to wait=w352) -> ()  [unwired: 1 out]
      }
      frame "standby" {
        n41 = Index Array(array=w411, index=0 ("Index")) -> (element=w401:string)
        n42 = case shown="\"off\", Default" w401 {
          tunnel: [":PAGE:SCON:STAN 0" ":PAGE:SCON:STAN 1"] -> w396
          frame "off", Default {
          }
          frame "on" {
          }
        }
        n43 = VISA Write(VISA resource name=w400, write buffer=w396, error in (no error)=w399) -> (VISA resource name out=w398:refnum<visa-resource-name>, error out=w397:errorcluster)  [unwired: 1 out]
      }
      frame "Probe4" {
        n44 = Delete From Array(array=w421, index=0) -> (deleted portion=w424:string, array with subset deleted=w427:string[])  [unwired: 1 in]
        n45 = Equal?(x=w424, y="ON") -> (x = y?=w422:bool)
        n46 = Delete From Array(array=w427, index=0) -> (deleted portion=w426:string)  [unwired: 1 in, 1 out]
        n47 = Fract/Exp String To Number(string=w426) -> (number=w423:dbl)  [unwired: 3 in, 1 out]
        n48 = Bundle(w422, w423) -> (w420:cluster{bool, dbl})  [unwired: 1 in]
      }
      frame "transfer" {
        # "Is off"
        # "Is on"
        # "Ig off"
        # "Ig on"
        # "Is min"
        # "Is max"
        # "Ig min"
        # "Ig max"
        # "Id min"
        # "Id max"
        # "Id off"
        # "Id on"
        n49 = Delete From Array(array=w568, index=0 ("Index")) -> (deleted portion=w566:string, array with subset deleted=w565:string[])  [unwired: 1 in]
        n50 = Bundle By Name(cluster=w530, "Emergency Stop"=w577) -> (w531:T2)
        n51 = local read "Transfer/Output - Source/Common"() -> (w466:u32)
        n52 = Number To Decimal String(number=w526) -> (decimal integer string=w525:string)  [unwired: 1 in]
        n53 = case shown="\"d\", Default" w566 {
          tunnel: [w662 w663] -> w564
          frame "s" {
            w662 = u16 0 items=["Single", "Double"] ("sweep mode")
          }
          frame "d", Default {
            w663 = u16 1 items=["Single", "Double"] ("sweep mode")
          }
        }
        n54 = Fract/Exp String To Number(string=w565) -> (number=w550:dbl[])  [unwired: 3 in, 1 out]
        n55 = Concatenate Strings(w575, w475, w525, w523, "_T_1_C_L.txt" ("Suffix (transfer)")) -> (w576:string)
        n56 = VISA Write(VISA resource name=w546, write buffer=":PAGE:CHAN:MODE SWE;" ("write buffer (\"\")"), error in (no error)=w545) -> (VISA resource name out=w543:refnum<visa-resource-name>, error out=w544:errorcluster)  [unwired: 1 out]
        n57 = local read "Plot transfer curve extrema vs time"() -> (w473:bool)
        n58 = local read "Transfer/Output - Gate"() -> (w464:u32)
        n59 = local read "Transfer/Output - Drain"() -> (w465:u32)
        n60 = String To Path(string=w576) -> (path=w574:path)
        n61 = local read "Transfer/Output - Probe 4"() -> (w463:u32)
        n62 = Index Array(array=w550, index #1=0 ("Index")) -> (element #1=w563:dbl, element #2=w562:dbl, element #3=w561:dbl)  [unwired: 2 in]
        n63 = Delete From Array(array=w550, length=3 ("Length"), index=0 ("Index")) -> (array with subset deleted=w548:dbl[])  [unwired: 1 out]
        n64 = case shown="True" w473 {
          tunnel: w522 -> [w579 w582]
          tunnel: w519 -> [_ w581]
          tunnel: [w579 w580] -> w491
          frame False {
          }
          frame True {
            n65 = Build Array (concatenate)(w582, w581) -> (w580:i32[])
          }
        }
        n66 = Bundle By Name(cluster=w555, "Gate Start"=w563, "Gate Stop"=w562, "Gate Step (linear only)"=w561, "Gate Compliance"=w572, "Range mode"=w539, "Range"=w538) -> (w540:T6)
        n67 = Index Array(array=w548, index #1=0 ("Index")) -> (element #1=w558:dbl, element #2=w557:dbl, element #3=w556:dbl)  [unwired: 2 in]
        n68 = call <vilib>:"compatOverwrite.vi"("overwrite (F)"=TRUE) -> ("overwrite?"=w529:T8)
        n69 = Bundle By Name(cluster=w554, "Drain Start"=w558, "Drain Stop"=w557, "Drain Step"=w556, "Drain Compliance"=w573, "Range mode"=w537, "Range"=w536) -> (w541:T7)
        n70 = call "4155C Transfer v3.0.vi"("VISA resource name in"=w543, "Source/Common"=w466, 2:"Gate"=w540, 3:"Drain"=w541, 4:"Drain"=w465, "Timings"=w571, "error in (no error)"=w544, 7:"Probe 4"=w472, 8:"Gate"=w464, 9:"Probe 4"=w463, "sweep mode"=w564, "Panel Controls"=w531, "Standby"=w467) -> ("VG"=w528:dbl[], "Outparams"=w535:T9, "VISA Resource Name out"=w570:refnum<visa-resource-name>, "IS"=w501:dbl[], "ID"=w502:dbl[], "IG"=w500:dbl[], "error out"=w520:errorcluster, "Probe 4"=w532:dbl[])  [unwired: 7 in]
        n71 = Unbundle By Name(w535) -> ("V2 Step"=w534:dbl, "V2 Start"=w533:dbl, "Number of points"=w489:i32)
        n72 = call "4155C Split array.vi"("Number of VAR2 steps"=w489, "Y2 data in"=w502, "X data in"=w528, "Y1 data in"=w501, "Y3 data in"=w500, "error in (no error)"=w520) -> ("Array of clusters"=w521:cluster{"Y data in":dbl[], "X data in":dbl[]}[], "error out"=w477:errorcluster)  [unwired: 1 in]
        n73 = case shown="True" "Plot transfer curve extrema vs time" {
          tunnel: w527 -> [w591 w661]
          tunnel: w518 -> [w592 w656]
          tunnel: w504 -> [w585 w652]
          tunnel: w503 -> [w586 w651]
          tunnel: w502 -> [_ w648]
          tunnel: w501 -> [_ w646]
          tunnel: w500 -> [_ w645]
          tunnel: w499 -> [w593 w641]
          tunnel: w498 -> [w594 w640]
          tunnel: w497 -> [w589 w637]
          tunnel: w496 -> [w590 w636]
          tunnel: w495 -> [w584 w633]
          tunnel: w494 -> [w583 w632]
          tunnel: w493 -> [w588 w629]
          tunnel: w492 -> [w587 w628]
          tunnel: w491 -> [_ w621]
          tunnel: [w589 w616] -> w490
          tunnel: w489 -> [_ w615]
          tunnel: [w590 w614] -> w488
          tunnel: [w591 w613] -> w487
          tunnel: [w592 w612] -> w486
          tunnel: [w593 w611] -> w485
          tunnel: [w594 w610] -> w484
          tunnel: [w588 w609] -> w483
          tunnel: [w587 w608] -> w482
          tunnel: [w586 w607] -> w481
          tunnel: [w585 w606] -> w480
          tunnel: [w584 w605] -> w479
          tunnel: [w583 w604] -> w478
          tunnel: w477 -> [w595 w603]
          tunnel: [w595 w599] -> w476
          frame False {
          }
          frame True {
            # "Adjusts graph colors."
            # "Adjusts graph colors."
            # "Ion will be the middle element of the array. The calculation of the index is done only once, since Is, Id, and Ig have the same dimensions."
            # "abs(Ig)"
            # "abs(Is)"
            # "Y1: Is\nY2: Id\nY3: Ig"
            # "abs(Id)"
            # "Adjusts graph colors."
            # "Adjusts graph colors."
            # "Adjusts graph colors."
            n74 = Absolute Value(x=w646) -> (abs(x)=w631:dbl[])
            n75 = Absolute Value(x=w648) -> (abs(x)=w647:dbl[])
            n76 = Absolute Value(x=w645) -> (abs(x)=w634:dbl[])
            n77 = Array Size(array=w647) -> (size(s)=w655:i32)
            n78 = Divide(x=w655, y=2) -> (x/y=w598:dbl)
            n79 = Subtract(x=w598, y=1) -> (x-y=w597:dbl)
            n80 = Array Max & Min(array=w631) -> (max value=w638:dbl, min value=w639:dbl)  [unwired: 2 out]
            n81 = Array Max & Min(array=w647) -> (max value=w660:dbl, min value=w644:dbl)  [unwired: 2 out]
            n82 = Array Max & Min(array=w634) -> (max value=w643:dbl, min value=w642:dbl)  [unwired: 2 out]
            n83 = Index Array(array=w631, index=w597) -> (element=w622:dbl)
            n84 = Index Array(array=w631, index=0) -> (element=w623:dbl)
            n85 = Index Array(array=w647, index=w597) -> (element=w624:dbl)
            n86 = Index Array(array=w647, index=0) -> (element=w625:dbl)
            n87 = Index Array(array=w634, index=w597) -> (element=w627:dbl)
            n88 = Index Array(array=w634, index=0) -> (element=w626:dbl)
            n89 = local write "Ig max"(w643) -> ()
            n90 = local write "Ig min"(w642) -> ()
            n91 = local write "Is max"(w638) -> ()
            n92 = local write "Is min"(w639) -> ()
            n93 = local write "Id max"(w660) -> ()
            n94 = local write "Id min"(w644) -> ()
            n95 = Build Array (concatenate)(w637, w638) -> (w616:dbl[])
            n96 = Build Array (concatenate)(w636, w639) -> (w614:dbl[])
            n97 = local write "Is off"(w623) -> ()
            n98 = local write "Is on"(w622) -> ()
            n99 = Build Array (concatenate)(w661, w660) -> (w613:dbl[])
            n100 = Build Array (concatenate)(w656, w644) -> (w612:dbl[])
            n101 = Build Array (concatenate)(w641, w643) -> (w611:dbl[])
            n102 = Build Array (concatenate)(w640, w642) -> (w610:dbl[])
            n103 = Build Array (concatenate)(w629, w622) -> (w609:dbl[])
            n104 = Build Array (concatenate)(w628, w623) -> (w608:dbl[])
            n105 = Build Array (concatenate)(w651, w624) -> (w607:dbl[])
            n106 = Build Array (concatenate)(w652, w625) -> (w606:dbl[])
            n107 = Build Array (concatenate)(w633, w627) -> (w605:dbl[])
            n108 = Build Array (concatenate)(w632, w626) -> (w604:dbl[])
            n109 = local write "Ig off"(w626) -> ()
            n110 = local write "Ig on"(w627) -> ()
            n111 = local write "Id off"(w625) -> ()
            n112 = local write "Id on"(w624) -> ()
            n113 = control-ref of="Imax vs time"() -> (w650:refnum<vi>)
            n114 = control-ref of="Imin vs time"() -> (w649:refnum<vi>)
            n115 = control-ref of="Ion vs time"() -> (w618:refnum<vi>)
            n116 = control-ref of="Ioff vs time"() -> (w617:refnum<vi>)
            n117 = control-ref of="I vs Vg"() -> (w659:refnum<vi>)
            n118 = call "4155C Split array.vi"("Number of VAR2 steps"=w615, "Y2 data in"=w607, "X data in"=w621, "Y1 data in"=w609, "Y3 data in"=w605, "error in (no error)"=w603) -> ("Array of clusters"=w619:cluster{"Y data in":dbl[], "X data in":dbl[]}[], "error out"=w602:errorcluster)  [unwired: 1 in]
            n119 = call "4155C Split array.vi"("Number of VAR2 steps"=w615, "Y2 data in"=w606, "X data in"=w621, "Y1 data in"=w608, "Y3 data in"=w604, "error in (no error)"=w602) -> ("Array of clusters"=w620:cluster{"Y data in":dbl[], "X data in":dbl[]}[], "error out"=w601:errorcluster)  [unwired: 1 in]
            n120 = call "4155C Split array.vi"("Number of VAR2 steps"=w615, "Y2 data in"=w613, "X data in"=w621, "Y1 data in"=w616, "Y3 data in"=w611, "error in (no error)"=w601) -> ("Array of clusters"=w658:cluster{"Y data in":dbl[], "X data in":dbl[]}[], "error out"=w600:errorcluster)  [unwired: 1 in]
            n121 = call "4155C Split array.vi"("Number of VAR2 steps"=w615, "Y2 data in"=w612, "X data in"=w621, "Y1 data in"=w614, "Y3 data in"=w610, "error in (no error)"=w600) -> ("Array of clusters"=w657:cluster{"Y data in":dbl[], "X data in":dbl[]}[], "error out"=w599:errorcluster)  [unwired: 1 in]
            n122 = call "4155C Config Chart Colours.vi"("Numeric"=w615, "XY Graph 2"=w650) -> ()  [unwired: 6 in]
            n123 = call "4155C Config Chart Colours.vi"("Numeric"=w615, "XY Graph 2"=w649) -> ()  [unwired: 6 in]
            n124 = call "4155C Config Chart Colours.vi"("Numeric"=w615, "XY Graph 2"=w618) -> ()  [unwired: 6 in]
            n125 = call "4155C Config Chart Colours.vi"("Numeric"=w615, "XY Graph 2"=w617) -> ()  [unwired: 6 in]
            n126 = call "4155C Config Chart Colours.vi"("Numeric"=w615, "XY Graph 2"=w659) -> ()  [unwired: 6 in]
            n127 = local write "Imax vs time"(w658) -> ()
            n128 = local write "Imin vs time"(w657) -> ()
            n129 = local write "Ion vs time"(w619) -> ()
            n130 = local write "Ioff vs time"(w620) -> ()
          }
        }
        n131 = local write "I vs Vg"(w521) -> ()
        n132 = Open/Create/Replace File(file path (use dialog)=w574, error in=w476, operation (0:open)=w529) -> (refnum out=w516:refnum<file>, error out=w514:errorcluster)  [unwired: 3 in, 1 out]
        n133 = call "4155C Make Big 2d array.vi"("1D Var1"=w528, "1d IS"=w501, "1d ID"=w502, "1d IG"=w500, "1d SMU4"=w532, "SMU4"=w472, "VAR2 START"=w533, "Number of VAR2 steps"=w489, "VAR2 STEP"=w534, "VAR1 Name"="Vg", "Decimal places in header"=i8 1, "VAR2 Name"="Vd") -> ("Header array"=w517:string[], "Data array"=w515:dbl[][])  [unwired: 14 in]
        n134 = call "4155C Write array to file.vi"("Byte Stream File Refnum"=w516, "Header"=w517, "Data Array"=w515, "error in (no error)"=w514) -> ("dup refnum"=w513:refnum<file>, "error out"=w512:errorcluster)  [unwired: 1 in]
        n135 = Close File(refnum=w513, error in=w512) -> (error out=w569:errorcluster)  [unwired: 1 out]
      }
      frame "pulsedstressV" {
        w707 = 0
        n136 = local read "Pulsed Stress V - Source/Common"() -> (w670:u32)
        n137 = local read "Pulsed Stress V - Probe 4"() -> (w667:u32)
        n138 = Number To Decimal String(number=w698) -> (decimal integer string=w753:string)  [unwired: 1 in]
        n139 = local read "Pulsed Stress V - Vextra"() -> (w666:u32)
        n140 = local read "Pulsed Stress V - Drain"() -> (w669:u32)
        n141 = local read "Pulsed Stress V - Gate"() -> (w668:u32)
        n142 = Delete From Array(array=w688, index=0 ("Index")) -> (deleted portion=w744:string, array with subset deleted=w743:string[])  [unwired: 1 in]
        n143 = Bundle By Name(cluster=w724, "Emergency Stop"=w756) -> (w725:T2)
        n144 = VISA Write(VISA resource name=w737, write buffer=":PAGE:CHAN:MODE SWE;" ("write buffer (\"\")"), error in (no error)=w736) -> (VISA resource name out=w734:refnum<visa-resource-name>, error out=w735:errorcluster)  [unwired: 1 out]
        n145 = Concatenate Strings(w752, "-pulsedstressV-" ("Substring"), w753, w697, ".txt" ("Substring")) -> (w755:string)
        n146 = case shown="\"d\", Default" w744 {
          tunnel: [w765 w766] -> w742
          frame "s" {
            w765 = u16 0 items=["Single", "Double"] ("sweep mode")
          }
          frame "d", Default {
            w766 = u16 1 items=["Single", "Double"] ("sweep mode")
          }
        }
        n147 = Fract/Exp String To Number(string=w743) -> (number=w738:dbl[])  [unwired: 3 in, 1 out]
        n148 = String To Path(string=w755) -> (path=w751:path)
        n149 = Index Array(array=w738, index #1=0 ("Index")) -> (element #1=w716:dbl, element #2=w715:dbl, element #3=w712:dbl, element #4=w711:dbl, element #5=w710:dbl, element #6=w714:dbl)  [unwired: 5 in]
        n150 = Bundle By Name(cluster=w713, "Pulse period"=w711, "Base voltage"=w712, "Pulse width"=w710) -> (w709:T5)
        n151 = Unbundle By Name(w709) -> ("Pulse period"=w717:dbl)
        n152 = Bundle By Name(cluster=w740, "Gate Start"=w715, "Gate Stop"=w716, "Gate Step (linear only)"=0, "Gate Compliance"=w749, "Range mode"=w730, "Range"=w729) -> (w731:T6)
        n153 = call <vilib>:"compatOverwrite.vi"("overwrite (F)"=TRUE) -> ("overwrite?"=w702:T8)
        n154 = Bundle By Name(cluster=w739, "Drain Start"=w714, "Drain Stop"=w707, "Drain Step"=w707, "Drain Compliance"=w750, "Range mode"=w728, "Range"=w727) -> (w732:T7)
        n155 = call "4155C PulsedStressV v3.0.vi"("VISA resource name in"=w734, "Gate"=w731, "Pulsed Stress V - Source/Common"=w670, "Drain"=w732, "Timings"=w709, "error in (no error)"=w735, "sweep mode"=w742, "Probe 4"=w676, "Pulsed Stress V - Drain"=w669, "Pulsed Stress V - Gate"=w668, "Panel Controls"=w725, "Standby"=w671, "Pulsed Stress V - Probe 4"=w667, "Pulsed Stress V - Vextra"=w666) -> ("Outparams"=w726:T9, "VISA Resource Name out"=w747:refnum<visa-resource-name>, "ID"=w705:dbl[], "IG"=w703:dbl[], "error out"=w748:errorcluster)  [unwired: 1 in]
        n156 = Unbundle By Name(w726) -> ("Number of points"=w704:i32)  [unwired: 2 out]
        n157 = for {
          N: w704 -> [_]
          tunnel: [w762] -> w706 mode=indexing
          tunnel: w717 -> [w764]
          i -> [w763]
          n158 = Multiply(x=w764, y=w763) -> (x*y=w762:dbl)
        }
        n159 = Insert Into Array(array=dbl[][] [] ("Input Array"), new element=w706) -> (w718:dbl[][])  [unwired: 2 in]
        n160 = Insert Into Array(array=w718, new element=w705) -> (w723:dbl[][])  [unwired: 2 in]
        n161 = Insert Into Array(array=w723, new element=w703) -> (w722:dbl[][])  [unwired: 2 in]
        n162 = Transpose 2D Array(2D array=w722) -> (transposed array=w721:dbl[][])
        n163 = Open/Create/Replace File(file path (use dialog)=w751, error in=w748, operation (0:open)=w702) -> (refnum out=w759:refnum<file>, error out=w760:errorcluster)  [unwired: 3 in, 1 out]
        n164 = call "4155C Write array to file.vi"("Byte Stream File Refnum"=w759, "Header"=string[] ["Time /s", "Id /A", "Ig /A"], "Data Array"=w721, "error in (no error)"=w760) -> ("dup refnum"=w757:refnum<file>, "error out"=w758:errorcluster)  [unwired: 1 in]
        n165 = Close File(refnum=w757, error in=w758) -> (error out=w746:errorcluster)  [unwired: 1 out]
      }
      frame "transfer-fpp" {
        n166 = local read "FPP - Source"() -> (w773:u32)
        n167 = local read "FPP - Drain"() -> (w771:u32)
        n168 = local read "FPP - Gate"() -> (w772:u32)
        n169 = local read "FPP - Probe 1"() -> (w770:u32)
        n170 = local read "FPP - Probe 2"() -> (w769:u32)
        n171 = Number To Decimal String(number=w800) -> (decimal integer string=w854:string)  [unwired: 1 in]
        n172 = Bundle By Name(cluster=w830, "Emergency Stop"=w858) -> (w866:T1)
        n173 = Delete From Array(array=w845, index=0 ("Index")) -> (deleted portion=w843:string, array with subset deleted=w842:string[])  [unwired: 1 in]
        n174 = Concatenate Strings(w853, "-transferfpp-" ("Substring"), w854, w798, ".txt" ("Substring")) -> (w856:string)
        n175 = VISA Write(VISA resource name=w822, write buffer=":PAGE:CHAN:MODE SWE;" ("write buffer (\"\")"), error in (no error)=w821) -> (VISA resource name out=w819:refnum<visa-resource-name>, error out=w820:errorcluster)  [unwired: 1 out]
        n176 = case shown="\"d\", Default" w843 {
          tunnel: [w867 w868] -> w841
          frame "s" {
            w867 = u16 0 items=["Single", "Double"] ("sweep mode")
          }
          frame "d", Default {
            w868 = u16 1 items=["Single", "Double"] ("sweep mode")
          }
        }
        n177 = Fract/Exp String To Number(string=w842) -> (number=w826:dbl[])  [unwired: 3 in, 1 out]
        n178 = String To Path(string=w856) -> (path=w852:path)
        n179 = Index Array(array=w826, index #1=0 ("Index")) -> (element #1=w840:dbl, element #2=w839:dbl, element #3=w838:dbl)  [unwired: 2 in]
        n180 = Delete From Array(array=w826, length=3 ("Length"), index=0 ("Index")) -> (array with subset deleted=w824:dbl[])  [unwired: 1 out]
        n181 = Bundle By Name(cluster=w832, "Gate Start"=w840, "Gate Stop"=w839, "Gate Step (linear only)"=w838, "Gate Compliance"=w850, "Range mode"=w815, "Range"=w814) -> (w816:T6)
        n182 = Index Array(array=w824, index #1=0 ("Index")) -> (element #1=w835:dbl, element #2=w834:dbl, element #3=w833:dbl)  [unwired: 2 in]
        n183 = call <vilib>:"compatOverwrite.vi"("overwrite (F)"=TRUE) -> ("overwrite?"=w803:T8)
        n184 = Bundle By Name(cluster=w831, "Drain Start"=w835, "Drain Stop"=w834, "Drain Step"=w833, "Drain Compliance"=w851, "Range mode"=w813, "Range"=w812) -> (w817:T7)
        n185 = call "4155C Transfer-FPP v3.0.vi"("VISA resource name in"=w819, "FPP - Source"=w773, "Gate"=w816, "Drain"=w817, "FPP - Drain"=w771, "Timings"=w849, "error in (no error)"=w820, "FPP - Gate"=w772, "FPP - Probe 1"=w770, "sweep mode"=w841, "FPP - Probe 2"=w769, "Panel Controls"=w866) -> ("VG"=w857:dbl[], "Outparams"=w811:T9, "VISA Resource Name out"=w847:refnum<visa-resource-name>, "Vprobe2"=w807:dbl[], "ID"=w806:dbl[], "IG"=w805:dbl[], "Vprobe1"=w804:dbl[], "error out"=w848:errorcluster)  [unwired: 8 in]
        n186 = Unbundle By Name(w811) -> ("V2 Step"=w810:dbl, "V2 Start"=w809:dbl, "Number of points"=w808:i32)
        n187 = Open/Create/Replace File(file path (use dialog)=w852, error in=w848, operation (0:open)=w803) -> (refnum out=w863:refnum<file>, error out=w864:errorcluster)  [unwired: 3 in, 1 out]
        n188 = call "4155C Make Big 2d array FPP.vi"("1D Var1"=w857, "1d ID"=w806, "1d Vp2"=w807, "1d IG"=w805, "1d Vp1"=w804, "VAR2 START"=w809, "Number of VAR2 steps"=w808, "VAR2 STEP"=w810, "VAR1 Name"="Vg", "Decimal places in header"=i8 1, "VAR2 Name"="Vd") -> ("Header array"=w859:string[], "Data array"=w860:dbl[][])  [unwired: 15 in]
        n189 = call "4155C Write array to file.vi"("Byte Stream File Refnum"=w863, "Header"=w859, "Data Array"=w860, "error in (no error)"=w864) -> ("dup refnum"=w861:refnum<file>, "error out"=w862:errorcluster)  [unwired: 1 in]
        n190 = Close File(refnum=w861, error in=w862) -> (error out=w846:errorcluster)  [unwired: 1 out]
      }
      frame "output" {
        # "Is off"
        # "Is on"
        # "Ig off"
        # "Ig on"
        # "Is min"
        # "Is max"
        # "Ig min"
        # "Ig max"
        # "Id min"
        # "Id max"
        # "Id off"
        # "Id on"
        n191 = local read "Transfer/Output - Probe 4"() -> (w871:u32)
        n192 = Delete From Array(array=w976, index=0 ("Index")) -> (deleted portion=w974:string, array with subset deleted=w973:string[])  [unwired: 1 in]
        n193 = Bundle By Name(cluster=w883, "Emergency Stop"=w985) -> (w939:T1)
        n194 = Number To Decimal String(number=w935) -> (decimal integer string=w934:string)  [unwired: 1 in]
        n195 = case shown="\"d\", Default" w974 {
          tunnel: [w1070 w1071] -> w972
          frame "s" {
            w1070 = u16 0 items=["Single", "Double"] ("sweep mode")
          }
          frame "d", Default {
            w1071 = u16 1 items=["Single", "Double"] ("sweep mode")
          }
        }
        n196 = Fract/Exp String To Number(string=w973) -> (number=w958:dbl[])  [unwired: 3 in, 1 out]
        n197 = Concatenate Strings(w983, w884, w934, w932, "_O_1_C_L.txt" ("Suffix (transfer)")) -> (w984:string)
        n198 = local read "Transfer/Output - Drain"() -> (w873:u32)
        n199 = local read "Transfer/Output - Source/Common"() -> (w874:u32)
        n200 = VISA Write(VISA resource name=w954, write buffer=":PAGE:CHAN:MODE SWE;" ("write buffer (\"\")"), error in (no error)=w953) -> (VISA resource name out=w951:refnum<visa-resource-name>, error out=w952:errorcluster)  [unwired: 1 out]
        n201 = String To Path(string=w984) -> (path=w982:path)
        n202 = local read "Plot output curve extrema vs time"() -> (w881:bool)
        n203 = Index Array(array=w958, index #1=0 ("Index")) -> (element #1=w971:dbl, element #2=w970:dbl, element #3=w969:dbl)  [unwired: 2 in]
        n204 = Delete From Array(array=w958, length=3 ("Length"), index=0 ("Index")) -> (array with subset deleted=w956:dbl[])  [unwired: 1 out]
        n205 = local read "Transfer/Output - Gate"() -> (w872:u32)
        n206 = case shown="True" w881 {
          tunnel: w931 -> [w987 w990]
          tunnel: w928 -> [_ w989]
          tunnel: [w987 w988] -> w900
          frame False {
          }
          frame True {
            n207 = Build Array (concatenate)(w990, w989) -> (w988:i32[])
          }
        }
        n208 = Bundle By Name(cluster=w963, "Gate Start"=w971, "Gate Stop"=w970, "Gate Step (linear only)"=w969, "Gate Compliance"=w980, "Range mode"=w947, "Range"=w946) -> (w948:T6)
        n209 = Index Array(array=w956, index #1=0 ("Index")) -> (element #1=w966:dbl, element #2=w965:dbl, element #3=w964:dbl)  [unwired: 2 in]
        n210 = call <vilib>:"compatOverwrite.vi"("overwrite (F)"=TRUE) -> ("overwrite?"=w938:T8)
        n211 = Bundle By Name(cluster=w962, "Drain Start"=w966, "Drain Stop"=w965, "Drain Step"=w964, "Drain Compliance"=w981, "Range mode"=w945, "Range"=w944) -> (w949:T7)
        n212 = call "4155C Output v3.0.vi"("VISA resource name in"=w951, "Source/Common"=w874, 2:"Gate"=w948, 3:"Drain"=w949, 4:"Drain"=w873, "Timings"=w979, "error in (no error)"=w952, 7:"Probe 4"=w880, 8:"Gate"=w872, 9:"Probe 4"=w871, "sweep mode"=w972, "Panel controls"=w939, "Standby"=w875) -> ("VD"=w937:dbl[], "Outparams"=w943:T9, "VISA Resource Name out"=w978:refnum<visa-resource-name>, "IS"=w910:dbl[], "ID"=w911:dbl[], "IG"=w909:dbl[], "error out"=w929:errorcluster, "Probe 4"=w940:dbl[])  [unwired: 7 in]
        n213 = Unbundle By Name(w943) -> ("V2 Step"=w942:dbl, "V2 Start"=w941:dbl, "Number of points"=w898:i32)
        n214 = call "4155C Split array.vi"("Number of VAR2 steps"=w898, "Y2 data in"=w911, "X data in"=w937, "Y1 data in"=w910, "Y3 data in"=w909, "error in (no error)"=w929) -> ("Array of clusters"=w930:cluster{"Y data in":dbl[], "X data in":dbl[]}[], "error out"=w886:errorcluster)  [unwired: 1 in]
        n215 = case shown="True" "Plot output curve extrema vs time" {
          tunnel: w936 -> [w994 w1069]
          tunnel: w927 -> [w993 w1064]
          tunnel: w913 -> [w999 w1060]
          tunnel: w912 -> [w1000 w1059]
          tunnel: w911 -> [_ w1056]
          tunnel: w910 -> [_ w1054]
          tunnel: w909 -> [_ w1053]
          tunnel: w908 -> [w992 w1049]
          tunnel: w907 -> [w991 w1048]
          tunnel: w906 -> [w996 w1045]
          tunnel: w905 -> [w995 w1044]
          tunnel: w904 -> [w998 w1041]
          tunnel: w903 -> [w997 w1040]
          tunnel: w902 -> [w1002 w1037]
          tunnel: w901 -> [w1001 w1036]
          tunnel: w900 -> [_ w1029]
          tunnel: [w996 w1024] -> w899
          tunnel: w898 -> [_ w1023]
          tunnel: [w995 w1022] -> w897
          tunnel: [w994 w1021] -> w896
          tunnel: [w993 w1020] -> w895
          tunnel: [w992 w1019] -> w894
          tunnel: [w991 w1018] -> w893
          tunnel: [w1002 w1017] -> w892
          tunnel: [w1001 w1016] -> w891
          tunnel: [w1000 w1015] -> w890
          tunnel: [w999 w1014] -> w889
          tunnel: [w998 w1013] -> w888
          tunnel: [w997 w1012] -> w887
          tunnel: w886 -> [w1003 w1011]
          tunnel: [w1003 w1007] -> w885
          frame False {
          }
          frame True {
            # "Adjusts graph colors."
            # "Adjusts graph colors."
            # "Ion will be the middle element of the array. The calculation of the index is done only once, since Is, Id, and Ig have the same dimensions."
            # "abs(Ig)"
            # "abs(Is)"
            # "Y1: Is\nY2: Id\nY3: Ig"
            # "abs(Id)"
            # "Adjusts graph colors."
            # "Adjusts graph colors."
            # "Adjusts graph colors."
            n216 = Absolute Value(x=w1054) -> (abs(x)=w1039:dbl[])
            n217 = Absolute Value(x=w1056) -> (abs(x)=w1055:dbl[])
            n218 = Absolute Value(x=w1053) -> (abs(x)=w1042:dbl[])
            n219 = Array Size(array=w1055) -> (size(s)=w1063:i32)
            n220 = Divide(x=w1063, y=2) -> (x/y=w1006:dbl)
            n221 = Subtract(x=w1006, y=1) -> (x-y=w1005:dbl)
            n222 = Array Max & Min(array=w1039) -> (max value=w1046:dbl, min value=w1047:dbl)  [unwired: 2 out]
            n223 = Array Max & Min(array=w1055) -> (max value=w1068:dbl, min value=w1052:dbl)  [unwired: 2 out]
            n224 = Array Max & Min(array=w1042) -> (max value=w1051:dbl, min value=w1050:dbl)  [unwired: 2 out]
            n225 = Index Array(array=w1039, index=w1005) -> (element=w1030:dbl)
            n226 = Index Array(array=w1039, index=0) -> (element=w1031:dbl)
            n227 = Index Array(array=w1055, index=w1005) -> (element=w1032:dbl)
            n228 = Index Array(array=w1055, index=0) -> (element=w1033:dbl)
            n229 = Index Array(array=w1042, index=w1005) -> (element=w1035:dbl)
            n230 = Index Array(array=w1042, index=0) -> (element=w1034:dbl)
            n231 = local write "Ig max"(w1051) -> ()
            n232 = local write "Ig min"(w1050) -> ()
            n233 = local write "Is max"(w1046) -> ()
            n234 = local write "Is min"(w1047) -> ()
            n235 = local write "Id max"(w1068) -> ()
            n236 = local write "Id min"(w1052) -> ()
            n237 = Build Array (concatenate)(w1045, w1046) -> (w1024:dbl[])
            n238 = Build Array (concatenate)(w1044, w1047) -> (w1022:dbl[])
            n239 = local write "Is off"(w1031) -> ()
            n240 = local write "Is on"(w1030) -> ()
            n241 = Build Array (concatenate)(w1069, w1068) -> (w1021:dbl[])
            n242 = Build Array (concatenate)(w1064, w1052) -> (w1020:dbl[])
            n243 = Build Array (concatenate)(w1049, w1051) -> (w1019:dbl[])
            n244 = Build Array (concatenate)(w1048, w1050) -> (w1018:dbl[])
            n245 = Build Array (concatenate)(w1037, w1030) -> (w1017:dbl[])
            n246 = Build Array (concatenate)(w1036, w1031) -> (w1016:dbl[])
            n247 = Build Array (concatenate)(w1059, w1032) -> (w1015:dbl[])
            n248 = Build Array (concatenate)(w1060, w1033) -> (w1014:dbl[])
            n249 = Build Array (concatenate)(w1041, w1035) -> (w1013:dbl[])
            n250 = Build Array (concatenate)(w1040, w1034) -> (w1012:dbl[])
            n251 = local write "Ig off"(w1034) -> ()
            n252 = local write "Ig on"(w1035) -> ()
            n253 = local write "Id off"(w1033) -> ()
            n254 = local write "Id on"(w1032) -> ()
            n255 = control-ref of="Imax vs time"() -> (w1058:refnum<vi>)
            n256 = control-ref of="Imin vs time"() -> (w1057:refnum<vi>)
            n257 = control-ref of="Ion vs time"() -> (w1026:refnum<vi>)
            n258 = control-ref of="Ioff vs time"() -> (w1025:refnum<vi>)
            n259 = control-ref of="I vs Vg"() -> (w1067:refnum<vi>)
            n260 = call "4155C Split array.vi"("Number of VAR2 steps"=w1023, "Y2 data in"=w1015, "X data in"=w1029, "Y1 data in"=w1017, "Y3 data in"=w1013, "error in (no error)"=w1011) -> ("Array of clusters"=w1027:cluster{"Y data in":dbl[], "X data in":dbl[]}[], "error out"=w1010:errorcluster)  [unwired: 1 in]
            n261 = call "4155C Split array.vi"("Number of VAR2 steps"=w1023, "Y2 data in"=w1014, "X data in"=w1029, "Y1 data in"=w1016, "Y3 data in"=w1012, "error in (no error)"=w1010) -> ("Array of clusters"=w1028:cluster{"Y data in":dbl[], "X data in":dbl[]}[], "error out"=w1009:errorcluster)  [unwired: 1 in]
            n262 = call "4155C Split array.vi"("Number of VAR2 steps"=w1023, "Y2 data in"=w1021, "X data in"=w1029, "Y1 data in"=w1024, "Y3 data in"=w1019, "error in (no error)"=w1009) -> ("Array of clusters"=w1066:cluster{"Y data in":dbl[], "X data in":dbl[]}[], "error out"=w1008:errorcluster)  [unwired: 1 in]
            n263 = call "4155C Split array.vi"("Number of VAR2 steps"=w1023, "Y2 data in"=w1020, "X data in"=w1029, "Y1 data in"=w1022, "Y3 data in"=w1018, "error in (no error)"=w1008) -> ("Array of clusters"=w1065:cluster{"Y data in":dbl[], "X data in":dbl[]}[], "error out"=w1007:errorcluster)  [unwired: 1 in]
            n264 = call "4155C Config Chart Colours.vi"("Numeric"=w1023, "XY Graph 2"=w1058) -> ()  [unwired: 6 in]
            n265 = call "4155C Config Chart Colours.vi"("Numeric"=w1023, "XY Graph 2"=w1057) -> ()  [unwired: 6 in]
            n266 = call "4155C Config Chart Colours.vi"("Numeric"=w1023, "XY Graph 2"=w1026) -> ()  [unwired: 6 in]
            n267 = call "4155C Config Chart Colours.vi"("Numeric"=w1023, "XY Graph 2"=w1025) -> ()  [unwired: 6 in]
            n268 = call "4155C Config Chart Colours.vi"("Numeric"=w1023, "XY Graph 2"=w1067) -> ()  [unwired: 6 in]
            n269 = local write "Imax vs time"(w1066) -> ()
            n270 = local write "Imin vs time"(w1065) -> ()
            n271 = local write "Ion vs time"(w1027) -> ()
            n272 = local write "Ioff vs time"(w1028) -> ()
          }
        }
        n273 = local write "I vs Vd"(w930) -> ()
        n274 = Open/Create/Replace File(file path (use dialog)=w982, error in=w885, operation (0:open)=w938) -> (refnum out=w925:refnum<file>, error out=w923:errorcluster)  [unwired: 3 in, 1 out]
        n275 = call "4155C Make Big 2d array.vi"("1D Var1"=w937, "1d IS"=w910, "1d ID"=w911, "1d IG"=w909, "1d SMU4"=w940, "SMU4"=w880, "VAR2 START"=w941, "Number of VAR2 steps"=w898, "VAR2 STEP"=w942, "VAR1 Name"="Vd", "Decimal places in header"=i8 1, "VAR2 Name"="Vg") -> ("Header array"=w926:string[], "Data array"=w924:dbl[][])  [unwired: 14 in]
        n276 = call "4155C Write array to file.vi"("Byte Stream File Refnum"=w925, "Header"=w926, "Data Array"=w924, "error in (no error)"=w923) -> ("dup refnum"=w922:refnum<file>, "error out"=w921:errorcluster)  [unwired: 1 in]
        n277 = Close File(refnum=w922, error in=w921) -> (error out=w977:errorcluster)  [unwired: 1 out]
      }
      frame "output-fpp" {
        n278 = local read "FPP - Source"() -> (w1078:u32)
        n279 = local read "FPP - Drain"() -> (w1077:u32)
        n280 = local read "FPP - Gate"() -> (w1076:u32)
        n281 = local read "FPP - Probe 1"() -> (w1075:u32)
        n282 = local read "FPP - Probe 2"() -> (w1074:u32)
        n283 = Number To Decimal String(number=w1104) -> (decimal integer string=w1158:string)  [unwired: 1 in]
        n284 = Bundle By Name(cluster=w1134, "Emergency Stop"=w1161) -> (w1171:T1)
        n285 = Delete From Array(array=w1149, index=0 ("Index")) -> (deleted portion=w1147:string, array with subset deleted=w1146:string[])  [unwired: 1 in]
        n286 = VISA Write(VISA resource name=w1125, write buffer=":PAGE:CHAN:MODE SWE;" ("write buffer (\"\")"), error in (no error)=w1122) -> (VISA resource name out=w1124:refnum<visa-resource-name>, error out=w1123:errorcluster)  [unwired: 1 out]
        n287 = Concatenate Strings(w1157, "-outputfpp-" ("Substring"), w1158, w1103, ".txt" ("Substring")) -> (w1160:string)
        n288 = case shown="\"d\", Default" w1147 {
          tunnel: [w1172 w1173] -> w1145
          frame "s" {
            w1172 = u16 0 items=["Single", "Double"] ("sweep mode")
          }
          frame "d", Default {
            w1173 = u16 1 items=["Single", "Double"] ("sweep mode")
          }
        }
        n289 = Fract/Exp String To Number(string=w1146) -> (number=w1128:dbl[])  [unwired: 3 in, 1 out]
        n290 = String To Path(string=w1160) -> (path=w1156:path)
        n291 = Index Array(array=w1128, index #1=0 ("Index")) -> (element #1=w1144:dbl, element #2=w1143:dbl, element #3=w1142:dbl)  [unwired: 2 in]
        n292 = Delete From Array(array=w1128, length=3 ("Length"), index=0 ("Index")) -> (array with subset deleted=w1127:dbl[])  [unwired: 1 out]
        n293 = Bundle By Name(cluster=w1136, "Gate Start"=w1144, "Gate Stop"=w1143, "Gate Step (linear only)"=w1142, "Gate Compliance"=w1154, "Range mode"=w1120, "Range"=w1119) -> (w1170:T6)
        n294 = Index Array(array=w1127, index #1=0 ("Index")) -> (element #1=w1139:dbl, element #2=w1138:dbl, element #3=w1137:dbl)  [unwired: 2 in]
        n295 = call <vilib>:"compatOverwrite.vi"("overwrite (F)"=TRUE) -> ("overwrite?"=w1108:T8)
        n296 = Bundle By Name(cluster=w1135, "Drain Start"=w1139, "Drain Stop"=w1138, "Drain Step"=w1137, "Drain Compliance"=w1155, "Range mode"=w1118, "Range"=w1121) -> (w1169:T7)
        n297 = call "4155C Output-FPP v3.0.vi"("VISA resource name in"=w1124, "FPP - Source"=w1078, "Gate"=w1170, "Drain"=w1169, "FPP - Drain"=w1077, "Timings"=w1153, "error in (no error)"=w1123, "FPP - Gate"=w1076, "FPP - Probe 1"=w1075, "sweep mode"=w1145, "FPP - Probe 2"=w1074, "Panel controls"=w1171) -> ("VD"=w1113:dbl[], "Outparams"=w1116:T9, "VISA Resource Name out"=w1151:refnum<visa-resource-name>, "Vprobe2"=w1112:dbl[], "ID"=w1111:dbl[], "IG"=w1110:dbl[], "Vprobe1"=w1109:dbl[], "error out"=w1152:errorcluster)  [unwired: 8 in]
        n298 = Unbundle By Name(w1116) -> ("V2 Step"=w1117:dbl, "V2 Start"=w1115:dbl, "Number of points"=w1114:i32)
        n299 = Open/Create/Replace File(file path (use dialog)=w1156, error in=w1152, operation (0:open)=w1108) -> (refnum out=w1166:refnum<file>, error out=w1167:errorcluster)  [unwired: 3 in, 1 out]
        n300 = call "4155C Make Big 2d array FPP.vi"("1D Var1"=w1113, "1d ID"=w1111, "1d Vp2"=w1112, "1d IG"=w1110, "1d Vp1"=w1109, "VAR2 START"=w1115, "Number of VAR2 steps"=w1114, "VAR2 STEP"=w1117, "VAR1 Name"="Vd", "Decimal places in header"=i8 1, "VAR2 Name"="Vg") -> ("Header array"=w1162:string[], "Data array"=w1163:dbl[][])  [unwired: 15 in]
        n301 = call "4155C Write array to file.vi"("Byte Stream File Refnum"=w1166, "Header"=w1162, "Data Array"=w1163, "error in (no error)"=w1167) -> ("dup refnum"=w1164:refnum<file>, "error out"=w1165:errorcluster)  [unwired: 1 in]
        n302 = Close File(refnum=w1164, error in=w1165) -> (error out=w1150:errorcluster)  [unwired: 1 out]
      }
      frame "itime" {
        n303 = Delete From Array(array=w1183, index=1) -> (deleted portion=w1182:string)  [unwired: 1 in, 1 out]
        n304 = Delete From Array(array=w1183, index=0 ("Index")) -> (deleted portion=w1217:string)  [unwired: 1 in, 1 out]
        n305 = Fract/Exp String To Number(string=w1182) -> (number=w1181:dbl)  [unwired: 3 in, 1 out]
        n306 = case shown="\"l\"" w1217 {
          tunnel: w1216 -> [w1222 w1224 w1228]
          tunnel: [w1221 w1223 w1227] -> w1209
          tunnel: w1181 -> [w1219 _ w1226]
          frame "s" {
            w1220 = u32 0 items=["short  ", "medium  ", "long  "] ("integration time 2")
            n307 = Bundle By Name(cluster=w1222, "integration time"=w1220, "Short/Long integration time"=w1219) -> (w1221:T5)
          }
          frame "m", Default {
            w1225 = u32 1 items=["short  ", "medium  ", "long  "] ("integration time 2")
            n308 = Bundle By Name(cluster=w1224, "integration time"=w1225) -> (w1223:T5)
          }
          frame "l" {
            w1229 = u32 2 items=["short  ", "medium  ", "long  "] ("integration time 2")
            n309 = Bundle By Name(cluster=w1228, "integration time"=w1229, "Short/Long integration time"=w1226) -> (w1227:T5)
          }
        }
      }
      frame "pulsed" {
        n310 = Delete From Array(array=w1270, index=0 ("Index")) -> (deleted portion=w1271:string, array with subset deleted=w1258:string[])  [unwired: 1 in]
        n311 = case shown="\"on\", Default" w1271 {
          tunnel: w1269 -> [w1281 w1284]
          tunnel: [w1280 w1283] -> w1262
          tunnel: w1258 -> [w1278 _]
          frame "on", Default {
            w1279 = u16 1 items=["Continuous", "Pulsed"] ("sweep method")
            n312 = Fract/Exp String To Number(string=w1278) -> (number=w1276:dbl[])  [unwired: 3 in, 1 out]
            n313 = Index Array(array=w1276, index #1=0 ("Index")) -> (element #1=w1275:dbl, element #2=w1274:dbl, element #3=w1273:dbl)  [unwired: 2 in]
            n314 = Bundle By Name(cluster=w1281, "sweep method"=w1279, "Pulse period"=w1275, "Base voltage"=w1274, "Pulse width"=w1273) -> (w1280:T5)
          }
          frame "off" {
            w1282 = u16 0 items=["Continuous", "Pulsed"] ("sweep method")
            n315 = Bundle By Name(cluster=w1284, "sweep method"=w1282) -> (w1283:T5)
          }
        }
      }
      frame "gaterangemode" {
        n316 = Delete From Array(array=w1323, index=0 ("Index")) -> (deleted portion=w1324:string)  [unwired: 1 in, 1 out]
        n317 = case shown="\"f\"" w1324 {
          tunnel: [w1326 w1327 w1328] -> w1313
          frame "a", Default {
            w1326 = u16 0 items=["Auto", "Limited", "Fixed"] ("Gate Range\nmode 2")
          }
          frame "f" {
            w1327 = u16 2 items=["Auto", "Limited", "Fixed"] ("Gate Range\nmode 2")
          }
          frame "l" {
            w1328 = u16 1 items=["Auto", "Limited", "Fixed"] ("Gate Range\nmode 2")
          }
        }
      }
      frame "gaterange" {
        (unwired) u8 11 items=["10fA  ", "100fA  ", "1nA  ", "10nA", "100nA", "1uA", "10uA", "100uA", "1mA", "10mA", "100mA", "1A"] ("Gate Range 2")
        n318 = Delete From Array(array=w1374, index=0 ("Index")) -> (deleted portion=w1364:string)  [unwired: 1 in, 1 out]
        n319 = Scan Value(string=w1364, format string="") -> (value=w1362:dbl)  [unwired: 1 in, 1 out]
        n320 = Logarithm Base 10(1:w1362) -> (0:w1361:dbl)
        n321 = Round To Nearest(number=w1361) -> (nearest integer value=w1360:dbl)
        n322 = Add(x=w1360, y=11.0) -> (x+y=w1358:dbl)
        n323 = To Unsigned Byte Integer(number=w1358) -> (unsigned 8bit integer=w1357:u8)
      }
      frame "drainrange" {
        (unwired) u8 11 items=["10fA  ", "100fA  ", "1nA  ", "10nA", "100nA", "1uA", "10uA", "100uA", "1mA", "10mA", "100mA", "1A"] ("Gate Range 2")
        n324 = Delete From Array(array=w1421, index=0 ("Index")) -> (deleted portion=w1412:string)  [unwired: 1 in, 1 out]
        n325 = Scan Value(string=w1412, format string="") -> (value=w1410:dbl)  [unwired: 1 in, 1 out]
        n326 = Logarithm Base 10(1:w1410) -> (0:w1409:dbl)
        n327 = Round To Nearest(number=w1409) -> (nearest integer value=w1408:dbl)
        n328 = Add(x=w1408, y=11.0) -> (x+y=w1406:dbl)
        n329 = To Unsigned Byte Integer(number=w1406) -> (unsigned 8bit integer=w1405:u8)
      }
      frame "drainrangemode" {
        n330 = Delete From Array(array=w1461, index=0 ("Index")) -> (deleted portion=w1462:string)  [unwired: 1 in, 1 out]
        n331 = case shown="\"f\"" w1462 {
          tunnel: [w1464 w1465 w1466] -> w1451
          frame "a", Default {
            w1464 = u16 0 items=["Auto", "Limited", "Fixed"] ("Gate Range\nmode 2")
          }
          frame "f" {
            w1465 = u16 2 items=["Auto", "Limited", "Fixed"] ("Gate Range\nmode 2")
          }
          frame "l" {
            w1466 = u16 1 items=["Auto", "Limited", "Fixed"] ("Gate Range\nmode 2")
          }
        }
      }
      frame "Error", Default {
      }
      frame "logfile" {
        n332 = Number To Decimal String(number=w1533) -> (decimal integer string=w1568:string)  [unwired: 1 in]
        n333 = Concatenate Strings(w1567, "logfile" ("Substring"), w1568, w1531, ".txt" ("Substring")) -> (w1565:string)
        n334 = String To Path(string=w1565) -> (path=w1538:path)
        n335 = Unbundle(w1564) -> ("integration time"=w1563:u32, "Short/Long integration time"=w1562:dbl, "hold time (sec)"=w1561:dbl, "delay time (sec)"=w1560:dbl, "Step Time (0 disables)"=w1559:dbl, "sweep method"=w1558:u16, "Pulse period"=w1557:dbl, "Base voltage"=w1556:dbl, "Pulse width"=w1555:dbl)
        n336 = Build Array(w1563, w1562, w1561, w1560, w1559, w1558, w1557, w1556, w1555, w1549, w1550, w1551, w1552, w1553, w1554) -> (w1542:dbl[])
        n337 = Insert Into Array(array=dbl[][] [] ("Input Array"), new element=w1542) -> (w1541:dbl[][])  [unwired: 2 in]
        n338 = call <vilib>:"compatOverwrite.vi"("overwrite (F)"=TRUE) -> ("overwrite?"=w1536:T8)
        n339 = Open/Create/Replace File(file path (use dialog)=w1538, error in=w1540, operation (0:open)=w1536) -> (refnum out=w1546:refnum<file>, error out=w1545:errorcluster)  [unwired: 3 in, 1 out]
        n340 = call "4155C Write array to file.vi"("Byte Stream File Refnum"=w1546, "Header"=string[] ["Int Time", "Short/Long Itime", "Hold time", "Delay time", "Step time", "Sweep method", "Pulse period", "Base Voltage", "Pulse width", "Drain compliance", "Gate compliance", "Gate range mode", "Gate range", "S/D range mode", "S/D range"], "Data Array"=w1541, "error in (no error)"=w1545) -> ("dup refnum"=w1548:refnum<file>, "error out"=w1547:errorcluster)  [unwired: 1 in]
        n341 = Close File(refnum=w1548, error in=w1547) -> (error out=w1539:errorcluster)  [unwired: 1 out]
      }
      frame "sample" {
        w1608 = 1
        # "The suffix is Vg_Vd_Time."
        # "Add a time offset (elapsed time) to the time axis."
        # "Adjusts graph colors."
        n342 = Number To Decimal String(number=w1642) -> (decimal integer string=w1680:string)  [unwired: 1 in]
        n343 = local read "Sample - Drain"() -> (w1576:u32)
        n344 = Fract/Exp String To Number(string=w1678) -> (number=w1646:dbl[])  [unwired: 3 in, 1 out]
        n345 = Index Array(array=w1646, index=0 ("Index")) -> (element=w1600:dbl)
        n346 = Index Array(array=w1646, index=2 ("Index")) -> (element=w1674:dbl)
        n347 = Index Array(array=w1646, index=3 ("Index")) -> (element=w1597:dbl)
        n348 = Index Array(array=w1646, index=4 ("Index")) -> (element=w1645:dbl)
        n349 = Index Array(array=w1646, index=1 ("Index")) -> (element=w1602:dbl)
        n350 = local read "Sample - Probe 4"() -> (w1579:u32)
        n351 = local read "Sample - Source/Common"() -> (w1577:u32)
        n352 = local read "Time Units"() -> (w1572:u16)
        n353 = local read "Sample - Gate"() -> (w1578:u32)
        n354 = call "4155C Config Sampling Measurements v3.0.vi"("VISA session"=w1683, "Num Points"=w1674, "Sample - Drain"=w1576, "Display on/off"=TRUE, "Gate Compliance"=w1661, "Sampling interval"=w1645, "Sample - Source/Common"=w1577, "Sample - Probe 4"=w1579, "Drain Compliance"=w1681, "Standby"=w1580, "error in (no error)"=w1682, "Timings"=w1653, "Sample - Gate"=w1578, "Sample time"=w1597) -> ("dup VISA resource name"=w1685:refnum<visa-resource-name>, "error out"=w1684:errorcluster)
        n355 = local read "Plot sample extrema vs time"() -> (w1610:bool)
        n356 = Number To Decimal String(number=w1602) -> (decimal integer string=w1603:string)  [unwired: 1 in]
        n357 = Number To Decimal String(number=w1600) -> (decimal integer string=w1599:string)  [unwired: 1 in]
        n358 = Number To Decimal String(number=w1597) -> (decimal integer string=w1596:string)  [unwired: 1 in]
        n359 = call "4155C Take Sample v3.0.vi"("VISA resource name in"=w1685, "Emergency Stop"=w1658, "Sample - Gate"=w1578, "Vg"=w1600, "Sample - Drain"=w1576, "Vd"=w1602, "error in (no error)"=w1684) -> ("Time"=w1573:dbl[], "VISA Resource Name out"=w1655:refnum<visa-resource-name>, "Ig"=w1590:dbl[], "Id"=w1591:dbl[], "Is"=w1592:dbl[], "error out"=w1618:errorcluster)  [unwired: 3 in]
        n360 = Insert Into Array(array=w1584, new element=w1591) -> (w1587:dbl[])  [unwired: 1 in]
        n361 = case shown="0, Default" w1572 {
          tunnel: [w1688 w1689 w1692] -> w1575
          tunnel: w1573 -> [w1687 w1689 w1691]
          frame 2 {
            n362 = Divide(x=w1687, y=3600.0) -> (x/y=w1688:dbl[])
          }
          frame 0, Default {
          }
          frame 1 {
            n363 = Divide(x=w1691, y=60.0) -> (x/y=w1692:dbl[])
          }
        }
        n364 = Insert Into Array(array=w1583, new element=w1592) -> (w1589:dbl[])  [unwired: 1 in]
        n365 = Insert Into Array(array=w1585, new element=w1590) -> (w1588:dbl[])  [unwired: 1 in]
        n366 = Concatenate Strings(w1603, "_" ("Substring"), w1599, "_" ("Substring"), w1596, ".txt" ("Substring")) -> (w1594:string)
        n367 = Concatenate Strings(w1605, w1604, w1680, w1640, "_S_" ("Substring"), w1594) -> (w1679:string)
        n368 = String To Path(string=w1679) -> (path=w1664:path)
        n369 = Add(x=w1575, y=w1574) -> (x+y=w1593:dbl[])
        n370 = Insert Into Array(array=w1582, new element=w1593) -> (w1586:dbl[])  [unwired: 1 in]
        n371 = case shown="True" w1610 {
          tunnel: w1593 -> [_ w1695]
          tunnel: [w1693 w1696] -> w1607
          tunnel: w1611 -> [w1693 w1694]
          frame False {
          }
          frame True {
            n372 = Insert Into Array(array=w1694, new element=w1695) -> (w1696:i32[])  [unwired: 1 in]
          }
        }
        n373 = case shown="True" "Plot sample extrema vs time" {
          tunnel: w1592 -> [_ w1725]
          tunnel: w1591 -> [_ w1726]
          tunnel: w1590 -> [_ w1727]
          tunnel: [w1703 w1713] -> w1581
          tunnel: w1618 -> [w1703 w1718]
          tunnel: w1624 -> [w1702 w1730]
          tunnel: w1623 -> [w1701 w1729]
          tunnel: w1622 -> [w1700 w1731]
          tunnel: w1621 -> [w1699 w1728]
          tunnel: w1620 -> [w1698 w1733]
          tunnel: w1619 -> [w1697 w1732]
          tunnel: [w1702 w1717] -> w1617
          tunnel: [w1701 w1711] -> w1616
          tunnel: [w1700 w1715] -> w1615
          tunnel: [w1699 w1710] -> w1614
          tunnel: [w1698 w1716] -> w1613
          tunnel: [w1697 w1709] -> w1612
          tunnel: w1607 -> [_ w1707]
          frame False {
          }
          frame True {
            w1712 = 1
            # "Number of VAR2 steps is 1."
            # "abs(Ig)"
            # "abs(Is)"
            # "abs(Id)"
            # "Adjusts graph colors."
            n374 = Absolute Value(x=w1727) -> (abs(x)=w1704:dbl[])
            n375 = Absolute Value(x=w1726) -> (abs(x)=w1705:dbl[])
            n376 = Absolute Value(x=w1725) -> (abs(x)=w1706:dbl[])
            n377 = Array Max & Min(array=w1706) -> (max value=w1724:dbl, min value=w1721:dbl)  [unwired: 2 out]
            n378 = Array Max & Min(array=w1705) -> (max value=w1723:dbl, min value=w1720:dbl)  [unwired: 2 out]
            n379 = Array Max & Min(array=w1704) -> (max value=w1722:dbl, min value=w1719:dbl)  [unwired: 2 out]
            n380 = local write "Id max"(w1723) -> ()
            n381 = local write "Id min"(w1720) -> ()
            n382 = local write "Ig max"(w1722) -> ()
            n383 = local write "Ig min"(w1719) -> ()
            n384 = Insert Into Array(array=w1733, new element=w1704) -> (w1716:dbl[])  [unwired: 1 in]
            n385 = Insert Into Array(array=w1732, new element=w1704) -> (w1709:dbl[])  [unwired: 1 in]
            n386 = local write "Is max"(w1724) -> ()
            n387 = local write "Is min"(w1721) -> ()
            n388 = Insert Into Array(array=w1731, new element=w1705) -> (w1715:dbl[])  [unwired: 1 in]
            n389 = Insert Into Array(array=w1728, new element=w1705) -> (w1710:dbl[])  [unwired: 1 in]
            n390 = Insert Into Array(array=w1730, new element=w1706) -> (w1717:dbl[])  [unwired: 1 in]
            n391 = Insert Into Array(array=w1729, new element=w1706) -> (w1711:dbl[])  [unwired: 1 in]
            n392 = control-ref of="Imax vs time"() -> (w1734:refnum<vi>)
            n393 = call "4155C Config Chart Colours.vi"("Numeric"=w1712, "XY Graph 2"=w1734) -> ()  [unwired: 6 in]
            n394 = call "4155C Split array.vi"("Number of VAR2 steps"=w1712, "Y2 data in"=w1715, "X data in"=w1707, "Y1 data in"=w1717, "Y3 data in"=w1716, "error in (no error)"=w1718) -> ("Array of clusters"=w1735:cluster{"Y data in":dbl[], "X data in":dbl[]}[], "error out"=w1714:errorcluster)  [unwired: 1 in]
            n395 = call "4155C Split array.vi"("Number of VAR2 steps"=w1712, "Y2 data in"=w1710, "X data in"=w1707, "Y1 data in"=w1711, "Y3 data in"=w1709, "error in (no error)"=w1714) -> ("Array of clusters"=w1708:cluster{"Y data in":dbl[], "X data in":dbl[]}[], "error out"=w1713:errorcluster)  [unwired: 1 in]
            n396 = local write "Imax vs time"(w1735) -> ()
            n397 = local write "Imin vs time"(w1708) -> ()
          }
        }
        n398 = control-ref of="I vs time (Bias Stress)"() -> (w1606:refnum<vi>)
        n399 = call "4155C Split array.vi"("Number of VAR2 steps"=w1608, "Y2 data in"=w1587, "X data in"=w1586, "Y1 data in"=w1589, "Y3 data in"=w1588) -> ("Array of clusters"=w1609:cluster{"Y data in":dbl[], "X data in":dbl[]}[])  [unwired: 2 in, 1 out]
        n400 = local write "I vs time (Bias Stress)"(w1609) -> ()
        n401 = call "4155C Config Chart Colours.vi"("Numeric"=w1608, "XY Graph 2"=w1606) -> ()  [unwired: 6 in]
        n402 = Insert Into Array(array=dbl[][] [] ("Input Array"), new element=w1593) -> (w1668:dbl[][])  [unwired: 2 in]
        n403 = Insert Into Array(array=w1668, new element=w1590) -> (w1667:dbl[][])  [unwired: 2 in]
        n404 = VISA Write(VISA resource name=w1655, write buffer=":DISP ON" ("write buffer (\"\")"), error in (no error)=w1581) -> (VISA resource name out=w1654:refnum<visa-resource-name>, error out=w1656:errorcluster)  [unwired: 1 out]
        n405 = Insert Into Array(array=w1667, new element=w1591) -> (w1666:dbl[][])  [unwired: 2 in]
        n406 = Insert Into Array(array=w1666, new element=w1592) -> (w1660:dbl[][])  [unwired: 2 in]
        n407 = call <vilib>:"compatOverwrite.vi"("overwrite (F)"=TRUE) -> ("overwrite?"=w1643:T8)
        n408 = Open/Create/Replace File(file path (use dialog)=w1664, error in=w1656, operation (0:open)=w1643) -> (refnum out=w1671:refnum<file>, error out=w1670:errorcluster)  [unwired: 3 in, 1 out]
        n409 = Transpose 2D Array(2D array=w1660) -> (transposed array=w1659:dbl[][])
        n410 = call "4155C Write array to file.vi"("Byte Stream File Refnum"=w1671, "Header"=string[] ["Time /Units", "Ig /A", "Id /A", "Is /A"], "Data Array"=w1659, "error in (no error)"=w1670) -> ("dup refnum"=w1673:refnum<file>, "error out"=w1672:errorcluster)  [unwired: 1 in]
        n411 = Close File(refnum=w1673, error in=w1672) -> (error out=w1662:errorcluster)  [unwired: 1 out]
      }
      frame "samplei" {
        n412 = Number To Decimal String(number=w1769) -> (decimal integer string=w1820:string)  [unwired: 1 in]
        n413 = local read "Sample I - Source/Common"() -> (w1738:u32)
        n414 = local read "Sample I - Probe 4 (Disabled)"() -> (w1741:u32)
        n415 = Concatenate Strings(w1799, "-samplei-" ("Substring"), w1820, w1768, ".txt" ("Substring")) -> (w1818:string)
        n416 = Fract/Exp String To Number(string=w1817) -> (number=w1784:dbl[])  [unwired: 3 in, 1 out]
        n417 = String To Path(string=w1818) -> (path=w1802:path)
        n418 = Index Array(array=w1784, index=4 ("Index")) -> (element=w1778:dbl)
        n419 = Index Array(array=w1784, index=3 ("Index")) -> (element=w1779:dbl)
        n420 = Index Array(array=w1784, index=1 ("Index")) -> (element=w1781:dbl)
        n421 = Index Array(array=w1784, index=0 ("Index")) -> (element=w1782:dbl)
        n422 = local read "Sample I - Drain/Gate"() -> (w1740:u32)
        n423 = Index Array(array=w1784, index=2 ("Index")) -> (element=w1780:dbl)
        n424 = local read "Sample I - Probe 3 (Disabled)"() -> (w1739:u32)
        n425 = call "4155C Config SamplingI Measurements v3.0.vi"("VISA session"=w1823, "Num Points"=w1781, "Sample I - Probe 3 (Disabled)"=w1739, "Display on/off"=TRUE, "Sample I - Source/Common"=w1738, "Sample I - Drain/Gate"=w1740, "Sampling interval"=w1779, "Standby"=w1742, "error in (no error)"=w1822, "Timings"=w1791, "Sample I - Probe 4 (Disabled)"=w1741, "Sample time"=w1780) -> ("dup VISA resource name"=w1825:refnum<visa-resource-name>, "error out"=w1824:errorcluster)  [unwired: 2 in]
        n426 = call "4155C Take SampleI v3.0.vi"("Sample I - Drain/Gate"=w1740, "Emergency Stop"=w1796, "error in (no error)"=w1824, "Idg 2"=w1782, "Vdg compliance 2"=w1778, "VISA resource name in"=w1825) -> ("error out"=w1794:errorcluster, "Idg"=w1827:dbl[], "Vdg"=w1804:dbl[], "VISA Resource Name out"=w1792:refnum<visa-resource-name>, "Is"=w1826:dbl[], "Time"=w1808:dbl[])
        n427 = Insert Into Array(array=dbl[][] [] ("Input Array"), new element=w1808) -> (w1807:dbl[][])  [unwired: 2 in]
        n428 = Insert Into Array(array=w1807, new element=w1804) -> (w1806:dbl[][])  [unwired: 2 in]
        n429 = Insert Into Array(array=w1806, new element=w1827) -> (w1805:dbl[][])  [unwired: 2 in]
        n430 = VISA Write(VISA resource name=w1792, write buffer=":DISP ON" ("write buffer (\"\")"), error in (no error)=w1794) -> (VISA resource name out=w1777:refnum<visa-resource-name>, error out=w1793:errorcluster)  [unwired: 1 out]
        n431 = Insert Into Array(array=w1805, new element=w1826) -> (w1798:dbl[][])  [unwired: 2 in]
        n432 = call <vilib>:"compatOverwrite.vi"("overwrite (F)"=TRUE) -> ("overwrite?"=w1772:T8)
        n433 = Open/Create/Replace File(file path (use dialog)=w1802, error in=w1793, operation (0:open)=w1772) -> (refnum out=w1811:refnum<file>, error out=w1810:errorcluster)  [unwired: 3 in, 1 out]
        n434 = Transpose 2D Array(2D array=w1798) -> (transposed array=w1797:dbl[][])
        n435 = call "4155C Write array to file.vi"("Byte Stream File Refnum"=w1811, "Header"=string[] ["Time /s", "Vdg /V", "Idg /A", "Is /A"], "Data Array"=w1797, "error in (no error)"=w1810) -> ("dup refnum"=w1813:refnum<file>, "error out"=w1812:errorcluster)  [unwired: 1 in]
        n436 = Close File(refnum=w1813, error in=w1812) -> (error out=w1775:errorcluster)  [unwired: 1 out]
        n437 = VISA Write(VISA resource name=w1777, write buffer=";:PAGE:SCON:STAN OFF;:PAGE:CHAN:VSU2:DIS;" ("write buffer (\"\")"), error in (no error)=w1775) -> (VISA resource name out=w1773:refnum<visa-resource-name>, error out=w1774:errorcluster)  [unwired: 1 out]
      }
      frame "#" {
        n438 = VISA Write(VISA resource name=w1860, write buffer=":DISP ON" ("write buffer (\"\")"), error in (no error)=w1859) -> (VISA resource name out=w1858:refnum<visa-resource-name>, error out=w1857:errorcluster)  [unwired: 1 out]
      }
      frame "stressV" {
        n439 = Number To Decimal String(number=w1899) -> (decimal integer string=w1940:string)  [unwired: 1 in]
        n440 = Concatenate Strings(w1924, "-stressV-" ("Substring"), w1940, w1898, ".txt" ("Substring")) -> (w1938:string)
        n441 = Fract/Exp String To Number(string=w1937) -> (number=w1910:dbl[])  [unwired: 3 in, 1 out]
        n442 = local read "Stress V - Source/Common"() -> (w1873:u32)
        n443 = String To Path(string=w1938) -> (path=w1928:path)
        n444 = Index Array(array=w1910, index=3 ("Index")) -> (element=w1907:dbl)
        n445 = Index Array(array=w1910, index=1 ("Index")) -> (element=w1905:dbl)
        n446 = Index Array(array=w1910, index=0 ("Index")) -> (element=w1904:dbl)
        n447 = Index Array(array=w1910, index=4 ("Index")) -> (element=w1909:dbl)
        n448 = Index Array(array=w1910, index=2 ("Index")) -> (element=w1906:dbl)
        n449 = local read "Stress V - Drain"() -> (w1872:u32)
        n450 = local read "Stress V - Gate"() -> (w1871:u32)
        n451 = call "4155C Config V Stress v3.0.vi"("Display on/off"=TRUE, "Stress V - Gate"=w1871, "Stress V - Drain"=w1872, "Stress V - Source/Common"=w1873, "IG compliance"=w1906, "ID compliance"=w1907, "error in (no error)"=w1942, "VG"=w1904, "VD"=w1905, "VISA session"=w1943) -> ("error out"=w1944:errorcluster, "dup VISA resource name"=w1945:refnum<visa-resource-name>)
        n452 = call "4155C Apply Stress.vi"("error in (no error)"=w1944, "Duration"=w1909, "Emergency Stop"=w1923, "VISA resource name in"=w1945) -> ("error out"=w1921:errorcluster, "VISA Resource Name out"=w1919:refnum<visa-resource-name>)
        n453 = VISA Write(VISA resource name=w1919, write buffer=":DISP ON" ("write buffer (\"\")"), error in (no error)=w1921) -> (VISA resource name out=w1918:refnum<visa-resource-name>, error out=w1920:errorcluster)  [unwired: 1 out]
        n454 = call <vilib>:"compatOverwrite.vi"("overwrite (F)"=TRUE) -> ("overwrite?"=w1903:T8)
        n455 = Open/Create/Replace File(file path (use dialog)=w1928, error in=w1920, operation (0:open)=w1903) -> (refnum out=w1931:refnum<file>, error out=w1930:errorcluster)  [unwired: 3 in, 1 out]
        n456 = call "4155C Write array to file.vi"("Byte Stream File Refnum"=w1931, "Header"=string[] ["V stress completed successfully", ""], "error in (no error)"=w1930) -> ("dup refnum"=w1933:refnum<file>, "error out"=w1932:errorcluster)  [unwired: 2 in]
        n457 = Close File(refnum=w1933, error in=w1932) -> (error out=w1926:errorcluster)  [unwired: 1 out]
      }
      frame "stressI" {
        n458 = local read "Stress I - Source/Common"() -> (w1948:u32)
        n459 = Number To Decimal String(number=w1975) -> (decimal integer string=w2012:string)  [unwired: 1 in]
        n460 = Concatenate Strings(w1996, "-stressI-" ("Substring"), w2012, w1974, ".txt" ("Substring")) -> (w2010:string)
        n461 = Fract/Exp String To Number(string=w2009) -> (number=w1984:dbl[])  [unwired: 3 in, 1 out]
        n462 = Index Array(array=w1984, index=1 ("Index")) -> (element=w1980:dbl)
        n463 = Index Array(array=w1984, index=0 ("Index")) -> (element=w1981:dbl)
        n464 = Index Array(array=w1984, index=2 ("Index")) -> (element=w1982:dbl)
        n465 = String To Path(string=w2010) -> (path=w2000:path)
        n466 = local read "Stress I - Drain/Gate"() -> (w1949:u32)
        n467 = call "4155C Config I Stress v3.0.vi"("Stress I - Drain/Gate"=w1949, "Stress I - Source/Common"=w1948, "Display on/off"=TRUE, "error in (no error)"=w2014, "VDG compliance"=w1980, "IDG"=w1981, "VISA session"=w2015) -> ("error out"=w2016:errorcluster, "dup VISA resource name"=w2017:refnum<visa-resource-name>)  [unwired: 1 in]
        n468 = call "4155C Apply Stress.vi"("error in (no error)"=w2016, "Duration"=w1982, "Emergency Stop"=w1995, "VISA resource name in"=w2017) -> ("error out"=w1993:errorcluster, "VISA Resource Name out"=w1991:refnum<visa-resource-name>)
        n469 = VISA Write(VISA resource name=w1991, write buffer=":DISP ON" ("write buffer (\"\")"), error in (no error)=w1993) -> (VISA resource name out=w1990:refnum<visa-resource-name>, error out=w1992:errorcluster)  [unwired: 1 out]
        n470 = call <vilib>:"compatOverwrite.vi"("overwrite (F)"=TRUE) -> ("overwrite?"=w1979:T8)
        n471 = Open/Create/Replace File(file path (use dialog)=w2000, error in=w1992, operation (0:open)=w1979) -> (refnum out=w2003:refnum<file>, error out=w2002:errorcluster)  [unwired: 3 in, 1 out]
        n472 = call "4155C Write array to file.vi"("Byte Stream File Refnum"=w2003, "Header"=string[] ["I stress completed successfully", ""], "error in (no error)"=w2002) -> ("dup refnum"=w2005:refnum<file>, "error out"=w2004:errorcluster)  [unwired: 2 in]
        n473 = Close File(refnum=w2005, error in=w2004) -> (error out=w1998:errorcluster)  [unwired: 1 out]
      }
      frame "vsu2pulse" {
        n474 = Number To Decimal String(number=w2046) -> (decimal integer string=w2081:string)  [unwired: 1 in]
        n475 = Concatenate Strings(w2066, "-vsu2-" ("Substring"), w2081, w2045, ".txt" ("Substring")) -> (w2079:string)
        n476 = Fract/Exp String To Number(string=w2078) -> (number=w2054:dbl[])  [unwired: 3 in, 1 out]
        n477 = String To Path(string=w2079) -> (path=w2070:path)
        n478 = Index Array(array=w2054, index=1 ("Index")) -> (element=w2053:dbl)
        n479 = Index Array(array=w2054, index=0 ("Index")) -> (element=w2051:dbl)
        n480 = local read "VSU2 Stress - Source/Common"() -> (w2020:u32)
        n481 = call "4155C Config VSU2 Stress v3.0.vi"("VISA session"=w2084, "Display on/off"=TRUE, "VSU2"=w2051, "error in (no error)"=w2083, "VSU2 Stress - Source/Common"=w2020) -> ("dup VISA resource name"=w2086:refnum<visa-resource-name>, "error out"=w2085:errorcluster)
        n482 = call "4155C Apply Stress.vi"("error in (no error)"=w2085, "Duration"=w2053, "Emergency Stop"=w2065, "VISA resource name in"=w2086) -> ("error out"=w2063:errorcluster, "VISA Resource Name out"=w2061:refnum<visa-resource-name>)
        n483 = VISA Write(VISA resource name=w2061, write buffer=":DISP ON" ("write buffer (\"\")"), error in (no error)=w2063) -> (VISA resource name out=w2060:refnum<visa-resource-name>, error out=w2062:errorcluster)  [unwired: 1 out]
        n484 = call <vilib>:"compatOverwrite.vi"("overwrite (F)"=TRUE) -> ("overwrite?"=w2050:T8)
        n485 = Open/Create/Replace File(file path (use dialog)=w2070, error in=w2062, operation (0:open)=w2050) -> (refnum out=w2073:refnum<file>, error out=w2072:errorcluster)  [unwired: 3 in, 1 out]
        n486 = call "4155C Write array to file.vi"("Byte Stream File Refnum"=w2073, "Header"=string[] ["VSU2 pulse completed successfully", ""], "error in (no error)"=w2072) -> ("dup refnum"=w2075:refnum<file>, "error out"=w2074:errorcluster)  [unwired: 2 in]
        n487 = Close File(refnum=w2075, error in=w2074) -> (error out=w2068:errorcluster)  [unwired: 1 out]
      }
      frame "sample-fpp" {
        w2094 = 1
        w2160 = string[] ["Time /s", "Id VgVd /A", "Ig VgVd /A", "Vp1 VgVd /V", "Vp2 VgVd /V"] ("Header")
        w2164 = "%d" ("format string")
        # "Y1 = Vp2\nY2 = Vp1"
        # "Add a time offset (elapsed time) to the time axis."
        n488 = local read "Plot sample extrema vs time"() -> (w2103:bool)
        n489 = Number To Decimal String(number=w2152) -> (decimal integer string=w2206:string)  [unwired: 1 in]
        n490 = Fract/Exp String To Number(string=w2203) -> (number=w2191:dbl[])  [unwired: 3 in, 1 out]
        n491 = local read "Plot sample extrema vs time"() -> (w2106:bool)
        n492 = Concatenate Strings(w2197, "-samplefpp-" ("Substring"), w2206, w2151, ".txt" ("Substring")) -> (w2204:string)
        n493 = local read "FPP - Source"() -> (w2130:u32)
        n494 = local read "FPP - Drain"() -> (w2131:u32)
        n495 = local read "FPP - Gate"() -> (w2132:u32)
        n496 = local read "FPP - Probe 1"() -> (w2133:u32)
        n497 = control-ref of="I vs time (Bias Stress)"() -> (w2123:refnum<vi>)
        n498 = String To Path(string=w2204) -> (path=w2172:path)
        n499 = Index Array(array=w2191, index=0 ("Index")) -> (element=w2159:dbl)
        n500 = Index Array(array=w2191, index=1 ("Index")) -> (element=w2158:dbl)
        n501 = local read "Time Units"() -> (w2119:u16)
        n502 = Index Array(array=w2191, index=2 ("Index")) -> (element=w2199:dbl)
        n503 = Index Array(array=w2191, index=3 ("Index")) -> (element=w2189:dbl)
        n504 = Number To Decimal String(number=w2159) -> (decimal integer string=w2180:string)  [unwired: 1 in]
        n505 = local read "FPP - Probe 2"() -> (w2134:u32)
        n506 = call "4155C Config Sampling Measurements FPP v3.0.vi"("VISA session"=w2209, "Gate Compliance"=w2198, "FPP - Source"=w2130, "FPP - Drain"=w2131, "Drain Compliance"=w2207, "error in (no error)"=w2208, "Num Points"=w2199, "Timings"=w2196, "FPP - Gate"=w2132, "FPP - Probe 1"=w2133, "Vg"=w2159, "Vd"=w2158, "Display on/off"=TRUE, "Sample time"=w2189, "FPP - Probe 2"=w2134, "Standby"=w2135) -> ("dup VISA resource name"=w2174:refnum<visa-resource-name>, "error out"=w2173:errorcluster)  [unwired: 2 in]
        n507 = call "4155C Take Sample FPP.vi"("VISA resource name in"=w2174, "error in (no error)"=w2173, "Emergency Stop"=w2175) -> ("Time"=w2122:dbl[], "Vp1"=w2088:dbl[], "VISA Resource Name out"=w2156:refnum<visa-resource-name>, "Ig"=w2100:dbl[], "Id"=w2099:dbl[], "Vp2"=w2087:dbl[], "error out"=w2102:errorcluster)  [unwired: 10 in]
        n508 = Insert Into Array(array=w2128, new element=w2099) -> (w2125:dbl[])  [unwired: 1 in]
        n509 = Insert Into Array(array=w2129, new element=w2100) -> (w2126:dbl[])  [unwired: 1 in]
        n510 = Number To Decimal String(number=w2158) -> (decimal integer string=w2178:string)  [unwired: 1 in]
        n511 = call "4155C Config Chart Colours.vi"("Numeric"=w2094, "XY Graph 2"=w2123) -> ()  [unwired: 6 in]
        n512 = case shown="2" w2119 {
          tunnel: [w2249 w2250 w2253] -> w2121
          tunnel: w2122 -> [w2248 w2250 w2252]
          frame 2 {
            n513 = Divide(x=w2248, y=3600.0) -> (x/y=w2249:dbl[])
          }
          frame 0, Default {
          }
          frame 1 {
            n514 = Divide(x=w2252, y=60.0) -> (x/y=w2253:dbl[])
          }
        }
        n515 = Concatenate Strings("(Vg = " ("Substring"), w2180, "V, Vd = " ("Substring"), w2178, "V)" ("Substring")) -> (w2176:string)
        n516 = Add(x=w2121, y=w2120) -> (x+y=w2093:dbl[])
        n517 = case shown="True" w2103 {
          tunnel: w2093 -> [_ w2212]
          tunnel: [w2210 w2213] -> w2104
          tunnel: w2105 -> [w2210 w2211]
          frame False {
          }
          frame True {
            n518 = Insert Into Array(array=w2211, new element=w2212) -> (w2213:i32[])  [unwired: 1 in]
          }
        }
        n519 = case shown="False" w2106 {
          tunnel: w2099 -> [_ w2240]
          tunnel: w2100 -> [_ w2241]
          tunnel: [w2220 w2231] -> w2101
          tunnel: w2102 -> [w2220 w2235]
          tunnel: w2118 -> [w2219 w2223]
          tunnel: w2117 -> [w2218 w2222]
          tunnel: w2116 -> [w2217 w2243]
          tunnel: w2115 -> [w2216 w2242]
          tunnel: w2114 -> [w2215 w2244]
          tunnel: [w2219 w2223] -> w2112
          tunnel: [w2218 w2222] -> w2111
          tunnel: [w2217 w2233] -> w2110
          tunnel: [w2216 w2229] -> w2109
          tunnel: [w2215 w2234] -> w2108
          tunnel: [w2214 w2228] -> w2107
          tunnel: w2104 -> [_ w2226]
          tunnel: w2113 -> [w2214 w2221]
          frame False {
          }
          frame True {
            w2230 = 1
            # "Number of VAR2 steps is 1."
            # "abs(Ig)"
            # "abs(Id)"
            # "Adjusts graph colors."
            n520 = Absolute Value(x=w2241) -> (abs(x)=w2224:dbl[])
            n521 = Absolute Value(x=w2240) -> (abs(x)=w2225:dbl[])
            n522 = Array Max & Min(array=w2225) -> (max value=w2239:dbl, min value=w2237:dbl)  [unwired: 2 out]
            n523 = Array Max & Min(array=w2224) -> (max value=w2238:dbl, min value=w2236:dbl)  [unwired: 2 out]
            n524 = Insert Into Array(array=w2244, new element=w2224) -> (w2234:dbl[])  [unwired: 1 in]
            n525 = local write "Id max"(w2239) -> ()
            n526 = local write "Id min"(w2237) -> ()
            n527 = local write "Ig max"(w2238) -> ()
            n528 = local write "Ig min"(w2236) -> ()
            n529 = Insert Into Array(array=w2221, new element=w2224) -> (w2228:dbl[])  [unwired: 1 in]
            n530 = Insert Into Array(array=w2243, new element=w2225) -> (w2233:dbl[])  [unwired: 1 in]
            n531 = Insert Into Array(array=w2242, new element=w2225) -> (w2229:dbl[])  [unwired: 1 in]
            n532 = control-ref of="Imax vs time"() -> (w2245:refnum<vi>)
            n533 = call "4155C Config Chart Colours.vi"("Numeric"=w2230, "XY Graph 2"=w2245) -> ()  [unwired: 6 in]
            n534 = call "4155C Split array.vi"("Number of VAR2 steps"=w2230, "Y2 data in"=w2233, "X data in"=w2226, "Y3 data in"=w2234, "error in (no error)"=w2235) -> ("Array of clusters"=w2246:cluster{"Y data in":dbl[], "X data in":dbl[]}[], "error out"=w2232:errorcluster)  [unwired: 2 in]
            n535 = call "4155C Split array.vi"("Number of VAR2 steps"=w2230, "Y2 data in"=w2229, "X data in"=w2226, "Y3 data in"=w2228, "error in (no error)"=w2232) -> ("Array of clusters"=w2227:cluster{"Y data in":dbl[], "X data in":dbl[]}[], "error out"=w2231:errorcluster)  [unwired: 2 in]
            n536 = local write "Imax vs time"(w2246) -> ()
            n537 = local write "Imin vs time"(w2227) -> ()
          }
        }
        n538 = Insert Into Array(array=w2127, new element=w2093) -> (w2095:dbl[])  [unwired: 1 in]
        n539 = call "4155C Split array.vi"("Number of VAR2 steps"=w2094, "Y2 data in"=w2125, "X data in"=w2095, "Y3 data in"=w2126) -> ("Array of clusters"=w2124:cluster{"Y data in":dbl[], "X data in":dbl[]}[])  [unwired: 3 in, 1 out]
        n540 = local write "I vs time (Bias Stress)"(w2124) -> ()
        n541 = Insert Into Array(array=w2092, new element=w2088) -> (w2090:dbl[])  [unwired: 1 in]
        n542 = Insert Into Array(array=w2091, new element=w2087) -> (w2089:dbl[])  [unwired: 1 in]
        n543 = Insert Into Array(array=dbl[][] [] ("Input Array"), new element=w2093) -> (w2187:dbl[][])  [unwired: 2 in]
        n544 = control-ref of="Vp vs time (FPP Bias Stress)"() -> (w2096:refnum<vi>)
        n545 = Insert Into Array(array=w2187, new element=w2099) -> (w2186:dbl[][])  [unwired: 2 in]
        n546 = call <vilib>:"compatOverwrite.vi"("overwrite (F)"=TRUE) -> ("overwrite?"=w2154:T8)
        n547 = Open/Create/Replace File(file path (use dialog)=w2172, error in=w2101, operation (0:open)=w2154) -> (refnum out=w2169:refnum<file>, error out=w2170:errorcluster)  [unwired: 3 in, 1 out]
        n548 = Array To Spreadsheet String(array=w2160, 3:w2164) -> (spreadsheet string=w2166:string)  [unwired: 1 in]
        n549 = call "4155C Split array.vi"("Number of VAR2 steps"=w2094, "Y2 data in"=w2090, "X data in"=w2095, "Y1 data in"=w2089) -> ("Array of clusters"=w2097:cluster{"Y data in":dbl[], "X data in":dbl[]}[])  [unwired: 3 in, 1 out]
        n550 = Insert Into Array(array=w2186, new element=w2100) -> (w2185:dbl[][])  [unwired: 2 in]
        n551 = Search and Replace String(replace all?=TRUE ("replace all? (F)"), input string=w2166, search string="VgVd", replace string=w2176) -> (result string=w2162:string)  [unwired: 4 in, 3 out]
        n552 = local write "Vp vs time (FPP Bias Stress)"(w2097) -> ()
        n553 = Insert Into Array(array=w2185, new element=w2088) -> (w2183:dbl[][])  [unwired: 2 in]
        n554 = call "4155C Config Chart Colours.vi"("Numeric"=w2094, "XY Graph 2"=w2096) -> ()  [unwired: 6 in]
        n555 = Spreadsheet String To Array(format string=w2164, spreadsheet string=w2162, array type (2D Dbl)=w2160) -> (array=w2161:string[])  [unwired: 1 in]
        n556 = Insert Into Array(array=w2183, new element=w2087) -> (w2157:dbl[][])  [unwired: 2 in]
        n557 = Transpose 2D Array(2D array=w2157) -> (transposed array=w2182:dbl[][])
        n558 = call "4155C Write array to file.vi"("Byte Stream File Refnum"=w2169, "Header"=w2161, "Data Array"=w2182, "error in (no error)"=w2170) -> ("dup refnum"=w2167:refnum<file>, "error out"=w2168:errorcluster)  [unwired: 1 in]
        n559 = Close File(refnum=w2167, error in=w2168) -> (error out=w2155:errorcluster)  [unwired: 1 out]
      }
      frame "resample-fpp" {
        w2261 = 1
        w2324 = string[] ["Time /s", "Id VgVd /A", "Ig VgVd /A", "Vp1 VgVd /V", "Vp2 VgVd /V"] ("Header")
        w2328 = "%d" ("format string")
        # "Add a time offset (elapsed time) to the time axis."
        n560 = Number To Decimal String(number=w2312) -> (decimal integer string=w2362:string)  [unwired: 1 in]
        n561 = local read "Plot sample extrema vs time"() -> (w2270:bool)
        n562 = Fract/Exp String To Number(string=w2359) -> (number=w2317:dbl[])  [unwired: 3 in, 1 out]
        n563 = Concatenate Strings(w2355, "-resamplefpp-" ("Substring"), w2362, w2313, ".txt" ("Substring")) -> (w2360:string)
        n564 = local read "Plot sample extrema vs time"() -> (w2273:bool)
        n565 = String To Path(string=w2360) -> (path=w2336:path)
        n566 = local read "Time Units"() -> (w2286:u16)
        n567 = Index Array(array=w2317, index=0 ("Index")) -> (element=w2323:dbl)
        n568 = Index Array(array=w2317, index=1 ("Index")) -> (element=w2322:dbl)
        n569 = Number To Decimal String(number=w2323) -> (decimal integer string=w2342:string)  [unwired: 1 in]
        n570 = call "4155C Take Sample FPP.vi"("VISA resource name in"=w2319, "error in (no error)"=w2318, "Emergency Stop"=w2337) -> ("Time"=w2287:dbl[], "Vp1"=w2255:dbl[], "VISA Resource Name out"=w2321:refnum<visa-resource-name>, "Ig"=w2267:dbl[], "Id"=w2266:dbl[], "Vp2"=w2254:dbl[], "error out"=w2269:errorcluster)  [unwired: 10 in]
        n571 = Insert Into Array(array=w2295, new element=w2266) -> (w2292:dbl[])  [unwired: 1 in]
        n572 = case shown="1" w2286 {
          tunnel: [w2403 w2404 w2407] -> w2289
          tunnel: w2287 -> [w2402 w2404 w2406]
          frame 2 {
            n573 = Divide(x=w2402, y=3600.0) -> (x/y=w2403:dbl[])
          }
          frame 0, Default {
          }
          frame 1 {
            n574 = Divide(x=w2406, y=60.0) -> (x/y=w2407:dbl[])
          }
        }
        n575 = Insert Into Array(array=w2296, new element=w2267) -> (w2293:dbl[])  [unwired: 1 in]
        n576 = Number To Decimal String(number=w2322) -> (decimal integer string=w2340:string)  [unwired: 1 in]
        n577 = Add(x=w2289, y=w2288) -> (x+y=w2260:dbl[])
        n578 = case shown="True" w2270 {
          tunnel: w2260 -> [_ w2366]
          tunnel: [w2364 w2367] -> w2271
          tunnel: w2272 -> [w2364 w2365]
          frame False {
          }
          frame True {
            n579 = Insert Into Array(array=w2365, new element=w2366) -> (w2367:i32[])  [unwired: 1 in]
          }
        }
        n580 = case shown="True" w2273 {
          tunnel: w2266 -> [_ w2393]
          tunnel: w2267 -> [_ w2394]
          tunnel: [w2374 w2384] -> w2268
          tunnel: w2269 -> [w2374 w2388]
          tunnel: w2285 -> [w2373 w2376]
          tunnel: w2283 -> [w2372 w2375]
          tunnel: w2281 -> [w2371 w2396]
          tunnel: w2280 -> [w2370 w2395]
          tunnel: w2279 -> [w2369 w2398]
          tunnel: w2278 -> [w2368 w2397]
          tunnel: [w2373 w2376] -> w2284
          tunnel: [w2372 w2375] -> w2282
          tunnel: [w2371 w2386] -> w2277
          tunnel: [w2370 w2382] -> w2276
          tunnel: [w2369 w2387] -> w2275
          tunnel: [w2368 w2381] -> w2274
          tunnel: w2271 -> [_ w2379]
          frame False {
          }
          frame True {
            w2383 = 1
            # "Number of VAR2 steps is 1."
            # "abs(Ig)"
            # "abs(Id)"
            # "Adjusts graph colors."
            n581 = Absolute Value(x=w2394) -> (abs(x)=w2377:dbl[])
            n582 = Absolute Value(x=w2393) -> (abs(x)=w2378:dbl[])
            n583 = Array Max & Min(array=w2378) -> (max value=w2392:dbl, min value=w2390:dbl)  [unwired: 2 out]
            n584 = Array Max & Min(array=w2377) -> (max value=w2391:dbl, min value=w2389:dbl)  [unwired: 2 out]
            n585 = local write "Id max"(w2392) -> ()
            n586 = local write "Id min"(w2390) -> ()
            n587 = local write "Ig max"(w2391) -> ()
            n588 = local write "Ig min"(w2389) -> ()
            n589 = Insert Into Array(array=w2398, new element=w2377) -> (w2387:dbl[])  [unwired: 1 in]
            n590 = Insert Into Array(array=w2397, new element=w2377) -> (w2381:dbl[])  [unwired: 1 in]
            n591 = Insert Into Array(array=w2396, new element=w2378) -> (w2386:dbl[])  [unwired: 1 in]
            n592 = Insert Into Array(array=w2395, new element=w2378) -> (w2382:dbl[])  [unwired: 1 in]
            n593 = control-ref of="Imax vs time"() -> (w2399:refnum<vi>)
            n594 = call "4155C Config Chart Colours.vi"("Numeric"=w2383, "XY Graph 2"=w2399) -> ()  [unwired: 6 in]
            n595 = call "4155C Split array.vi"("Number of VAR2 steps"=w2383, "Y2 data in"=w2386, "X data in"=w2379, "Y3 data in"=w2387, "error in (no error)"=w2388) -> ("Array of clusters"=w2400:cluster{"Y data in":dbl[], "X data in":dbl[]}[], "error out"=w2385:errorcluster)  [unwired: 2 in]
            n596 = call "4155C Split array.vi"("Number of VAR2 steps"=w2383, "Y2 data in"=w2382, "X data in"=w2379, "Y3 data in"=w2381, "error in (no error)"=w2385) -> ("Array of clusters"=w2380:cluster{"Y data in":dbl[], "X data in":dbl[]}[], "error out"=w2384:errorcluster)  [unwired: 2 in]
            n597 = local write "Imax vs time"(w2400) -> ()
            n598 = local write "Imin vs time"(w2380) -> ()
          }
        }
        n599 = Insert Into Array(array=w2294, new element=w2260) -> (w2262:dbl[])  [unwired: 1 in]
        n600 = Concatenate Strings("(Vg = " ("Substring"), w2342, "V, Vd = " ("Substring"), w2340, "V)" ("Substring")) -> (w2338:string)
        n601 = control-ref of="I vs time (Bias Stress)"() -> (w2290:refnum<vi>)
        n602 = call "4155C Split array.vi"("Number of VAR2 steps"=w2261, "Y2 data in"=w2292, "X data in"=w2262, "Y3 data in"=w2293) -> ("Array of clusters"=w2291:cluster{"Y data in":dbl[], "X data in":dbl[]}[])  [unwired: 3 in, 1 out]
        n603 = local write "I vs time (Bias Stress)"(w2291) -> ()
        n604 = call "4155C Config Chart Colours.vi"("Numeric"=w2261, "XY Graph 2"=w2290) -> ()  [unwired: 6 in]
        n605 = Insert Into Array(array=dbl[][] [] ("Input Array"), new element=w2260) -> (w2349:dbl[][])  [unwired: 2 in]
        n606 = Insert Into Array(array=w2259, new element=w2255) -> (w2257:dbl[])  [unwired: 1 in]
        n607 = Insert Into Array(array=w2349, new element=w2266) -> (w2348:dbl[][])  [unwired: 2 in]
        n608 = call <vilib>:"compatOverwrite.vi"("overwrite (F)"=TRUE) -> ("overwrite?"=w2315:T8)
        n609 = Open/Create/Replace File(file path (use dialog)=w2336, error in=w2268, operation (0:open)=w2315) -> (refnum out=w2333:refnum<file>, error out=w2334:errorcluster)  [unwired: 3 in, 1 out]
        n610 = Array To Spreadsheet String(array=w2324, 3:w2328) -> (spreadsheet string=w2330:string)  [unwired: 1 in]
        n611 = Insert Into Array(array=w2348, new element=w2267) -> (w2347:dbl[][])  [unwired: 2 in]
        n612 = Insert Into Array(array=w2258, new element=w2254) -> (w2256:dbl[])  [unwired: 1 in]
        n613 = Search and Replace String(replace all?=TRUE ("replace all? (F)"), input string=w2330, search string="VgVd", replace string=w2338) -> (result string=w2326:string)  [unwired: 4 in, 3 out]
        n614 = Insert Into Array(array=w2347, new element=w2255) -> (w2345:dbl[][])  [unwired: 2 in]
        n615 = Spreadsheet String To Array(format string=w2328, spreadsheet string=w2326, array type (2D Dbl)=w2324) -> (array=w2325:string[])  [unwired: 1 in]
        n616 = Insert Into Array(array=w2345, new element=w2254) -> (w2316:dbl[][])  [unwired: 2 in]
        n617 = control-ref of="Vp vs time (FPP Bias Stress)"() -> (w2263:refnum<vi>)
        n618 = Transpose 2D Array(2D array=w2316) -> (transposed array=w2344:dbl[][])
        n619 = call "4155C Write array to file.vi"("Byte Stream File Refnum"=w2333, "Header"=w2325, "Data Array"=w2344, "error in (no error)"=w2334) -> ("dup refnum"=w2331:refnum<file>, "error out"=w2332:errorcluster)  [unwired: 1 in]
        n620 = Close File(refnum=w2331, error in=w2332) -> (error out=w2320:errorcluster)  [unwired: 1 out]
        n621 = call "4155C Split array.vi"("Number of VAR2 steps"=w2261, "Y2 data in"=w2257, "X data in"=w2262, "Y1 data in"=w2256) -> ("Array of clusters"=w2264:cluster{"Y data in":dbl[], "X data in":dbl[]}[])  [unwired: 3 in, 1 out]
        n622 = local write "Vp vs time (FPP Bias Stress)"(w2264) -> ()
        n623 = call "4155C Config Chart Colours.vi"("Numeric"=w2261, "XY Graph 2"=w2263) -> ()  [unwired: 6 in]
      }
      frame "serial" {
        n624 = local read "Termination char\n(0xA = '\\n' = LF)\n(0xD = '\\r' = CR)"() -> (w2441:u8)
        n625 = local read "Enable Termination\nChar (T)"() -> (w2442:bool)
        n626 = Index Array(array=w2449, index=0 ("Index")) -> (element=w2448:string)
        n627 = local read "parity"() -> (w2432:u16)
        n628 = local read "Delay before read (ms)"() -> (w2443:u32)
        n629 = local read "byte count"() -> (w2440:u32)
        n630 = local read "VISA resource name"() -> (w2436:refnum<visa-resource-name>)
        n631 = local read "baud rate"() -> (w2435:u32)
        n632 = local read "Serial End Mode for Reads"() -> (w2434:u16)
        n633 = local read "Timeout (ms)"() -> (w2439:u32)
        n634 = local read "data bits"() -> (w2433:u16)
        n635 = local read "stop bits"() -> (w2438:u16)
        n636 = local read "flow control"() -> (w2437:u16)
        n637 = call "Serial write and read v0.5.vi"("Delay before read (ms)"=w2443, "Termination char\n(0xA = '\\n' = LF)\n(0xD = '\\r' = CR)"=w2441, "Enable Termination\nChar (T)"=w2442, "parity"=w2432, "stop bits"=w2438, "string to write"=w2448, "flow control"=w2437, "byte count"=w2440, "Serial Settings:Serial End Mode for Reads"=w2434, "Timeout (ms)"=w2439, "error in (no error)"=w2454, "VISA resource name"=w2436, "baud rate"=w2435, "data bits"=w2433) -> ("Serial port output"=w2444:string, "error out"=w2453:errorcluster)
        n638 = Build Array (concatenate)(w2444, w2445) -> (w2446:string[])
      }
      frame "pump" {
        # "Time array for valve position"
        # "Time array for absolute plunger position"
        # "Valve position"
        # "Absolute plunger position"
        # "Remove \"_\""
        # "Check if hard stop is pressed."
        # "Check if halt is pressed."
        # "Check if pump is idle. Else halt."
        n639 = Index Array(array=w2526, index=0 ("Index")) -> (element=w2503:string)
        n640 = case shown="\"No error\", Default" w2501 {
          tunnel: w2503 -> [w2562 _ w2564 w2565 w2566 w2567 _ _ w2570 w2571 _]
          tunnel: [w2562 "/1H" w2564 w2565 w2566 w2567 "/1H" "/1H" w2570 w2571 "/1H"] -> w2502
          frame "No error", Default {
          }
          frame "Initialization" {
          }
          frame "Invalid command" {
          }
          frame "Invalid operand" {
          }
          frame "Device not initialized" {
          }
          frame "Internal failure" {
          }
          frame "Plunger overload" {
          }
          frame "Valve overload" {
          }
          frame "Plunger move not allowed" {
          }
          frame "A/D converter failure" {
          }
          frame "Command overflow" {
          }
        }
        n641 = local read "Hard stop pump"() -> (w2505:bool)
        n642 = local read "Halt pump"() -> (w2508:bool)
        n643 = local read "Serial End Mode for Reads"() -> (w2514:u16)
        n644 = local read "flow control"() -> (w2517:u16)
        n645 = local read "stop bits"() -> (w2518:u16)
        n646 = local read "parity"() -> (w2512:u16)
        n647 = local read "Delay before read (ms)"() -> (w2523:u32)
        n648 = local read "byte count"() -> (w2520:u32)
        n649 = local read "VISA resource name"() -> (w2516:refnum<visa-resource-name>)
        n650 = local read "baud rate"() -> (w2515:u32)
        n651 = local read "Timeout (ms)"() -> (w2519:u32)
        n652 = local read "Termination char\n(0xA = '\\n' = LF)\n(0xD = '\\r' = CR)"() -> (w2521:u8)
        n653 = local read "Enable Termination\nChar (T)"() -> (w2522:bool)
        n654 = case shown="True" w2508 {
          tunnel: [w2576 "/1H"] -> w2507
          tunnel: w2502 -> [w2576 _]
          frame False {
          }
          frame True {
            n655 = local write "Halt pump"(FALSE) -> ()
          }
        }
        n656 = case shown="True" w2505 {
          tunnel: [w2573 "/1T"] -> w2506
          tunnel: w2507 -> [w2573 _]
          frame False {
          }
          frame True {
            n657 = local write "Hard stop pump"(FALSE) -> ()
          }
        }
        n658 = local read "data bits"() -> (w2513:u16)
        n659 = String Subset(string=w2497, offset (0)=1) -> (substring=w2495:string)  [unwired: 1 in]
        n660 = call "SPM Pump v0.6.vi"("Termination char\n(0xA = '\\n' = LF)\n(0xD = '\\r' = CR)"=w2521, "Enable Termination\nChar (T)"=w2522, "Timeout (ms)"=w2519, "Serial Settings:Serial End Mode for Reads"=w2514, "byte count"=w2520, "Delay before read (ms)"=w2523, "Time <input>"=w2500, "error in (no error)"=w2531, "Serial port input"=w2506, "VISA resource name"=w2516, "parity"=w2512, "baud rate"=w2515, "stop bits"=w2518, "data bits"=w2513, "flow control"=w2517, "Time units <input>"=w2495) -> ("Input command"=w2494:string, "Serial port data"=w2484:string[], "Pump status"=w2490:string, "Valve position"=w2492:i32, "Absolute plunger position"=w2504:i32, "Serial port"=w2499:string, "error out"=w2530:errorcluster)  [unwired: 1 in, 4 out]
        n661 = case shown="\"?6\"" w2494 {
          tunnel: [w2543 w2551 w2557] -> w2511
          tunnel: w2510 -> [w2543 w2550 w2557]
          tunnel: w2504 -> [_ w2549 _]
          tunnel: w2491 -> [w2542 w2548 w2558]
          tunnel: [w2542 w2548 w2560] -> w2493
          tunnel: w2492 -> [_ _ w2559]
          tunnel: w2489 -> [_ w2547 w2555]
          tunnel: w2488 -> [w2541 w2546 w2556]
          tunnel: [w2541 w2545 w2556] -> w2487
          tunnel: [w2540 w2544 w2554] -> w2486
          tunnel: w2485 -> [w2540 w2544 w2553]
          frame "Q", Default {
          }
          frame "?" {
            n662 = Build Array (concatenate)(w2550, w2549) -> (w2551:i32[])
            n663 = Build Array (concatenate)(w2546, w2547) -> (w2545:i32[])
            n664 = call "4155C Split array.vi"("X data in"=w2545, "Y1 data in"=w2551) -> ("Array of clusters"=w2552:cluster{"Y data in":dbl[], "X data in":dbl[]}[])  [unwired: 5 in, 1 out]
            n665 = local write "Absolute plunger position vs time"(w2552) -> ()
          }
          frame "?6" {
            n666 = Build Array (concatenate)(w2558, w2559) -> (w2560:i32[])
            n667 = Build Array (concatenate)(w2553, w2555) -> (w2554:i32[])
            n668 = call "4155C Split array.vi"("X data in"=w2554, "Y1 data in"=w2560) -> ("Array of clusters"=w2561:cluster{"Y data in":dbl[], "X data in":dbl[]}[])  [unwired: 5 in, 1 out]
            n669 = local write "Valve position vs time"(w2561) -> ()
          }
        }
        n670 = Build Array (concatenate)(w2482, w2484) -> (w2483:string[][])
        n671 = Build Array (concatenate)(w2498, w2499) -> (w2524:string[])
      }
      frame "filename" {
        n672 = Index Array(array=w2587, index=0 ("Index")) -> (element=w2586:string)
      }
    }
    "Probe 4 Indicator" <- w73
    "Timings Indicator" <- w72
    n673 = local read "Time Units"() -> (w106:u16)
    n674 = case shown="0" w106 {
      tunnel: ["Time (Seconds)" ("element") "Time (Minutes)" ("element") "Time (Hours)" ("element")] -> w74
      frame 0 {
      }
      frame 1, Default {
      }
      frame 2 {
      }
    }
    n675 = Build Array(w180, w113, w123, w122, w121, w120, w119, w118, w117, w116, w115, w114, w112) -> (w218:dbl[][])
    n676 = Transpose 2D Array(2D array=w218) -> (transposed array=w217:dbl[][])
    n677 = Concatenate Strings(w81, w80, "I-vs-time.txt" ("Suffix (Imax,Imin,Ion,Ioff)")) -> (w228:string)
    n678 = Build Array(w74, "Is max (A)" ("VAR2 Name"), "Is min (A)" ("VAR2 Name"), "Id max (A)" ("VAR2 Name"), "Id min (A)" ("VAR2 Name"), "Ig max (A)" ("VAR2 Name"), "Ig min (A)" ("VAR2 Name"), "Is on (A)" ("VAR2 Name"), "Is off (A)" ("VAR2 Name"), "Id on (A)" ("VAR2 Name"), "Id off (A)" ("VAR2 Name"), "Ig on (A)" ("VAR2 Name"), "Ig off (A)" ("VAR2 Name")) -> (w223:string[])
    n679 = Array To Spreadsheet String(array=w217, 3:"%e" ("format string")) -> (spreadsheet string=w221:string)  [unwired: 1 in]
    n680 = Array To Spreadsheet String(array=w223, 3:"" ("format string")) -> (spreadsheet string=w222:string)  [unwired: 1 in]
    n681 = String To Path(string=w228) -> (path=w227:path)
    n682 = Build Array(w222, w221) -> (w220:string[])
    n683 = Write to Text File(file (use dialog)=w227, text=w220, error in=w177) -> (refnum out=w229:refnum<file>, error out=w219:errorcluster)  [unwired: 1 in, 1 out]
    n684 = Close File(refnum=w229, error in=w219) -> (error out=w161:errorcluster)  [unwired: 1 out]
    n685 = Build Array(w158, w181) -> (w186:i32[][])
    n686 = Build Array(w74, "Absolute plunger position" ("VAR2 Name")) -> (w189:string[])
    n687 = Transpose 2D Array(2D array=w186) -> (transposed array=w179:i32[][])
    n688 = Array To Spreadsheet String(array=w189, 3:"" ("format string")) -> (spreadsheet string=w188:string)  [unwired: 1 in]
    n689 = Array To Spreadsheet String(array=w179, 3:"%e" ("format string")) -> (spreadsheet string=w185:string)  [unwired: 1 in]
    n690 = Build Array(w188, w185) -> (w191:string[])
    n691 = Concatenate Strings(w81, w80, "plunger.txt" ("Suffix (plunger)")) -> (w183:string)
    n692 = String To Path(string=w183) -> (path=w182:path)
    n693 = Write to Text File(file (use dialog)=w182, text=w191, error in=w161) -> (refnum out=w184:refnum<file>, error out=w193:errorcluster)  [unwired: 1 in, 1 out]
    n694 = Close File(refnum=w184, error in=w193) -> (error out=w160:errorcluster)  [unwired: 1 out]
    n695 = Concatenate Strings(w81, w80, "serial-port.txt" ("Suffix (serial port log)")) -> (w199:string)
    n696 = String To Path(string=w199) -> (path=w198:path)
    n697 = Build Array(w74, "Serial port input" ("VAR2 Name"), "Pump status" ("VAR2 Name"), "Serial port output: ") -> (w148:string[])
    n698 = Array To Spreadsheet String(array=w154, 3:"" ("format string")) -> (spreadsheet string=w145:string)  [unwired: 1 in]
    n699 = Array To Spreadsheet String(array=w148, 3:"" ("format string")) -> (spreadsheet string=w146:string)  [unwired: 1 in]
    n700 = Array To Spreadsheet String(array=w153, 3:"" ("format string")) -> (spreadsheet string=w204:string)  [unwired: 1 in]
    n701 = Build Array(w146, w145) -> (w147:string[])
    n702 = Write to Text File(file (use dialog)=w198, text=w147, error in=w160) -> (refnum out=w200:refnum<file>, error out=w201:errorcluster)  [unwired: 1 in, 1 out]
    n703 = local write "Serial port data"(w204) -> ()
    n704 = Close File(refnum=w200, error in=w201) -> (error out=w159:errorcluster)  [unwired: 1 out]
    n705 = Build Array(w157, w163) -> (w169:i32[][])
    n706 = Build Array(w74, "Valve port" ("VAR2 Name")) -> (w172:string[])
    n707 = Transpose 2D Array(2D array=w169) -> (transposed array=w164:i32[][])
    n708 = Array To Spreadsheet String(array=w172, 3:"" ("format string")) -> (spreadsheet string=w171:string)  [unwired: 1 in]
    n709 = Array To Spreadsheet String(array=w164, 3:"%e" ("format string")) -> (spreadsheet string=w168:string)  [unwired: 1 in]
    n710 = Build Array(w171, w168) -> (w174:string[])
    n711 = Concatenate Strings(w81, w80, "valve-port.txt" ("Suffix (valve)")) -> (w166:string)
    n712 = String To Path(string=w166) -> (path=w165:path)
    n713 = Write to Text File(file (use dialog)=w165, text=w174, error in=w159) -> (refnum out=w167:refnum<file>, error out=w176:errorcluster)  [unwired: 1 in, 1 out]
    n714 = Close File(refnum=w167, error in=w176) -> (error out=w82:errorcluster)  [unwired: 1 out]
    n715 = Build Array(w79, w78, w77, w76) -> (w91:dbl[][])
    n716 = Build Array(w74, "Is (A)" ("VAR2 Name"), "Id (A)" ("VAR2 Name"), "Ig (A)" ("VAR2 Name")) -> (w87:string[])
    n717 = Transpose 2D Array(2D array=w91) -> (transposed array=w90:dbl[][])
    n718 = Concatenate Strings(w81, w80, "sample.txt" ("Suffix (Imax,Imin,Ion,Ioff)")) -> (w97:string)
    n719 = Array To Spreadsheet String(array=w87, 3:"" ("format string")) -> (spreadsheet string=w86:string)  [unwired: 1 in]
    n720 = Array To Spreadsheet String(array=w90, 3:"%e" ("format string")) -> (spreadsheet string=w94:string)  [unwired: 1 in]
    n721 = String To Path(string=w97) -> (path=w96:path)
    n722 = Build Array(w86, w94) -> (w93:string[])
    n723 = Write to Text File(file (use dialog)=w96, text=w93, error in=w82) -> (refnum out=w98:refnum<file>, error out=w92:errorcluster)  [unwired: 1 in, 1 out]
    n724 = Close File(refnum=w98, error in=w92) -> (error out=w71:errorcluster)  [unwired: 1 out]
    "error out" <- w71
  }
  "Is max" <- w15
  "Id max" <- w15
  "Ig max" <- w15
  "Imax vs time" <- w2
  "I vs Vg" <- w2
  "Imin vs time" <- w2
  "I vs Vd" <- w2
  "Serial port data" <- "" ("Serial port data")
  "Valve position vs time" <- cluster{"Y data in":dbl[], "X data in":dbl[]}[] [] ("Valve position vs time")
  "Is min" <- w14
  "Id min" <- w14
  "Ig min" <- w14
  "Ion vs time" <- w2
  "Ioff vs time" <- w2
  "Is on" <- w13
  "Id on" <- w13
  "Ig on" <- w13
  "Is off" <- w12
  "Id off" <- w12
  "Ig off" <- w12
  "I vs time (Bias Stress)" <- w2
  "Vp1" <- w3
  "Vp2" <- w3
  "Vp vs time (FPP Bias Stress)" <- w2
